vi "Beampointing.vi"() -> ()   [LabVIEW 2020]
uses:
  Ctrs/beam detection.ctl
  GUI_Beampointing_single_TRA/Ctrs/move.ctl
  Shared/GUI_Template/GUI_master/tcp_new_data_event.ctl
  Shared/GUI_Template/GUI_master/tcp new data cluster.ctl
  Ctrs/thresholds.ctl
  Ctrs/Detection all.ctl
  Ctrs/BP configuration.ctl
  General GUIs/Device GUIs/GUI_Cameras/Controls/Crosshair type def.ctl
  <userlib>/_OpenG.lib/array/array.llb/Filter 1D Array with Scalar (String)__ogtk.vi
  <userlib>/_OpenG.lib/array/array.llb/Sort 1D Array (DBL)__ogtk.vi
  <userlib>/_OpenG.lib/array/array.llb/Reorder 1D Array2 (Variant)__ogtk.vi
  <userlib>/_OpenG.lib/file/file.llb/File Exists - Scalar__ogtk.vi
  <userlib>/_OpenG.lib/array/array.llb/Remove Duplicates from 1D Array (String)__ogtk.vi
  <userlib>/_OpenG.lib/file/file.llb/Strip Path Extension - String__ogtk.vi
  <vilib>/Analysis/NI_AALBase.lvlib
  <vilib>/vision/NI_Vision_Development_Module.lvlib
  <vilib>/Utility/file.llb/Write To Spreadsheet File (string).vi
panel:
  in  "pixel calib":dbl
  out "A2y":dbl
  out "A1y":dbl
  out "A2x":dbl
  out "A1x":dbl
  in  "y'":dbl
  in  "x'":dbl
  in  "y":dbl
  in  "x":dbl
  in  "distance to target plane":dbl
  in  "seperation":dbl
  in  "downstream mirror":dbl
  in  "upstream mirror":dbl
  in  "Coupled Mirror Move":bool
  out "error out":errorcluster
  in  "active CCDs":i32(listbox)
  out "Prev State":string
  out "tcp data event 2":T1
  out "error out 3":errorcluster
  out "cam means":sgl[](array[numeric])
  in  "save path":path=path "W:/BP_DATA"
  out "millisecond timer value":u32
  out "motor refs 3":refnum<vi>[](array[refnum])
  in  "active man refs":cluster{"Ref X":refnum<vi>, "Ref Y":refnum<vi>}
  in  "#imgs avd so far":dbl
  out "Current State":string
  out "CCDs":string[](array[string])
  in  "GUIdevice 12":string
  in  "GUIdevice 11":string
  in  "GUIdevice 10":string
  in  "GUIdevice 9":string
  out "error out 2":errorcluster
  out "Names":string[](array[string])
  out "Box":T2(array[cluster])
  in  "Tab Cams":T3(tab)=enum."Main"
  in  "Cameras and motors":T4(array[cluster]) {"Motor Alias Y" items=["SHG-angle", "compensation-plate-x", "compensation-plate-y", "Stage [um]", "grating angle", "AttenuatorWavelplate", "Delay", "micrometer", "rail position", "Amp3 North", "djjdjd", "drive grating 2 trans", "speed_translation", "speed_rot_grating2", "speed_rot_grating1", "drive grating 2 rot", "drive grating 1 rot", "jet x", "jet y", "jet z", "ESP2_1_blade", "ESP2_2_target rotation", "home1", "ESP2_3_Scatter ST4 Move", "ESP3_3_mode z position", "com", "ESP3_1_Scatter_Mirror_Z", "ESP3_2", "ESP6_1_scatter ST4 x/hor", "ESP6_2_scatter ST4 y/vert", "ESP6_3_scatter mode z", "VISA", "S1C1 x", "S1C1 y", "S1C1 z", "S1C2 x", "S1C2 y", "S1C2 z", "S1C3 x", "S1C3 y", "S1C3 z", "S1C4 x", "S1C4 y", "S1C4 z", "S2C1 x", "S2C1 y", "S2C1 z", "S2C2 x", "S2C2 y", "S2C2 z", "S2C3 x", "S2C3 y", "S2C3 z", "S2C4 x", "S2C4 y", "S2C4 z", "S3C1 x", "S3C1 y", "S3C1 z", "S3C2 x", "S3C2 y", "S3C2 z", "S3C3 x", "S3C3 y", "S3C3 z", "S3C4 x", "S3C4 y", "S3C4 z", "S4C1 x", "S4C1y", "S4C1 z", "S4C2 x", "S4C2 y", "S4C2 z", "S4C3 x", "S4C3 y", "S4C3 z", "S4C4 x", "S4C4 y", "S4C4 z", "S5C1 x", "S5C1 y", "S5C1 z", "S5C2 x", "S5C2 y", "S5C2 z", "S5C3 x", "S5C3 y", "S5C3 z", "S5C4 x", "S5C4 y", "S5C4 z", "S1C1", "S1C2", "S1C3", "S1C4", "S2C1", "S2C2", "S2C3", "S2C4", "S3C1", "S3C2", "S3C3", "S3C4", "S4C1", "S4C2", "S4C3", "S4C4", "S5C1", "S5C2", "S5C3", "S5C4", "Stepsize 1", "Stepsize 2", "Stepsize 3", "VISA", "S1C1", "S1C2", "S1C3", "S1C4", "S2C1", "S2C2", "S2C3", "S2C4", "S3C1", "S3C2", "S3C3", "S3C4", "S4C1", "S4C2", "S4C3", "S4C4", "S5C1", "S5C2", "S5C3", "S5C4", "kHz EC wedge", "Fiber Mode", "XH2", "ND6", "XH4", "d-scan wedge", "EC wedge", "Lanex", "Gentec", "ModeImager", "Magnet", "ProbeDelay", "x position", "y position", "not working", "LaserDiodeX", "LaserDiodeY", "DelayStage (mm)", "Focus_Beam_2 (mm)", "Hex_x", "Hex_y", "Hex_z", "Hex_u", "Hex_v", "Hex_w", "Mode_Image_pos (mm)", "Jet X", "Jet Y", "Jet Z", "Amp2_out_Y", "Amp3_in_X", "Amp2_out_X", "Amp3_in_Y", "Amp4_in_X", "Amp4_in_Y", "Amp4_in_X", "Gaia2_South_Y", "Gaia3_South_X", "Gaia3_South_Y", "Gaia4_South_X", "Gaia4_South_Y", "Amp2_in_X", "Not Working", "Gaia3_North_X", "Gaia3_North_Y", "Gaia4_North_X", "Gaia4_North_Y", "Expanderin_1_X", "Expanderin_1_Y", "weak current", "Amp4_Out_Y", "Gaia2_North_X", "Gaia2_North_Y", "Amp4_out_X", "Amp2_in_Y", "Gaia2_South_X", "Stretcher_Out_X", "Not_Working", "Stretcher_Out_Y", "JetBladeHeight", "Probe far X", "Probe far Y", "Probe near X", "Probe near Y", "Seed in X", "Seed in Y", "Probe delay X", "Probe delay Y", "Seed Lens Z", "SeedWaveplateRot", "Broken", "SeedPrismBroken", "SeedPrismY", "SeedPrismX", "BCaveDiodeM2Horizontal", "BCaveDiodeM2Vertical", "BCaveDiodeM1Vertical", "BCaveDiodeM1Horizontal", "Grating separation (um)", "Grating1 angle", "Grating2 angle", "Jet_X (mm)", "Jet_Y (mm)", "Jet_Z (mm)", "Prepulse stage", "LegendCompressor (mm)", "devport", "ModeImager", "JetBlade", "ProbeDelay", "1", "TubeIn-x", "TubeIn-y", "CompIn-x", "CompIn-y", "stepSize", "Beamline_In-x", "Beamline_In-y", "Beamline_Out-y", "Beamline_Out-x", "OAPin2-x", "OAPin2-y", "Chassi IP", "BCaveIn-X", "BCaveIn-Y", "OAPIn1-X", "OAPIn1-Y", "DMSurface-X", "DMSurface-Y", "testzaber"]; "Motor Alias X" items=["SHG-angle", "compensation-plate-x", "compensation-plate-y", "Stage [um]", "grating angle", "AttenuatorWavelplate", "Delay", "micrometer", "rail position", "Amp3 North", "djjdjd", "drive grating 2 trans", "speed_translation", "speed_rot_grating2", "speed_rot_grating1", "drive grating 2 rot", "drive grating 1 rot", "jet x", "jet y", "jet z", "ESP2_1_blade", "ESP2_2_target rotation", "home1", "ESP2_3_Scatter ST4 Move", "ESP3_3_mode z position", "com", "ESP3_1_Scatter_Mirror_Z", "ESP3_2", "ESP6_1_scatter ST4 x/hor", "ESP6_2_scatter ST4 y/vert", "ESP6_3_scatter mode z", "VISA", "S1C1 x", "S1C1 y", "S1C1 z", "S1C2 x", "S1C2 y", "S1C2 z", "S1C3 x", "S1C3 y", "S1C3 z", "S1C4 x", "S1C4 y", "S1C4 z", "S2C1 x", "S2C1 y", "S2C1 z", "S2C2 x", "S2C2 y", "S2C2 z", "S2C3 x", "S2C3 y", "S2C3 z", "S2C4 x", "S2C4 y", "S2C4 z", "S3C1 x", "S3C1 y", "S3C1 z", "S3C2 x", "S3C2 y", "S3C2 z", "S3C3 x", "S3C3 y", "S3C3 z", "S3C4 x", "S3C4 y", "S3C4 z", "S4C1 x", "S4C1y", "S4C1 z", "S4C2 x", "S4C2 y", "S4C2 z", "S4C3 x", "S4C3 y", "S4C3 z", "S4C4 x", "S4C4 y", "S4C4 z", "S5C1 x", "S5C1 y", "S5C1 z", "S5C2 x", "S5C2 y", "S5C2 z", "S5C3 x", "S5C3 y", "S5C3 z", "S5C4 x", "S5C4 y", "S5C4 z", "S1C1", "S1C2", "S1C3", "S1C4", "S2C1", "S2C2", "S2C3", "S2C4", "S3C1", "S3C2", "S3C3", "S3C4", "S4C1", "S4C2", "S4C3", "S4C4", "S5C1", "S5C2", "S5C3", "S5C4", "Stepsize 1", "Stepsize 2", "Stepsize 3", "VISA", "S1C1", "S1C2", "S1C3", "S1C4", "S2C1", "S2C2", "S2C3", "S2C4", "S3C1", "S3C2", "S3C3", "S3C4", "S4C1", "S4C2", "S4C3", "S4C4", "S5C1", "S5C2", "S5C3", "S5C4", "kHz EC wedge", "Fiber Mode", "XH2", "ND6", "XH4", "d-scan wedge", "EC wedge", "Lanex", "Gentec", "ModeImager", "Magnet", "ProbeDelay", "x position", "y position", "not working", "LaserDiodeX", "LaserDiodeY", "DelayStage (mm)", "Focus_Beam_2 (mm)", "Hex_x", "Hex_y", "Hex_z", "Hex_u", "Hex_v", "Hex_w", "Mode_Image_pos (mm)", "Jet X", "Jet Y", "Jet Z", "Amp2_out_Y", "Amp3_in_X", "Amp2_out_X", "Amp3_in_Y", "Amp4_in_X", "Amp4_in_Y", "Amp4_in_X", "Gaia2_South_Y", "Gaia3_South_X", "Gaia3_South_Y", "Gaia4_South_X", "Gaia4_South_Y", "Amp2_in_X", "Not Working", "Gaia3_North_X", "Gaia3_North_Y", "Gaia4_North_X", "Gaia4_North_Y", "Expanderin_1_X", "Expanderin_1_Y", "weak current", "Amp4_Out_Y", "Gaia2_North_X", "Gaia2_North_Y", "Amp4_out_X", "Amp2_in_Y", "Gaia2_South_X", "Stretcher_Out_X", "Not_Working", "Stretcher_Out_Y", "JetBladeHeight", "Probe far X", "Probe far Y", "Probe near X", "Probe near Y", "Seed in X", "Seed in Y", "Probe delay X", "Probe delay Y", "Seed Lens Z", "SeedWaveplateRot", "Broken", "SeedPrismBroken", "SeedPrismY", "SeedPrismX", "BCaveDiodeM2Horizontal", "BCaveDiodeM2Vertical", "BCaveDiodeM1Vertical", "BCaveDiodeM1Horizontal", "Grating separation (um)", "Grating1 angle", "Grating2 angle", "Jet_X (mm)", "Jet_Y (mm)", "Jet_Z (mm)", "Prepulse stage", "LegendCompressor (mm)", "devport", "ModeImager", "JetBlade", "ProbeDelay", "1", "TubeIn-x", "TubeIn-y", "CompIn-x", "CompIn-y", "stepSize", "Beamline_In-x", "Beamline_In-y", "Beamline_Out-y", "Beamline_Out-x", "OAPin2-x", "OAPin2-y", "Chassi IP", "BCaveIn-X", "BCaveIn-Y", "OAPIn1-X", "OAPIn1-Y", "DMSurface-X", "DMSurface-Y", "testzaber"]}
  in  "tdms root":path=path "c:/BP_DATAsd"
  out "get pos time":u32
  out "config path":string
  out "tolerances (pix)":dbl[](array[numeric])
  in  "device ini":bool
  in  "Exposure:12":dbl=0.095 min=0.0001 max=1.0 format="%#_6f"
  in  "Triggerdelay::12":dbl=0.003 min=0.0 max=0.09 format="%#_6f"
  in  "Exposure::11":dbl=0.095 min=0.0001 max=1.0 format="%#_6f"
  in  "Triggerdelay::11":dbl=0.003 min=0.0 max=0.09 format="%#_6f"
  in  "Exposure::10":dbl=0.095 min=0.0001 max=1.0 format="%#_6f"
  in  "Triggerdelay::10":dbl=0.003 min=0.0 max=0.09 format="%#_6f"
  in  "Exposure::9":dbl=0.095 min=0.0001 max=1.0 format="%#_6f"
  in  "Triggerdelay::9":dbl=0.003 min=0.0 max=0.09 format="%#_6f"
  in  "Trigger::9":bool
  in  "Trigger::10":bool caption="Trigger:10"
  in  "Trigger::11":bool
  in  "Trigger::12":bool
  in  "Target.Y::9":dbl=45.0 caption="T9y" min=0.0 max=2000.0 format="%#_6f"
  in  "Target.X::9":dbl=47.0 caption="Tx9" min=0.0 max=2000.0 format="%#_6f"
  in  "Target.Y::10":dbl=45.0 caption="T10y" min=0.0 max=2000.0 format="%#_6f"
  in  "Target.X::10":dbl=47.0 caption="T10x" min=0.0 max=2000.0 format="%#_6f"
  in  "Target.Y::11":dbl=45.0 caption="T11y" min=0.0 max=2000.0 format="%#_6f"
  in  "Target.X::11":dbl=47.0 caption="T11x" min=0.0 max=2000.0 format="%#_6f"
  in  "Target.Y::12":dbl=45.0 caption="T12y" min=0.0 max=2000.0 format="%#_6f"
  in  "Target.X::12":dbl=47.0 caption="T12x" min=0.0 max=2000.0 format="%#_6f"
  in  "Exposure::8":dbl=0.095 min=3.8e-05 max=1.0 format="%#_6f"
  in  "Triggerdelay::8":dbl=0.003 min=0.0 max=0.09 format="%#_6f"
  in  "Trigger::8":bool
  in  "Target.Y::8":dbl=45.0 caption="T8y" min=0.0 max=2000.0 format="%#_6f"
  in  "Target.X::8":dbl=47.0 caption="T8x" min=0.0 max=2000.0 format="%#_6f"
  in  "Target.Y::7":dbl=45.0 caption="T7x" min=0.0 max=2000.0 format="%#_6f"
  in  "Target.X::7":dbl=47.0 caption="T7y" min=0.0 max=2000.0 format="%#_6f"
  in  "Target.Y::6":dbl=45.0 caption="T6y" min=0.0 max=2000.0 format="%#_6f"
  in  "Target.X::6":dbl=47.0 caption="T6x" min=0.0 max=2000.0 format="%#_6f"
  in  "Target.Y::5":dbl=45.0 caption="T5y" min=0.0 max=2000.0 format="%#_6f"
  in  "Target.X::5":dbl=47.0 caption="T5x" min=0.0 max=2000.0 format="%#_6f"
  in  "Target.Y::4":dbl=45.0 caption="T4y" min=0.0 max=2000.0 format="%#_6f"
  in  "Target.X::4":dbl=47.0 caption="T4x" min=0.0 max=2000.0 format="%#_6f"
  in  "Target.Y::3":dbl=163.0 caption="T3y" min=0.0 max=2000.0 format="%#_6f"
  in  "Target.X::3":dbl=152.0 caption="T3x" min=0.0 max=2000.0 format="%#_6f"
  in  "Target.Y::2":dbl=74.0 caption="T2y" min=0.0 max=2000.0 format="%#_6f"
  in  "Target.X::2":dbl=75.0 caption="T2x" min=0.0 max=2000.0 format="%#_6f"
  in  "Target.Y::1":dbl=61.0 caption="T1y" min=0.0 max=2000.0 format="%#_6f"
  in  "Target.X::1":dbl=77.0 caption="T1x" min=0.0 max=2000.0 format="%#_6f"
  in  "Exposure::7":dbl=0.095 min=3.8e-05 max=1.0 format="%#_6f"
  in  "Triggerdelay::7":dbl=0.003 min=0.0 max=0.09 format="%#_6f"
  in  "Trigger::7":bool
  in  "Exposure::6":dbl=0.095 min=0.0001 max=1.0 format="%#_6f"
  in  "Triggerdelay::6":dbl=0.003 min=1.0 max=900000.0 format="%#_6f"
  in  "Trigger::6":bool
  in  "Exposure::5":dbl=0.095 min=0.0001 max=1.0 format="%#_6f"
  in  "Triggerdelay::5":dbl=0.003 min=0.0 max=100000.0 format="%#_6f"
  in  "Trigger::5":bool
  in  "Exposure::4":dbl=0.095 min=10.0 max=1000000.0 format="%#_6f"
  in  "Triggerdelay::4":dbl=0.003 min=10.0 max=1000000.0 format="%#_6f"
  in  "Trigger::4":bool
  in  "Exposure::3":dbl=0.095 min=5e-05 max=1.0 format="%#_6f"
  in  "Triggerdelay::3":dbl=0.003 min=10.0 max=500000.0 format="%#_6f"
  in  "Trigger::3":bool
  in  "Exposure::2":dbl=0.095 min=1e-05 max=1.0 format="%#_6f"
  in  "Triggerdelay::2":dbl=0.003 min=10.0 max=100000.0 format="%#_6f"
  in  "Trigger::2":bool
  out "image::1":T5(plugin-control) caption="UC_TubeIn"
  out "image::2":T5(plugin-control) caption="UC_GratingMode"
  out "image::3":T5(plugin-control) caption="UC_DMSurface"
  out "image::4":T5(plugin-control) caption="UC_BCaveIn"
  out "image::5":T5(plugin-control) caption="UC_OAPin1"
  out "image::6":T5(plugin-control) caption="UC_OAPin2"
  out "image::7":T5(plugin-control)
  out "image::8":T5(plugin-control)
  in  "Exposure::1":dbl=0.095 min=50.0 max=500000.0 format="%#_6f"
  in  "Triggerdelay::1":dbl=0.003 min=0.01 max=999000.0 format="%#_6f"
  in  "Trigger::1":bool
  in  "UDP error message":string
  out "required Y":bool[](array[boolean])
  out "required X":bool[](array[boolean])
  out "detected":bool[](array[boolean])
  out "name array":string[](array[string])
  out "image::9":T5(plugin-control)
  out "image::10":T5(plugin-control)
  out "image::11":T5(plugin-control)
  out "image::12":T5(plugin-control)
  out "CCD 1":cluster{timestamp[], dbl[]}[](graph)
  in  "History Size":i32=500
  out "History Index":i32
  in  "Cam# history":i32
  out "Moving X":string
  out "Moving Y":string
  in  "centroidy::4":dbl=45.0 caption="T4y" min=0.0 max=0.0 format="%#_6f"
  in  "centroidx::4":dbl=47.0 caption="T4x" min=0.0 max=0.0 format="%#_6f"
  in  "centroidy::3":dbl=163.0 caption="T3y" min=0.0 max=0.0 format="%#_6f"
  in  "centroidx::3":dbl=152.0 caption="T3x" min=0.0 max=0.0 format="%#_6f"
  in  "centroidy::2":dbl=74.0 caption="T2y" min=0.0 max=0.0 format="%#_6f"
  in  "centroidx::2":dbl=75.0 caption="T2x" min=0.0 max=0.0 format="%#_6f"
  in  "centroidy::1":dbl=61.0 caption="T1y" min=0.0 max=0.0 format="%#_6f"
  in  "centroidx::1":dbl=77.0 caption="T1x" min=0.0 max=0.0 format="%#_6f"
  in  "centroidy::8":dbl=45.0 caption="T8y" min=0.0 max=0.0 format="%#_6f"
  in  "centroidx::8":dbl=47.0 caption="T8x" min=0.0 max=0.0 format="%#_6f"
  in  "centroidy::7":dbl=45.0 caption="T7x" min=0.0 max=0.0 format="%#_6f"
  in  "centroidx::7":dbl=47.0 caption="T7y" min=0.0 max=0.0 format="%#_6f"
  in  "centroidy::6":dbl=45.0 caption="T6y" min=0.0 max=0.0 format="%#_6f"
  in  "centroidx::6":dbl=47.0 caption="T6x" min=0.0 max=0.0 format="%#_6f"
  in  "centroidy::5":dbl=45.0 caption="T5y" min=0.0 max=0.0 format="%#_6f"
  in  "centroidx::5":dbl=47.0 caption="T5x" min=0.0 max=0.0 format="%#_6f"
  in  "centroidy::12":dbl=45.0 caption="T12y" min=0.0 max=2000.0 format="%#_6f"
  in  "centroidx::12":dbl=47.0 caption="T12x" min=0.0 max=2000.0 format="%#_6f"
  in  "centroidy::11":dbl=45.0 caption="T11y" min=0.0 max=2000.0 format="%#_6f"
  in  "centroidx::11":dbl=47.0 caption="T11x" min=0.0 max=2000.0 format="%#_6f"
  in  "centroidy::10":dbl=45.0 caption="T10y" min=0.0 max=2000.0 format="%#_6f"
  in  "centroidx::10":dbl=47.0 caption="T10x" min=0.0 max=2000.0 format="%#_6f"
  in  "centroidy::9":dbl=45.0 caption="T9y" min=0.0 max=2000.0 format="%#_6f"
  in  "centroidx::9":dbl=47.0 caption="Tx9" min=0.0 max=2000.0 format="%#_6f"
  out "active ccd particles":T6(array[cluster])
  in  "Speedmode":dbl=5.0 min=1.0 max=20.0
  out "all UDP in motor config good":bool
  in  "Feedback Global":bool
  in  "GUIdevice 8":string
  in  "Tab Control":T7(tab)
  in  "alarms":bool
  in  "new tdms":bool
  in  "Save Stats":bool
  in  "Save Config":bool
  in  "Load Config":bool
  in  "update speed [ms]":i32=2000 min=1000 max=10000
  in  "img to avg":i32=15 min=3 max=200
  in  "Reset History":bool
  in  "autodetect":bool
  in  "Detection Rate":dbl=0.9 min=0.001 max=1.0
  in  "Center":bool
  in  "Align":bool
  in  "average centroid":bool
  in  "clear error":bool
  in  "thresholds":T8
  in  "beam detection para":T9={"Filter"=1, "Filter Para"={"X Size"=5, "Y Size"=5, "% Tolerance"=1}, "detection method"=4, "Particle filtering"=[{"Measurement Parameter"=35, "Range Lower Value"=0.0, "Range Upper Value"=500.0, "Range"=FALSE, "Measurement Type"=FALSE}], "Remove small Objects"=TRUE, "Restrict to round Objects"=FALSE, "Use Cam COM"=FALSE} {"Particle filtering"."Measurement Parameter" items=["Center of Mass X", "Center of Mass Y", "First Pixel X", "First Pixel Y", "Bounding Rect Left", "Bounding Rect Top", "Bounding Rect Right", "Bounding Rect Bottom", "Max Feret Diameter Start X", "Max Feret Diameter Start Y", "Max Feret Diameter End X", "Max Feret Diameter End Y", "Max Horiz. Segment Length Left", "Max Horiz. Segment Length Right", "Max Horiz. Segment Length Row", "-", "Bounding Rect Width", "Bounding Rect Height", "Bounding Rect Diagonal", "Perimeter", "Convex Hull Perimeter", "Holes' Perimeter", "Max Feret Diameter", "Equivalent Ellipse Major Axis", "Equivalent Ellipse Minor Axis", "Equivalent Ellipse Minor Axis (Feret)", "Equivalent Rect Long Side", "Equivalent Rect Short Side", "Equivalent Rect Diagonal", "Equivalent Rect Short Side (Feret)", "Average Horiz. Segment Length", "Average Vert. Segment Length", "Hydraulic Radius", "Waddel Disk Diameter", "-", "Area", "Holes' Area", "Particle & Holes' Area", "Convex Hull Area", "Image Area", "-", "Number of Holes", "Number of Horiz. Segments", "Number of Vert. Segments", "-", "Orientation", "Max Feret Diameter Orientation", "-", "% Area/Image Area", "% Area/(Particle & Holes' Area)", "Ratio of Equivalent Ellipse Axes", "Ratio of Equivalent Rect Sides", "-", "Elongation Factor", "Compactness Factor", "Heywood Circularity Factor", "Type Factor", "-", "Sum X", "Sum Y", "Sum XX", "Sum XY", "Sum YY", "Sum XXX", "Sum XXY", "Sum XYY", "Sum YYY", "-", "Moment of Inertia XX", "Moment of Inertia XY", "Moment of Inertia YY", "Moment of Inertia XXX", "Moment of Inertia XXY", "Moment of Inertia XYY", "Moment of Inertia YYY", "Norm. Moment of Inertia XX", "Norm. Moment of Inertia XY", "Norm. Moment of Inertia YY", "Norm. Moment of Inertia XXX", "Norm. Moment of Inertia XXY", "Norm. Moment of Inertia XYY", "Norm. Moment of Inertia YYY", "Hu Moment 1", "Hu Moment 2", "Hu Moment 3", "Hu Moment 4", "Hu Moment 5", "Hu Moment 6", "Hu Moment 7"]; "Particle filtering"."Range Lower Value" format="%.2f"; "Particle filtering"."Range Upper Value" format="%.2f"; "detection method" items=["clustering", "entropy", "metric", "moments", "inter-class variance"]; "Filter" items=["No Filter", "Median Filter", "Low Pass Filter"]}
  out "Active CCD":string
  in  "move config":T11={"Tolerance [%]"=0.1, "Stepsize"=0.0001, "Invert Direction X"=FALSE, "Invert Direction Y"=TRUE, "enable feedback"=FALSE, "Set Centriod Target"=FALSE, "xCal"=0.0001, "xCal neg"=0.0001, "yCal"=0.0001, "yCal neg"=0.0001}
  in  "Position 2":dbl=0.001 caption="Stepsize" min=0.0 max=999999.0 format="%_6f"
  in  "Position 1":dbl=0.001 caption="Stepsize" min=0.0 max=999999.0 format="%_6f"
  in  "Right":bool caption="RelativeMove.Axis 1.CCW::1"
  in  "Left":bool caption="RelativeMove.Axis 1.CW::1"
  in  "Down":bool caption="RelativeMove.Axis. 2.CCW::1"
  in  "Up":bool caption="RelativeMove.Axis 2.CW::1"
  in  "StepSize":dbl=0.01 caption="Stepsize" min=0.0 max=1.0 step=0.001 format="%#_6p"
  in  "Time":timestamp[][](array[timestamp])
  in  "Offset X":dbl[][](array[numeric])
  in  "Mean Centroid X":dbl[][](array[numeric])
  in  "GUIdevice 7":string
  in  "GUIdevice 6":string
  in  "GUIdevice 5":string
  in  "GUIdevice 4":string
  in  "GUIdevice 3":string="TargetCam10Hz_Diode"
  in  "GUIdevice 2":string="StagingM1Far"
  in  "insert tag":bool=TRUE
  in  "stop":bool
  in  "GUIdevice 1":string="StagingM1Near"
  out "error IO 2":errorcluster
  # "code in progess for coupled mirror move: please don't delete (Sam)"
  # "Motor axes must have aliases"
  # "Save config after changing cams/motors"
  # "max"
  # "When running for the first time\nCancel the load configuration\nSet the Camera and motors in the config tab\nSave the configuration\nLoad the configuration\nConfigure the detection and feedback for each camera\nSave the configuration\n\nTips\nIn detection, you can exclude or include particles. Typically, include based on the area of the particle.\nYou can either use the particle centroid, or the center of mass calculated in the camera\nFor the case of camera COM, it will only use it if it is in the bounding box of the detected particle.\nA calibration is critical for good performance. Use MC to perform a motor scan and perform a linear fit of COM vs motor position in x and y. Put the gradients into xCal and yCal.\nStep size in move config no longer used.\nFor motors (like LTAs), set the backlash and set it to default in MC. Backlash amount is retrieved from a positive and negative motor scan, and reading the position distance between the lines of the graph of COM vs motor position.\nUnder system tab, update speed must be > than slowest camera update. Otherwise program will find the slow cam/s not having a new image, and it will perform a new configuration."
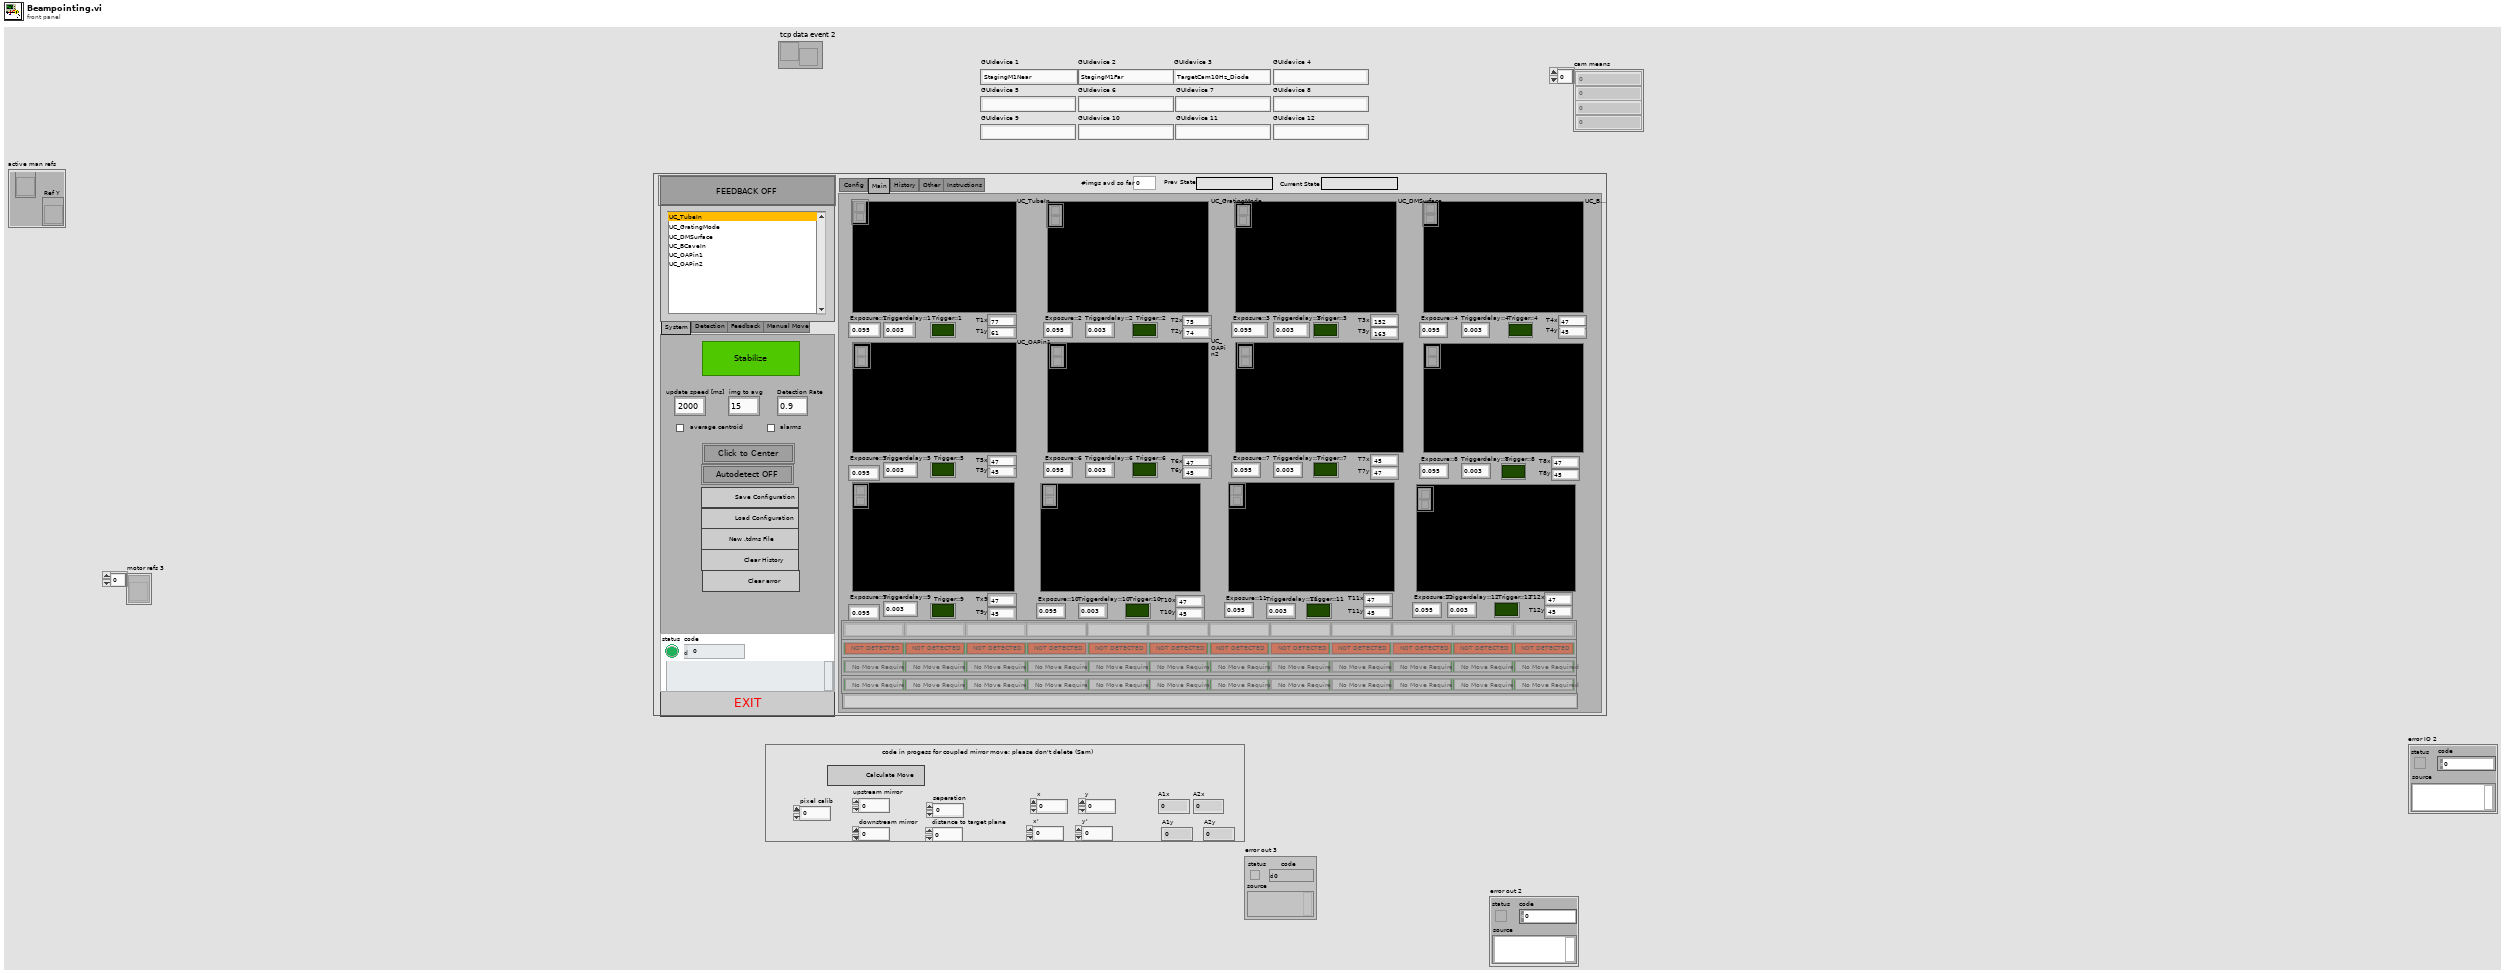
[diagram p1: front panel]
types:
  T1 = typedef "tcp_new_data_event.ctl" = refnum<user-event>
  T2 = cluster{"Left":dbl, "Top":dbl, "Right":dbl, "Bottom":dbl}[]
  T3 = enum32{"Config ", "Main", "History", "Other", "Instructions"}
  T4 = cluster{"Camera":string, "Motor Alias X":u16, "Motor Alias Y":u16}[]
  T5 = typedef "IMAQ Image.ctl" = refnum<image>
  T6 = cluster{"Area":dbl, "Number of Holes":dbl, "Bounding Rect":cluster{"Left":dbl, "Top":dbl, "Right":dbl, "Bottom":dbl}, "Center of Mass":cluster{"X":dbl, "Y":dbl}, "Orientation":dbl, "Dimensions":cluster{"Width":dbl, "Height":dbl}}[]
  T7 = enum32{"System", "Detection", "Feedback", "Manual Move"}
  T8 = typedef "thresholds.ctl" = cluster{"Lower value":sgl, "Upper value":sgl}
  T9 = typedef "beam detection.ctl" = cluster{"Filter":u16, "Filter Para":cluster{"X Size":i32, "Y Size":i32, "% Tolerance":i32}, "detection method":i32, "Particle filtering":cluster{"Measurement Parameter":T10, "Range Lower Value":dbl, "Range Upper Value":dbl, "Range":bool, "Measurement Type":bool}[], "Remove small Objects":bool, "Restrict to round Objects":bool, "Use Cam COM":bool}
  T10 = typedef "Particle Parameters" = i32
  T11 = typedef "move.ctl" = cluster{"Tolerance [%]":dbl, "Stepsize":dbl, "Invert Direction X":bool, "Invert Direction Y":bool, "enable feedback":bool, "Set Centriod Target":bool, "xCal":dbl, "xCal neg":dbl, "yCal":dbl, "yCal neg":dbl}
  T12 = cluster{"Target.X::1":refnum<vi>, "Target.Y::1":refnum<vi>}
  T13 = cluster{"Target.X::2":refnum<vi>, "Target.Y::2":refnum<vi>}
  T14 = cluster{"Target.X::3":refnum<vi>, "Target.Y::3":refnum<vi>}
  T15 = cluster{"Target.X::4":refnum<vi>, "Target.Y::4":refnum<vi>}
  T16 = cluster{"Target.X::5":refnum<vi>, "Target.Y::5":refnum<vi>}
  T17 = cluster{"Target.X::6":refnum<vi>, "Target.Y::6":refnum<vi>}
  T18 = cluster{"Target.X::7":refnum<vi>, "Target.Y::7":refnum<vi>}
  T19 = cluster{"Target.X::8":refnum<vi>, "Target.Y::8":refnum<vi>}
  T20 = cluster{"Target.X::12":refnum<vi>, "Target.Y::12":refnum<vi>}
  T21 = cluster{"Target.X::9":refnum<vi>, "Target.Y::9":refnum<vi>}
  T22 = cluster{"Target.X::10":refnum<vi>, "Target.Y::10":refnum<vi>}
  T23 = cluster{"Target.X::11":refnum<vi>, "Target.Y::11":refnum<vi>}
  T24 = cluster{"Target.X::12":refnum<vi>, "Target.Y::12":refnum<vi>}[]
  T25 = enum32{"invalid app kind", "Development System", "Run Time System", "Student Edition", "Embedded LabVIEW", "Evaluation", "Custom"}
  T26 = enum32{"Invalid", "Standard", "Closed", "Hidden", "Minimized", "Maximized"}
  T27 = typedef "BP configuration.ctl" = cluster{"Camera names":string[], "Motor aliases x":string[], "Motor aliases y":string[], "detection para":T9[], "thresholds":cluster{"Lower value":sgl, "Upper value":sgl}[], "move properties":T11[], "tdms root":path}
  T28 = typedef "tcp new data cluster.ctl" = cluster{"EventEnum":enum16{"new data", "connection status update"}, "Device name":string}
  T29 = enum16{"open", "replace", "create", "open or create", "replace or create", "replace or create with confirmation"}
  T30 = enum8{"Enabled", "Disabled", "Disabled and Grayed Out"}
  T31 = enum16{"open", "open or create", "create or replace", "create", "open (read-only)"}
  T32 = typedef "Detection all.ctl" = cluster{"detection para":T9[], "thresholds":cluster{"Lower value":sgl, "Upper value":sgl}[], "Centroid X":dbl[][], "Centroid Y":dbl[][], "Size":dbl[][], "Centroid refs":cluster{"centroidx::12":refnum<vi>, "centroidy::12":refnum<vi>}[], "img to avg":i32}
  T33 = cluster{"detection para":T9[], "thresholds":cluster{"Lower value":sgl, "Upper value":sgl}[], "Centroid X":dbl[][], "Centroid Y":dbl[][], "Size":dbl[][], "Centroid refs":cluster{"centroidx::12":refnum<vi>, "centroidy::12":refnum<vi>}[], "img to avg":i32}
  T34 = cluster{"Area":dbl, "Number of Holes":dbl, "Bounding Rect":cluster{"Left":dbl, "Top":dbl, "Right":dbl, "Bottom":dbl}, "Center of Mass":cluster{"X":dbl, "Y":dbl}, "Orientation":dbl, "Dimensions":cluster{"Width":dbl, "Height":dbl}}[][]
  T35 = cluster{"Core":cluster{"Current VI Reference":refnum<vi>, "Close Panel on Exit?":bool}, "Detection":T32, "Mean Centroid X":dbl[][], "Mean Centroid Y":dbl[][], "Offset X":dbl[][], "Offset Y":dbl[][], "Offset X stats ":dbl[][], "Offset Y stats ":dbl[][], "Mean Size":dbl[][], "Time":timestamp[][], "move properties":T11[], "active axis refs 2":cluster{"Ref X":refnum<vi>, "Ref Y":refnum<vi>}[], "active ccd":i32, "Feedback global":bool, "Motor X":dbl[][], "Motor Y":dbl[][], "active cams":string[], "tdms ref":refnum<k34>, "active man refs":cluster{"Ref X":refnum<vi>, "Ref Y":refnum<vi>}, "detected":bool[], "speedmode X":bool[], "speedmode Y":bool[], "steps speed X":dbl[], "steps speed Y":dbl[], "Supergui":cluster{"STOP queue":refnum<queue>, "SuperGUI ref":refnum<vi>}, "dev var alias arrays":cluster{"dev variable alias":string[][], "dev variable alias Motors X":string[][], "dev variable alias Motors Y":string[][]}, "Motor positions":cluster{"Positions x":dbl[], "Positions y":dbl[]}, "Config loaded":bool}
  T36 = cluster{"Positions x":dbl[], "Positions y":dbl[]}
  T37 = cluster{"dev variable alias":string[][], "dev variable alias Motors X":string[][], "dev variable alias Motors Y":string[][]}
  T38 = cluster{"Ref X":refnum<vi>, "Ref Y":refnum<vi>}[]
  T39 = cluster{"STOP queue":refnum<queue>, "SuperGUI ref":refnum<vi>}
  T40 = cluster{"Current VI Reference":refnum<vi>, "Close Panel on Exit?":bool}
  T41 = cluster{"centroidx::1":refnum<vi>, "centroidy::1":refnum<vi>}
  T42 = cluster{"centroidx::2":refnum<vi>, "centroidy::2":refnum<vi>}
  T43 = cluster{"centroidx::3":refnum<vi>, "centroidy::3":refnum<vi>}
  T44 = cluster{"centroidx::4":refnum<vi>, "centroidy::4":refnum<vi>}
  T45 = cluster{"centroidx::5":refnum<vi>, "centroidy::5":refnum<vi>}
  T46 = cluster{"centroidx::6":refnum<vi>, "centroidy::6":refnum<vi>}
  T47 = cluster{"centroidx::7":refnum<vi>, "centroidy::7":refnum<vi>}
  T48 = cluster{"centroidx::8":refnum<vi>, "centroidy::8":refnum<vi>}
  T49 = cluster{"centroidx::12":refnum<vi>, "centroidy::12":refnum<vi>}
  T50 = cluster{"centroidx::9":refnum<vi>, "centroidy::9":refnum<vi>}
  T51 = cluster{"centroidx::10":refnum<vi>, "centroidy::10":refnum<vi>}
  T52 = cluster{"centroidx::11":refnum<vi>, "centroidy::11":refnum<vi>}
  T53 = cluster{"centroidx::12":refnum<vi>, "centroidy::12":refnum<vi>}[]
  T54 = cluster{"Camera":string, "Motor Alias X":u16, "Motor Alias Y":u16}
  T55 = typedef "Image Type" = u32
  T56 = cluster{"appended array":timestamp[], "appended array":dbl[]}
  T57 = cluster{"appended array":timestamp[], "appended array":dbl[]}[]
  T58 = typedef "Crosshair type def.ctl" = cluster{"Draw":bool, "Target":cluster{"x":dbl, "y":dbl}, "Size":cluster{"x":dbl, "y":dbl}, "Angle":dbl, "Color":u32, "Thickness":u8, "CrosshairLabel":string}
  T59 = cluster{"Left":i32, "Top":i32, "Right":i32, "Bottom":i32}
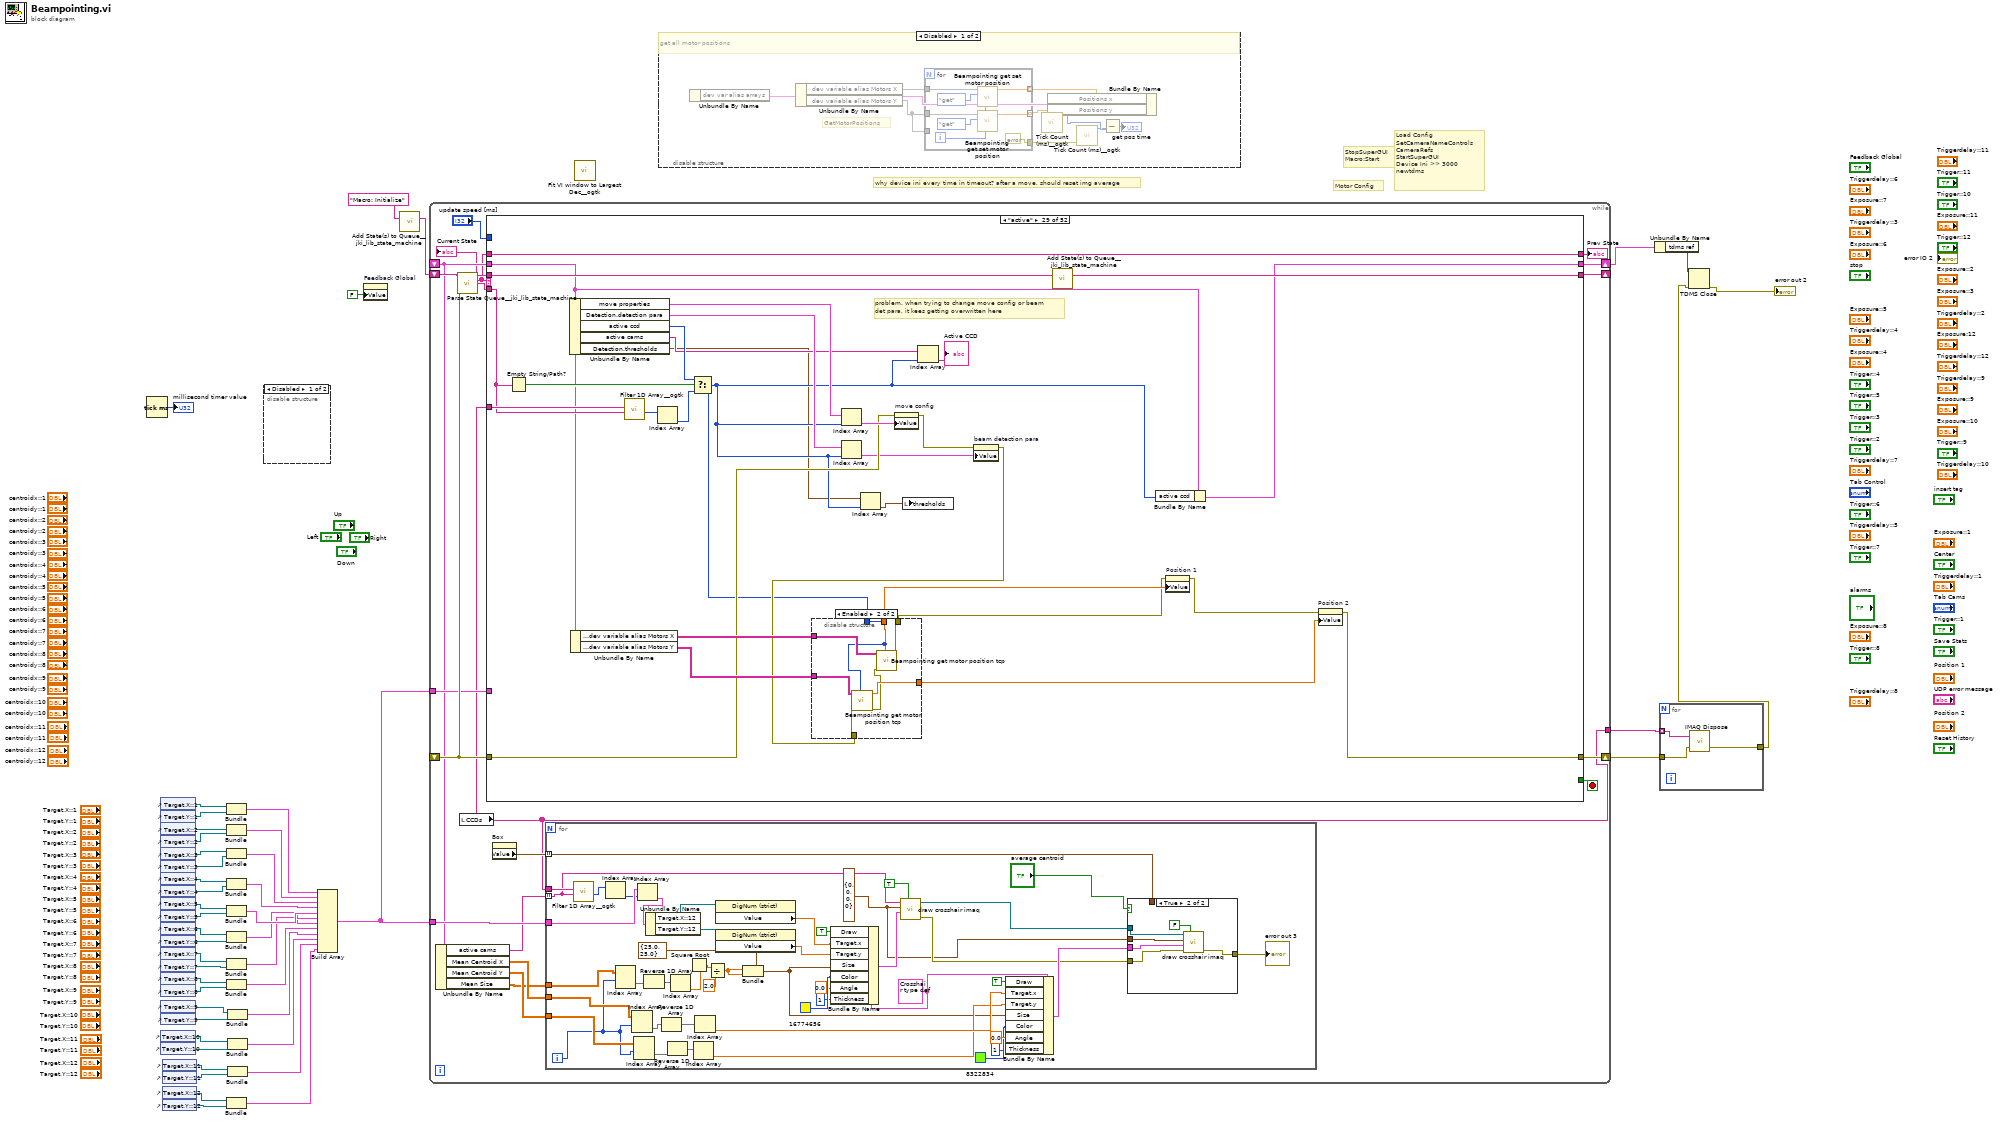
[diagram p0: block diagram]
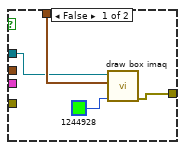
[diagram p4: hidden frame]
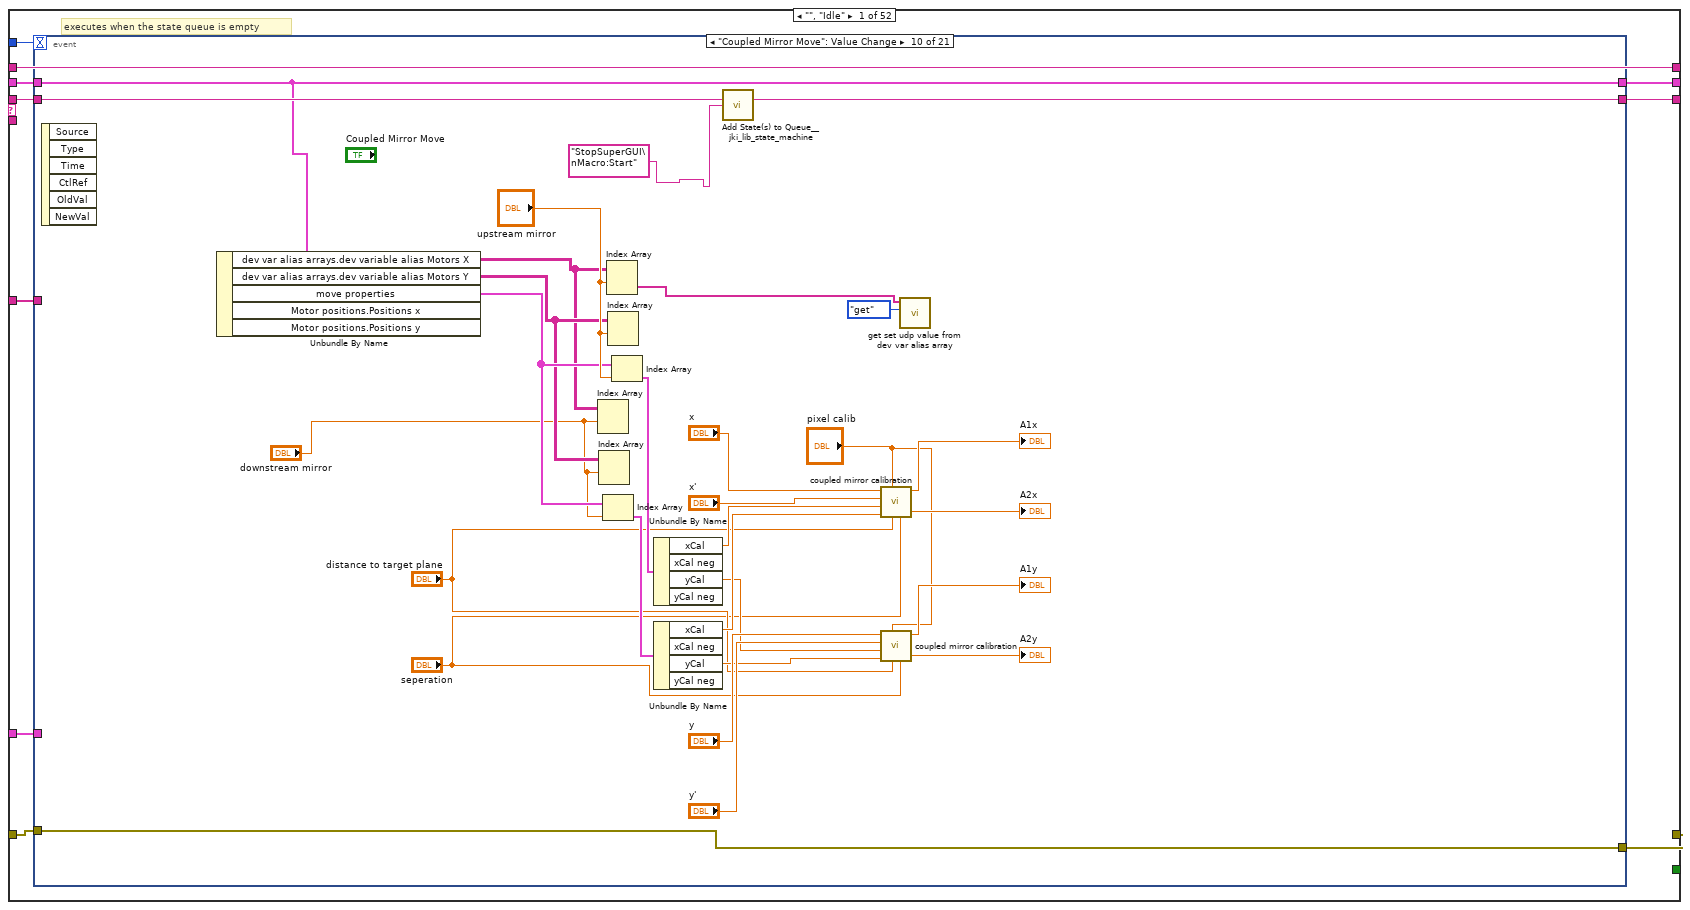
[diagram p5: hidden frame]
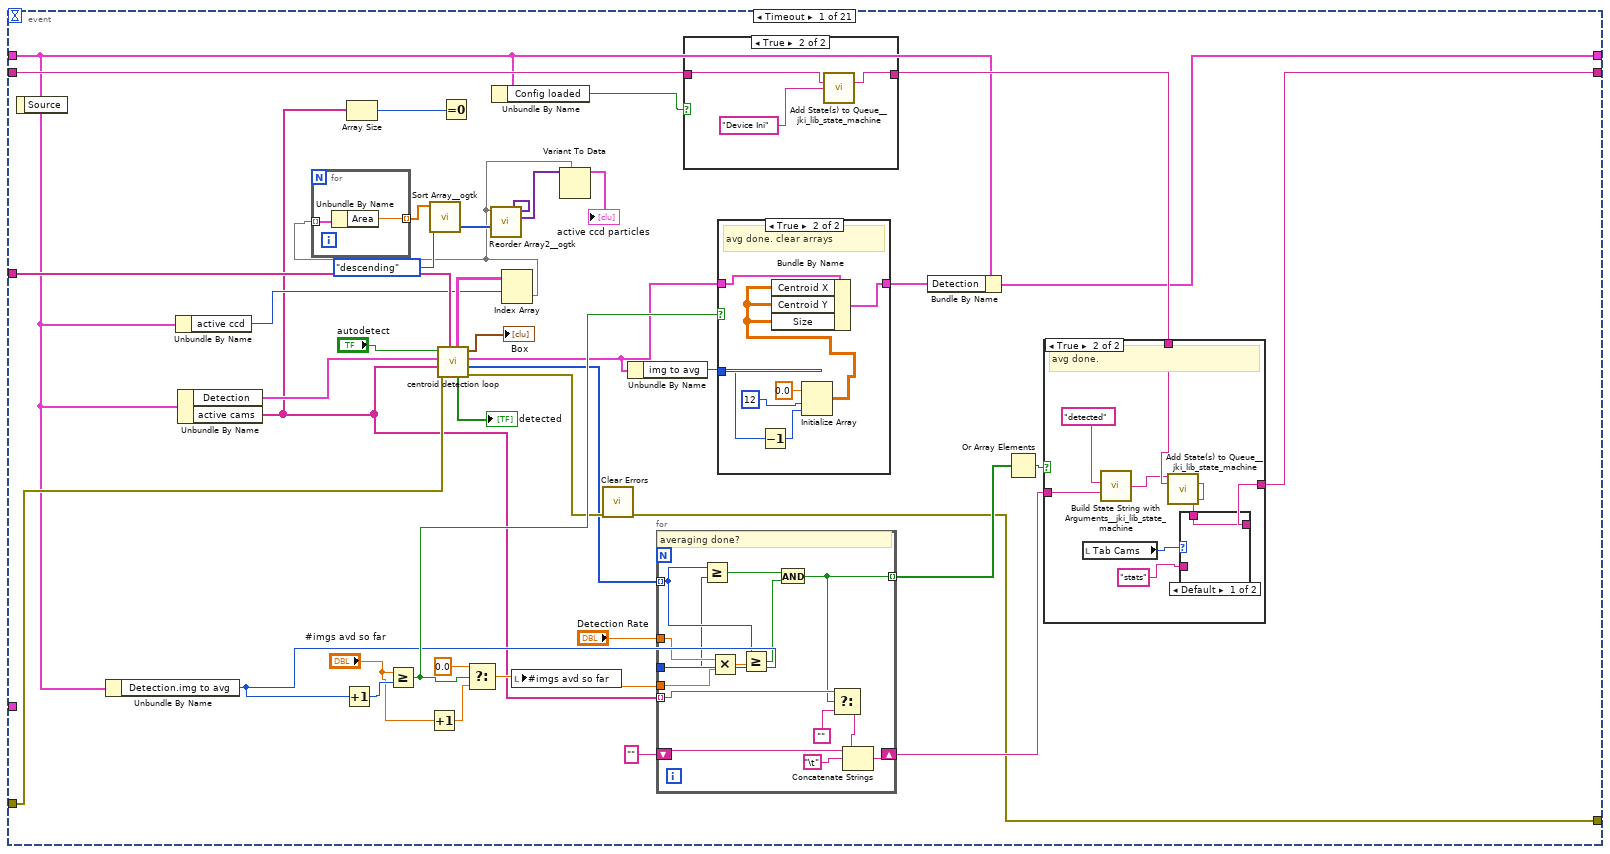
[diagram p6: hidden frame]
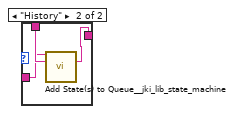
[diagram p10: hidden frame]
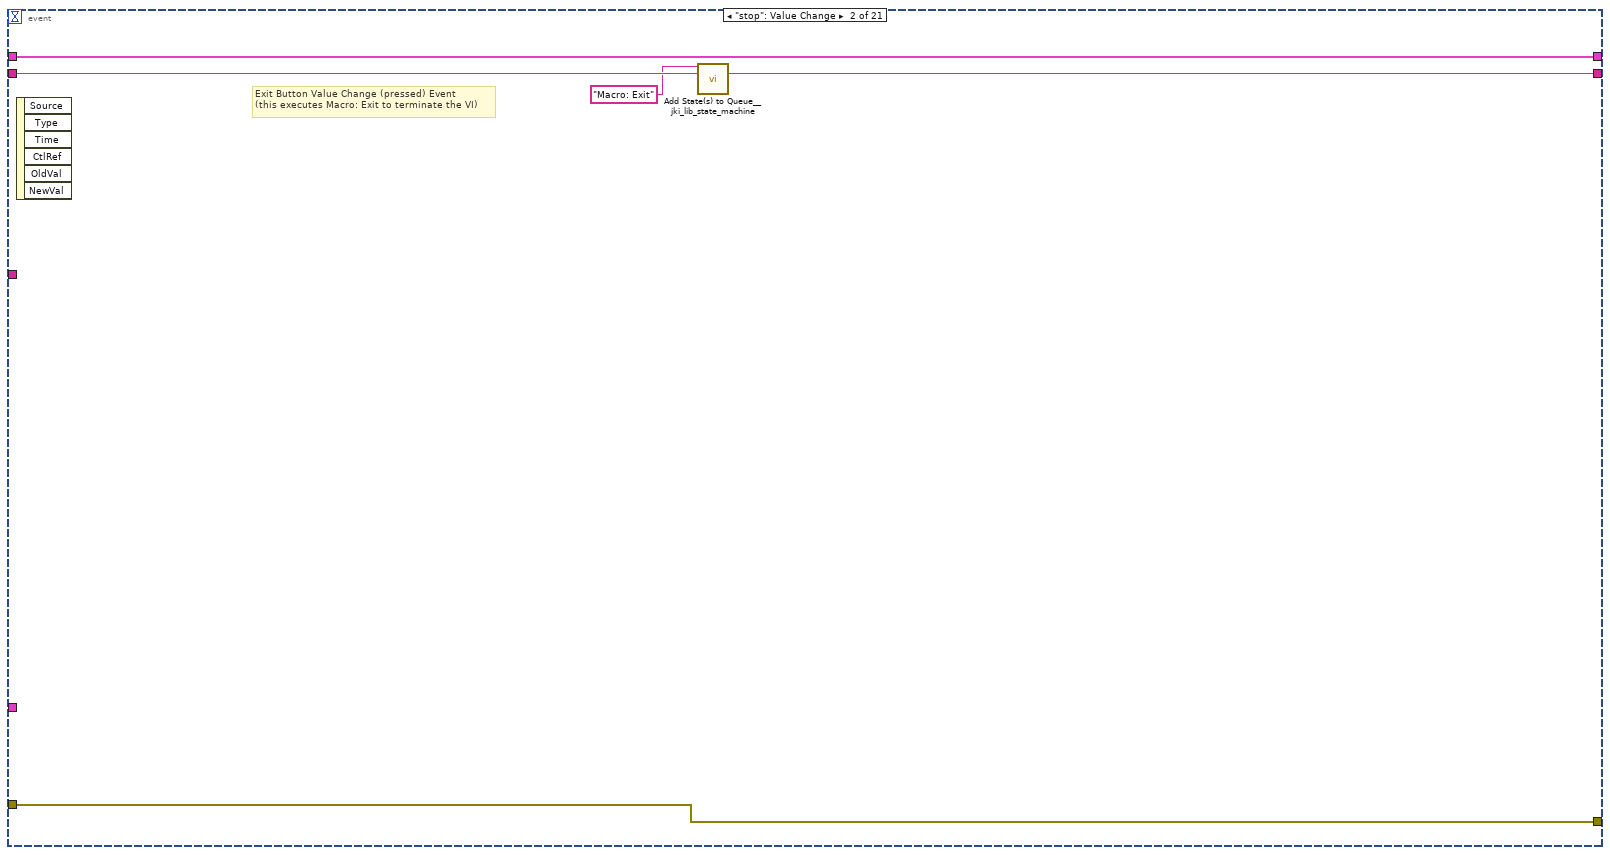
[diagram p11: hidden frame]
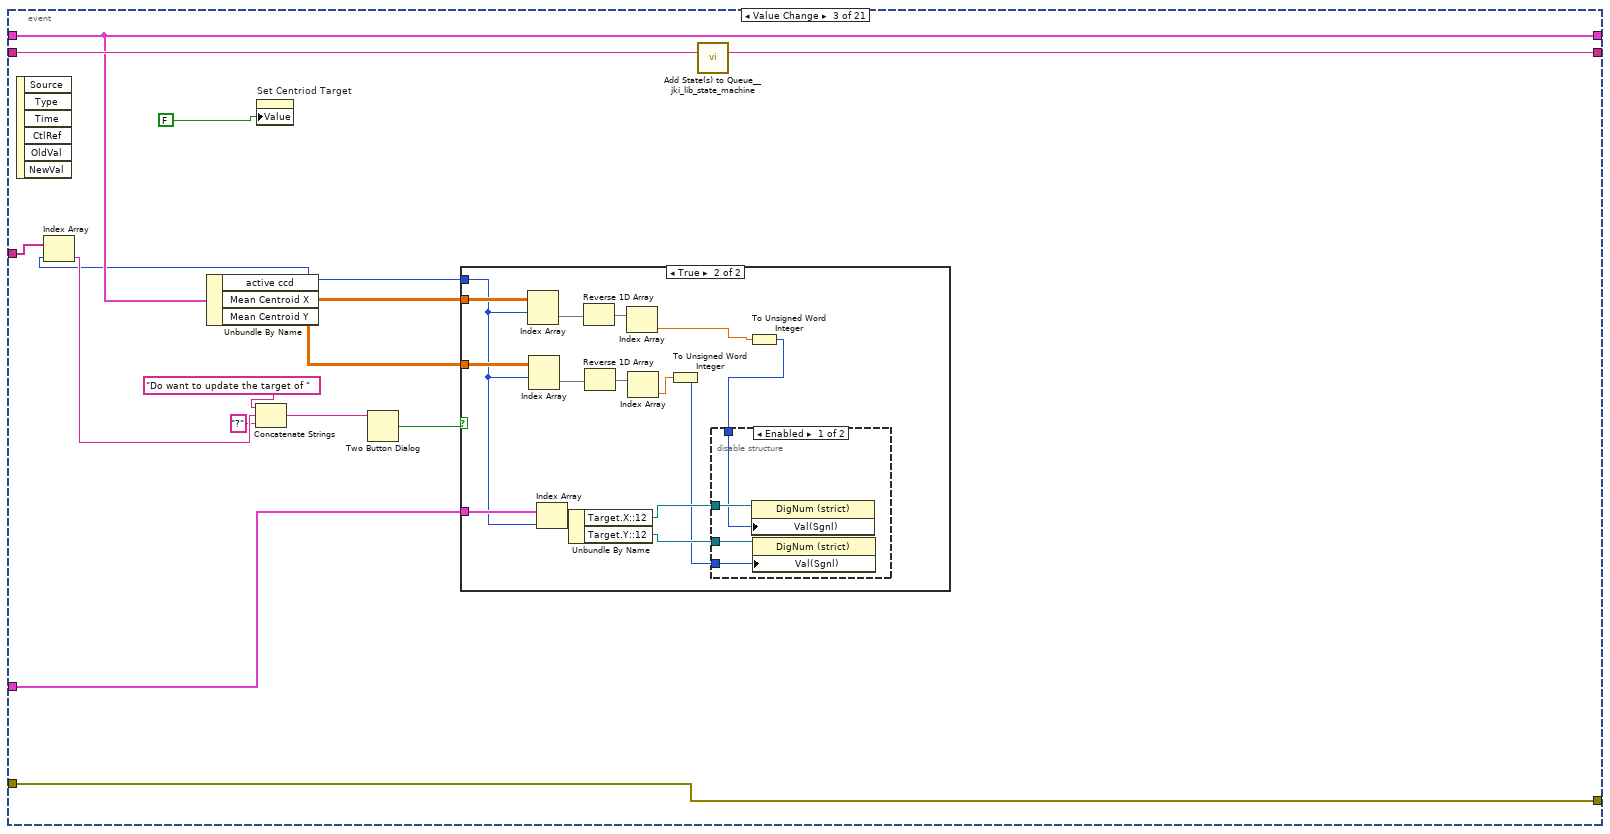
[diagram p12: hidden frame]
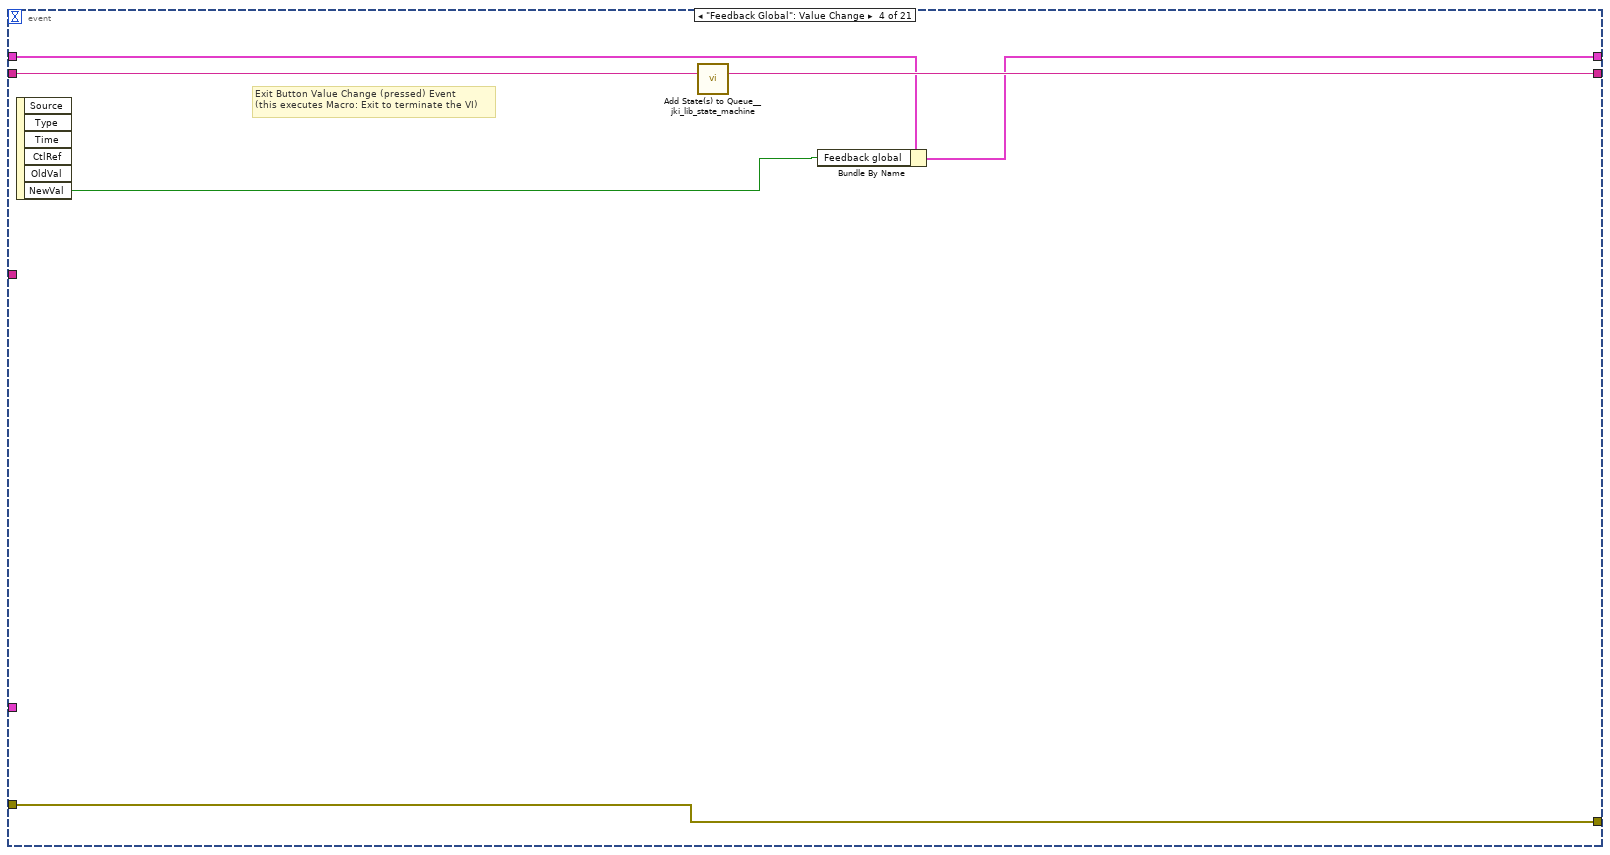
[diagram p15: hidden frame]
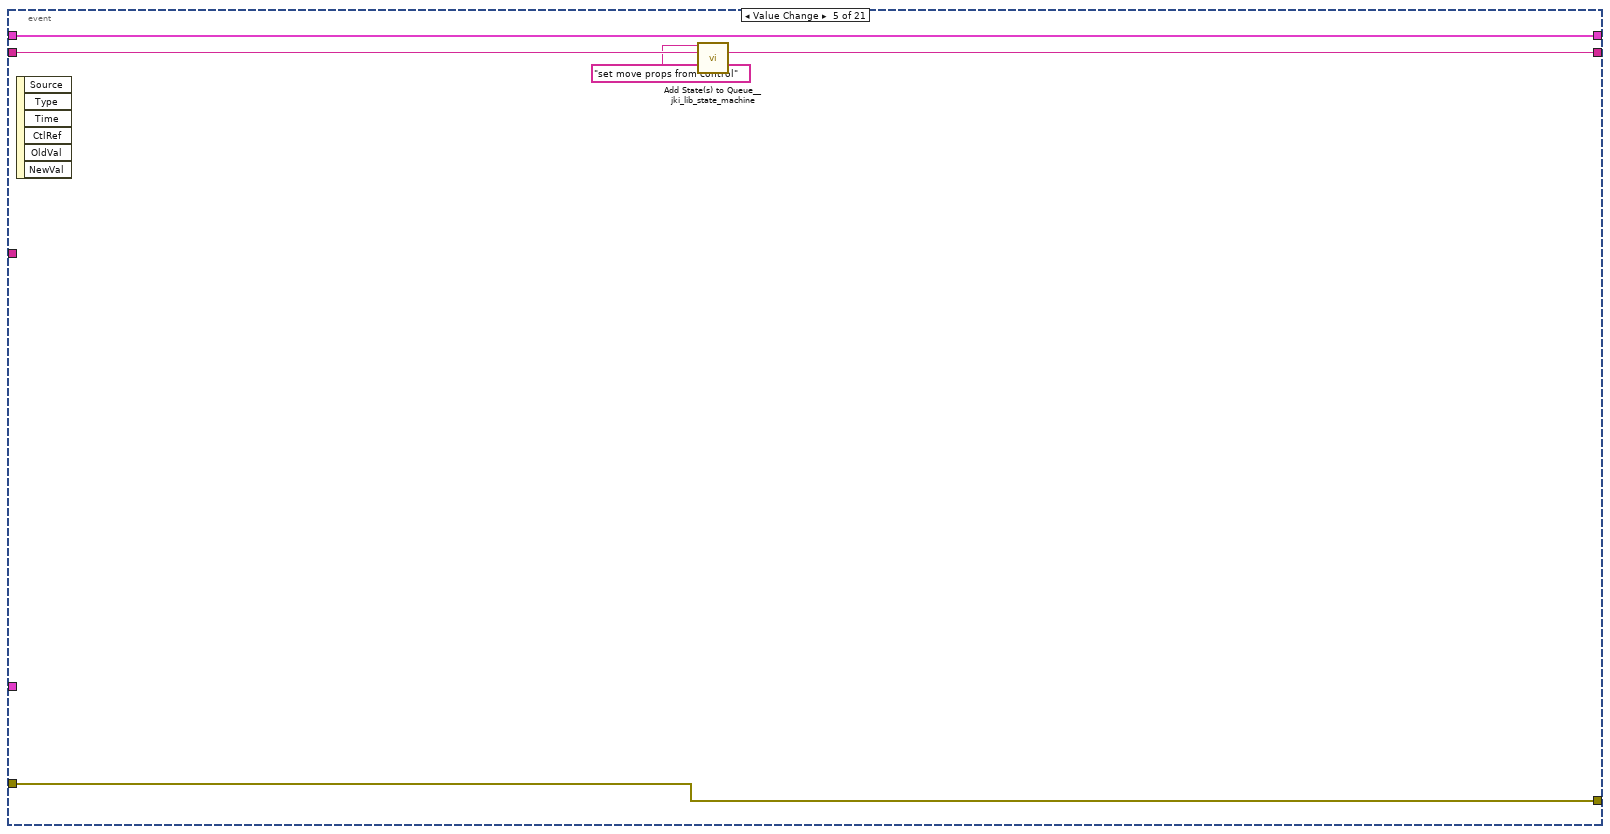
[diagram p16: hidden frame]
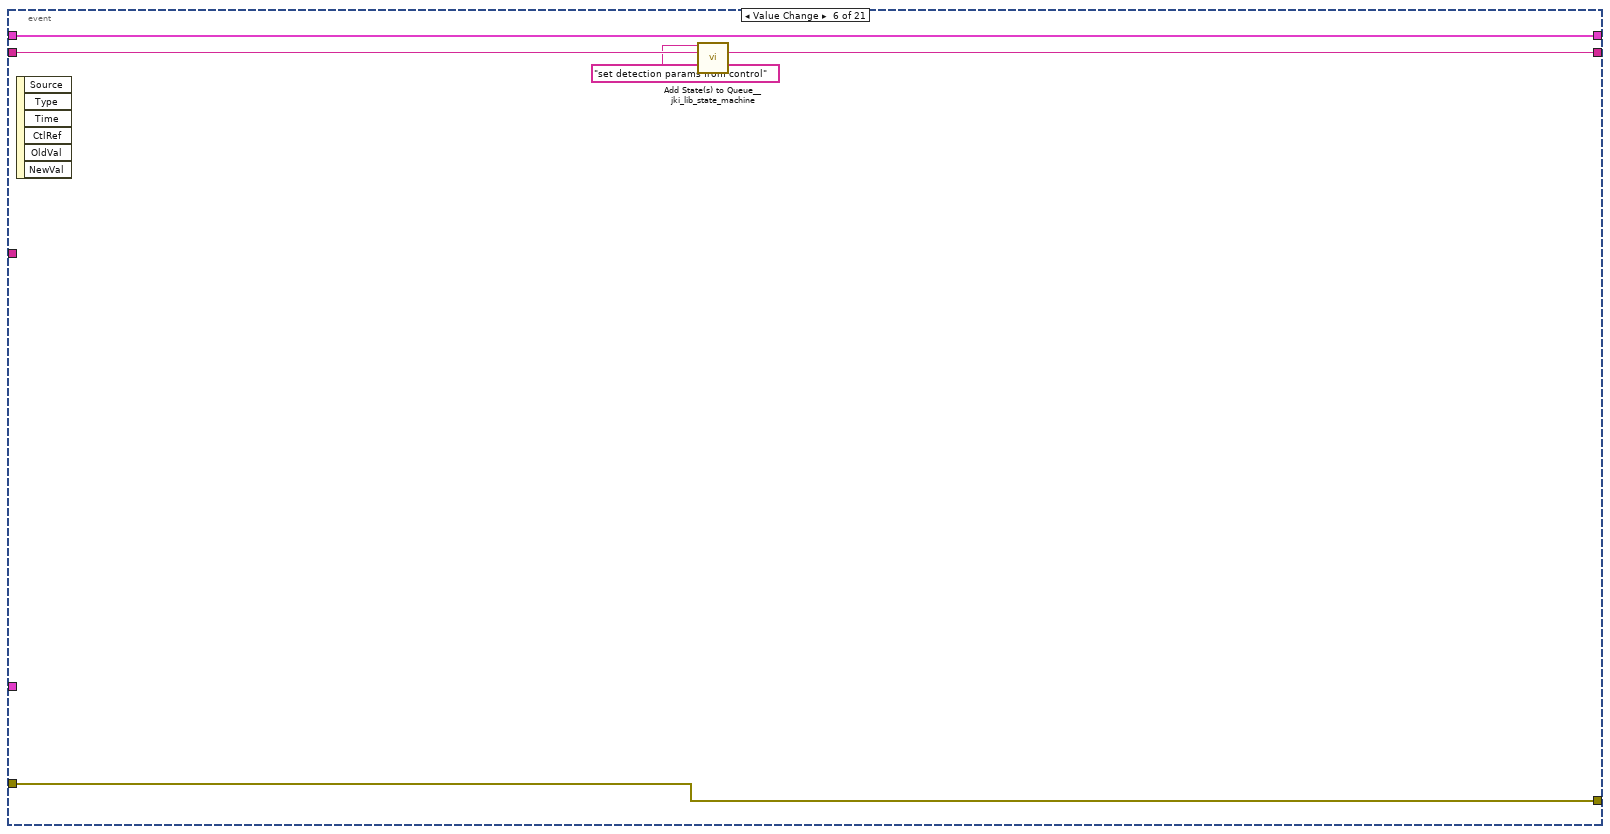
[diagram p17: hidden frame]
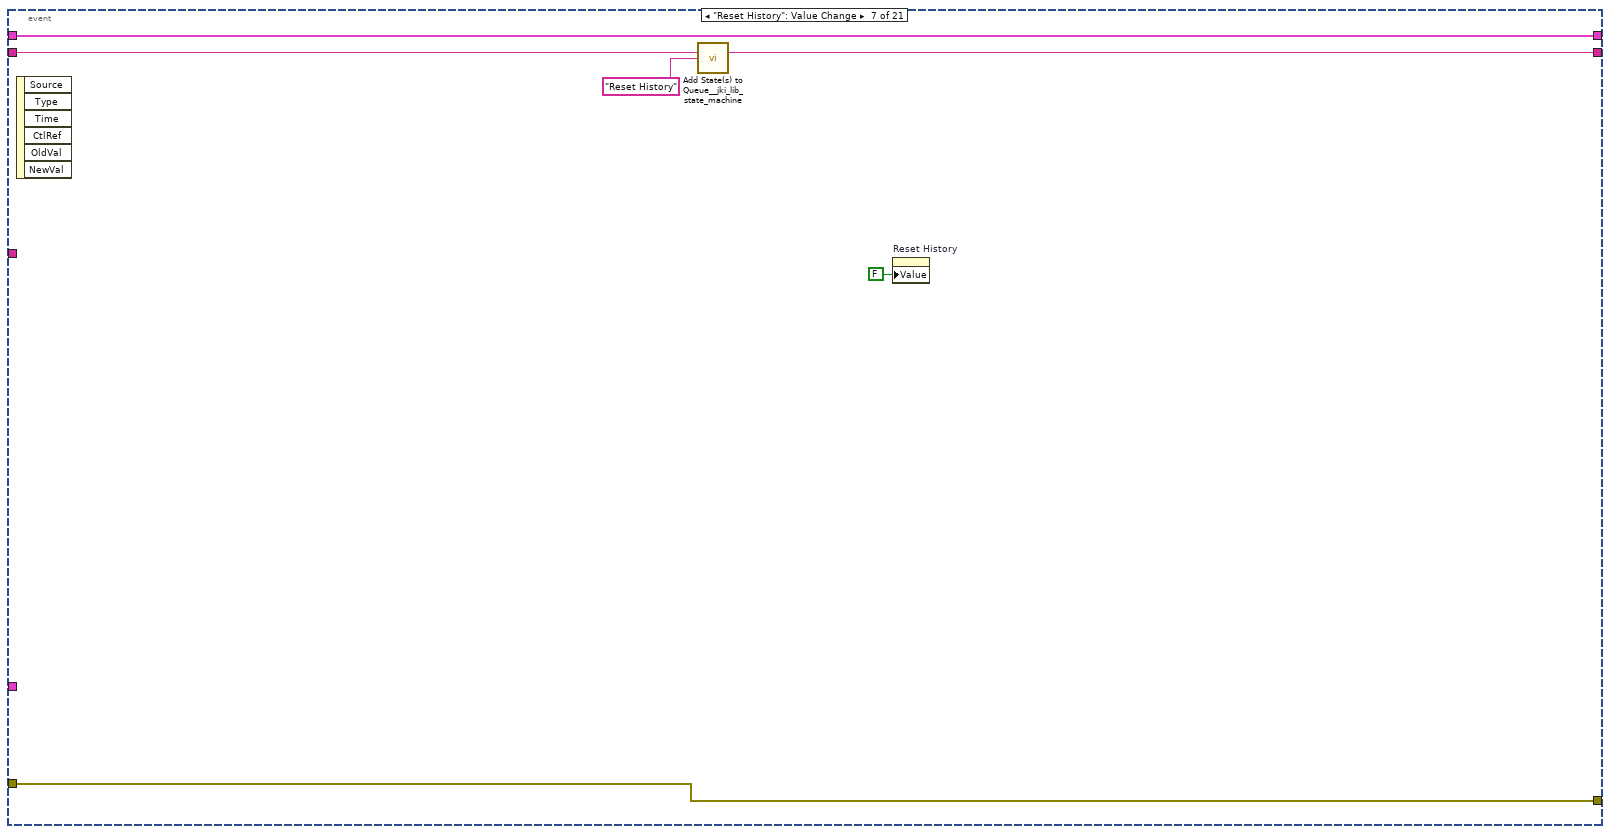
[diagram p18: hidden frame]
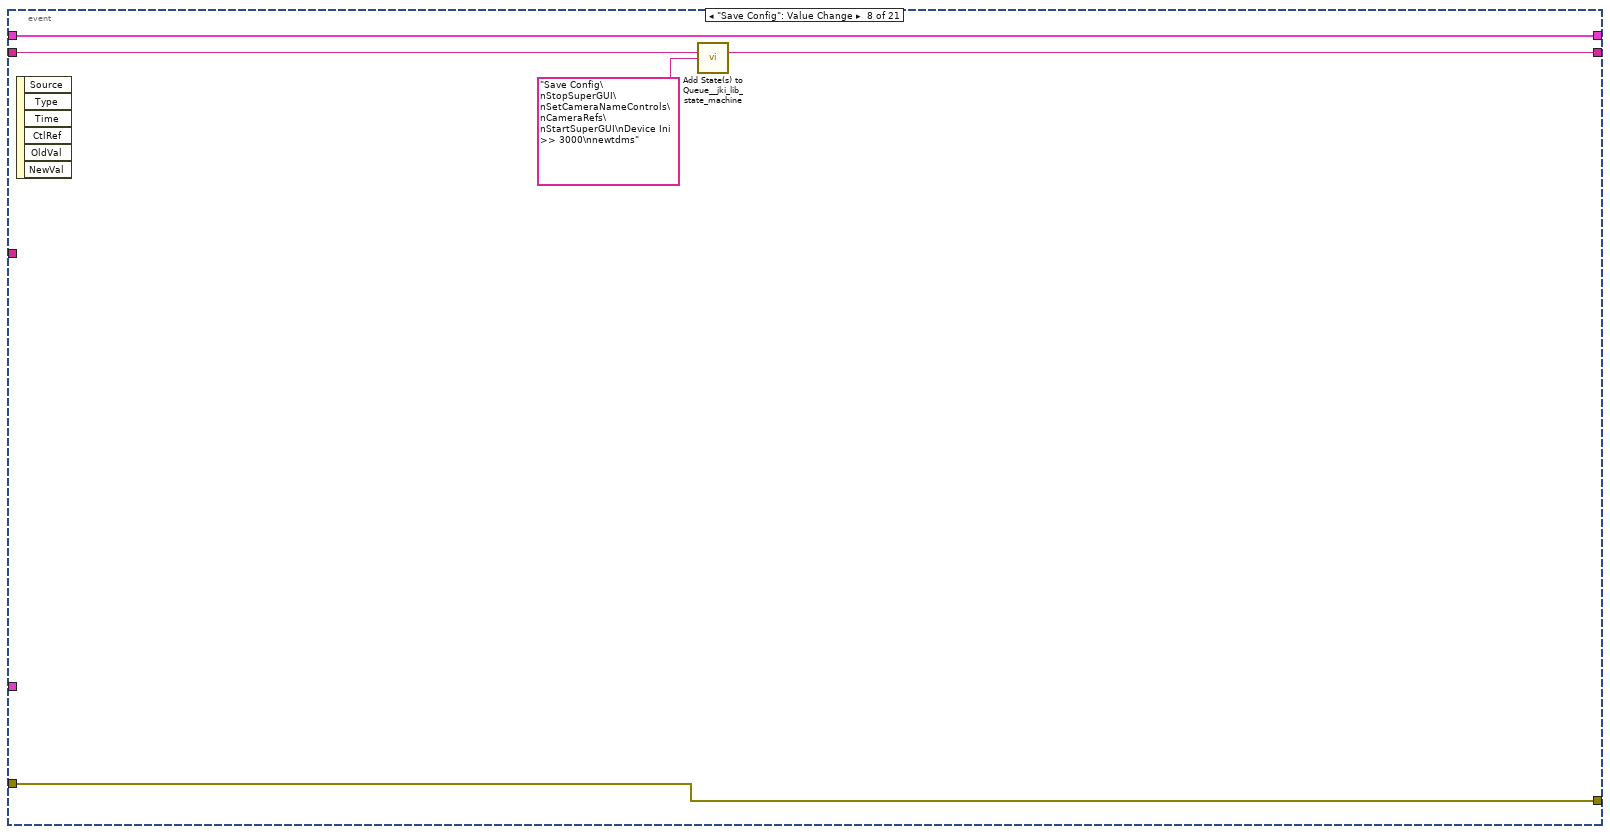
[diagram p19: hidden frame]
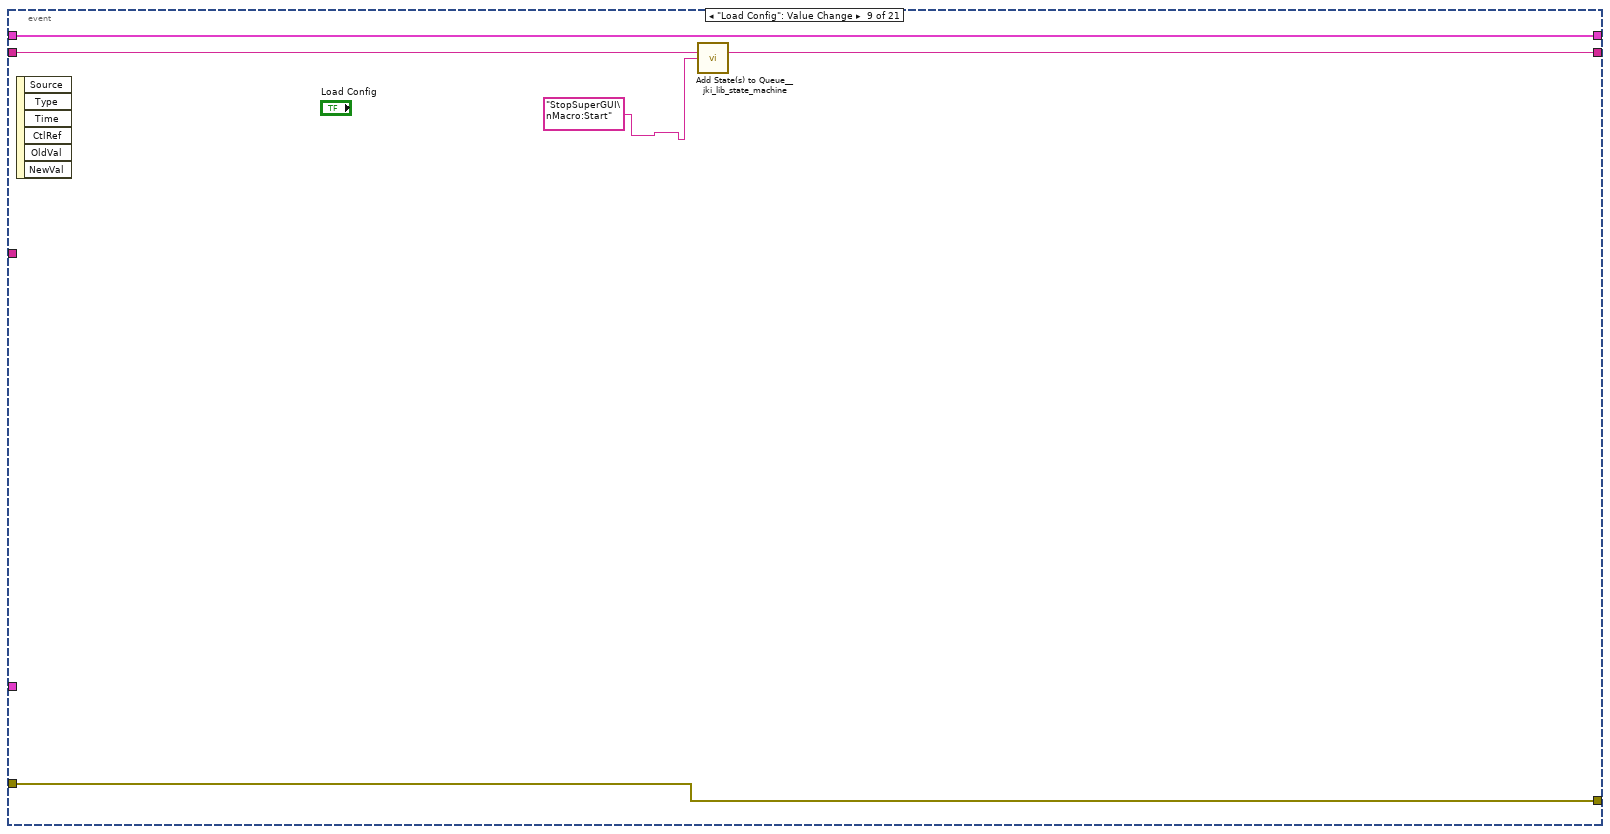
[diagram p20: hidden frame]
diagram:
  # "Motor Config"
  # "Load Config\nSetCameraNameControls\nCameraRefs\nStartSuperGUI\nDevice Ini >> 3000\nnewtdms"
  # "StopSuperGUI\nMacro:Start"
  # "why device ini every time in timeout? after a move, should reset img average"
  n1 = Tick Count (ms)() -> (millisecond timer value=→"millisecond timer value":u32)
  n2 = control-ref of="Target.X::1"() -> (w43:refnum<vi>)
  n3 = control-ref of="Target.Y::1"() -> (w42:refnum<vi>)
  n4 = control-ref of="Target.X::2"() -> (w41:refnum<vi>)
  n5 = control-ref of="Target.Y::2"() -> (w40:refnum<vi>)
  n6 = control-ref of="Target.X::3"() -> (w39:refnum<vi>)
  n7 = control-ref of="Target.Y::3"() -> (w38:refnum<vi>)
  n8 = control-ref of="Target.X::4"() -> (w37:refnum<vi>)
  n9 = control-ref of="Target.Y::4"() -> (w36:refnum<vi>)
  n10 = control-ref of="Target.X::5"() -> (w35:refnum<vi>)
  n11 = control-ref of="Target.Y::5"() -> (w34:refnum<vi>)
  n12 = control-ref of="Target.X::6"() -> (w33:refnum<vi>)
  n13 = control-ref of="Target.Y::6"() -> (w32:refnum<vi>)
  n14 = control-ref of="Target.X::7"() -> (w31:refnum<vi>)
  n15 = control-ref of="Target.Y::7"() -> (w30:refnum<vi>)
  n16 = control-ref of="Target.X::8"() -> (w29:refnum<vi>)
  n17 = control-ref of="Target.Y::8"() -> (w28:refnum<vi>)
  n18 = control-ref of="Target.X::9"() -> (w14:refnum<vi>)
  n19 = control-ref of="Target.Y::9"() -> (w13:refnum<vi>)
  n20 = control-ref of="Target.X::10"() -> (w12:refnum<vi>)
  n21 = control-ref of="Target.Y::10"() -> (w11:refnum<vi>)
  n22 = control-ref of="Target.X::11"() -> (w10:refnum<vi>)
  n23 = control-ref of="Target.Y::11"() -> (w9:refnum<vi>)
  n24 = control-ref of="Target.X::12"() -> (w8:refnum<vi>)
  n25 = control-ref of="Target.Y::12"() -> (w7:refnum<vi>)
  n26 = Bundle("Target.X::1"=w43, "Target.Y::1"=w42) -> (w27:T12)  [unwired: 1 in]
  n27 = Bundle("Target.X::2"=w41, "Target.Y::2"=w40) -> (w26:T13)  [unwired: 1 in]
  n28 = Bundle("Target.X::3"=w39, "Target.Y::3"=w38) -> (w25:T14)  [unwired: 1 in]
  n29 = Bundle("Target.X::4"=w37, "Target.Y::4"=w36) -> (w18:T15)  [unwired: 1 in]
  n30 = Bundle("Target.X::5"=w35, "Target.Y::5"=w34) -> (w24:T16)  [unwired: 1 in]
  n31 = Bundle("Target.X::6"=w33, "Target.Y::6"=w32) -> (w23:T17)  [unwired: 1 in]
  n32 = Bundle("Target.X::7"=w31, "Target.Y::7"=w30) -> (w22:T18)  [unwired: 1 in]
  n33 = Bundle("Target.X::8"=w29, "Target.Y::8"=w28) -> (w21:T19)  [unwired: 1 in]
  n34 = Bundle("Target.X::12"=w8, "Target.Y::12"=w7) -> (w3:T20)  [unwired: 1 in]
  n35 = Bundle("Target.X::9"=w14, "Target.Y::9"=w13) -> (w6:T21)  [unwired: 1 in]
  n36 = Bundle("Target.X::10"=w12, "Target.Y::10"=w11) -> (w5:T22)  [unwired: 1 in]
  n37 = Bundle("Target.X::11"=w10, "Target.Y::11"=w9) -> (w4:T23)  [unwired: 1 in]
  n38 = disable-structure shown="Disabled" {
    frame Disabled {
    }
    frame Enabled {
    }
  }
  n39 = Build Array(w27, w26, w25, w18, w24, w23, w22, w21, w6, w5, w4, w3) -> (w20:T24)
  n40 = property on="Feedback Global" class="Bool (strict)"("Value"=FALSE ("Feedback Global")) -> ()  [unwired: 2 in, 2 out]
  n41 = call <vilib>:"Add State(s) to Queue__jki_lib_state_machine.vi"("State(s) in (\"\")"="Macro: Initialize") -> ("States Out"=w47:string)  [unwired: 14 in]
  n42 = while "JKI - String-Based Queued State Machine (Basic) v1.0" {
    shift-right: [w62] -> w17
    shift-left: _ -> [w56]
    shift-right: [w64] -> w44
    shift-left: _ -> [w61]
    shift-right: [w50] -> _
    shift-left: w47 -> [w65]
    tunnel: w20 -> [w59]
    tunnel: [w51] -> w45
    tunnel: w20 -> [w58]
    stop <- w63 stop-if-true
    n43 = Unbundle By Name(w56) -> ("active cams"=w55:string[], "Mean Centroid X"=w54:dbl[][], "Mean Centroid Y"=w53:dbl[][], "Mean Size"=w52:dbl[][])
    n44 = call <vilib>:"Parse State Queue__jki_lib_state_machine.vi"("State Queue"=w65, "Error In (no error)"=w61) -> ("Remaining States"=w67:string, "Current State"=w48:string, "Arguments"=w66:string)  [unwired: 11 in]
    "Current State" <- w48
    n45 = local read "CCDs"() -> (w51:string[])
    n46 = case shown="\"active\"" w48 {
      selector: w48 -> [_ _ w399 _ _ _ _ _ _ _ _ _ _ _ _ _ _ _ _ _ _ _ _ _ _ _ _ _ _ _ _ _ _ _ _ _ _ _ _ _ _ _ _ _ _ _ _ _ _ _ _ _]
      tunnel: w67 -> [w133 w397 w403 w422 w429 w435 w440 w478 w490 w498 w508 w513 w520 w532 w557 w563 w606 w616 w624 w636 w641 w674 w735 w753 w783 w804 w832 w913 w963 w991 w1008 w1042 w1052 w1057 w1079 w1225 w1391 w1450 w1495 w1543 w1585 w1629 w1634 w1641 w1717 w1766 w1777 w1797 w1894 w1921 w1937 w1959]
      tunnel: w66 -> [_ _ _ _ _ _ _ _ _ _ _ _ w515 w527 _ _ _ _ _ _ _ w651 _ _ _ _ w810 _ w953 _ _ _ _ _ w1080 _ w1382 w1440 w1485 w1532 w1579 _ _ _ _ _ _ _ _ _ _ _]
      tunnel: w56 -> [w131 w394 w401 w412 w426 w433 w437 _ w483 w495 w505 w511 w518 w526 w554 w560 w566 w612 w621 w628 w638 w644 w733 w751 w781 w789 w825 w911 w950 w987 w1005 w1035 w1047 w1054 w1068 w1208 w1376 w1431 w1474 w1527 w1581 w1622 w1631 w1638 w1713 w1763 w1774 w1793 w1892 w1918 w1939 w1950]
      tunnel: [w130 w395 w405 w420 errorcluster {"status"=FALSE, "code"=0, "source"=""} ("error out") w432 w438 w452 w488 w494 w506 w510 w516 w529 w555 w561 w604 w614 w622 w634 w639 w647 w732 w750 w780 w786 w828 w909 w955 w989 w997 w1040 w1050 w1055 w1108 w1238 w1372 w1448 w1493 w1522 w1577 w1627 w1632 w1639 w1714 w1764 w1775 w1786 w1863 w1919 w1935 w1957] -> w64
      tunnel: w61 -> [w129 w395 w404 w420 w423 w432 w438 w452 w480 w494 w506 w510 w517 w530 w555 w561 w604 w614 w622 w634 w639 w645 w732 w750 w780 w787 w829 w910 w940 w989 w998 w1040 w1050 w1055 w1108 w1238 w1371 w1448 w1493 w1521 w1578 w1627 w1632 w1639 w1715 w1764 w1775 w1787 w1890 w1919 w1935 w1957]
      tunnel: [w132 w396 w402 w421 w428 w434 w439 w477 w489 w497 w507 w512 w519 w531 w556 w562 w605 w615 w623 w635 w640 w673 w734 w752 w782 w803 w819 w912 w962 w990 w1007 w1041 w1051 w1056 w1062 w1239 w1390 w1449 w1494 w1542 w1584 w1628 w1633 w1640 w1716 w1765 w1776 w1796 w1893 w1920 w1936 w1958] -> w50
      tunnel: [_ _ _ _ _ TRUE _ _ _ _ _ _ _ _ _ _ _ _ _ _ _ _ _ _ _ _ _ _ _ _ _ _ _ _ _ _ _ _ _ _ _ _ _ _ _ _ _ _ _ _ _ _] -> w63
      tunnel: [w126 w394 w401 w411 w426 w433 w437 w453 w483 w495 w505 w511 w518 w526 w554 w560 w565 w611 w621 w628 w638 w666 w733 w751 w781 w788 w830 w911 w957 w986 w1006 w1034 w1046 w1054 w1061 w1209 w1375 w1430 w1473 w1526 w1583 w1621 w1631 w1638 w1713 w1762 w1774 w1793 w1891 w1918 w1938 w1949] -> w62
      tunnel: "update speed [ms]" -> [w128 _ _ _ _ _ _ _ _ _ _ _ _ _ _ _ _ _ _ _ _ _ _ _ _ _ _ _ _ _ _ _ _ _ _ _ _ _ _ _ _ _ _ _ _ _ _ _ _ _ _ _]
      tunnel: w59 -> [w125 _ _ _ _ _ _ _ _ _ _ _ _ _ _ _ _ _ _ _ _ _ _ _ _ _ _ _ _ _ _ _ _ _ w1059 _ _ _ _ _ _ _ _ _ _ _ _ _ _ w1903 _ _]
      tunnel: w51 -> [w127 _ _ _ _ _ _ _ _ _ _ _ _ _ _ _ _ _ _ _ _ _ _ _ _ _ w831 _ w958 _ _ _ _ _ w1072 w1210 w1389 _ _ w1541 w1580 _ _ w1637 _ _ _ w1792 _ _ _ _]
      tunnel: [w124 w393 w398 w410 w424 w430 w436 w445 w486 w491 w504 w509 w514 w525 w553 w558 w603 w607 w619 w625 w637 w656 w731 w736 w754 w784 w806 w896 w948 w982 w1001 w1033 w1045 w1053 w1060 w1199 w1380 w1439 w1484 w1531 w1576 w1626 w1630 w1635 w1695 w1757 w1773 w1778 w1864 w1901 w1931 w1940] -> w49
      tunnel: w48 -> [w124 w393 w398 w410 w424 w430 w436 w445 w486 w491 w504 w509 w514 w525 w553 w558 w603 w607 w619 w625 w637 w656 w731 w736 w754 w784 w806 w896 w948 w982 w1001 w1033 w1045 w1053 w1060 w1199 w1380 w1439 w1484 w1531 w1576 w1626 w1630 w1635 w1695 w1757 w1773 w1778 w1864 w1901 w1931 w1940]
      frame "", "Idle" {
        # "executes when the state queue is empty"
        n47 = event shown="[9] \"Coupled Mirror Move\": Value Change" {
          selector: _ -> [_ _ _ _ _ _ _ _ _ _ _ _ _ _ _ _ _ _ _ _ _]
          dyn-events: _ -> [_ _ _ _ _ _ _ _ _ _ _ _ _ _ _ _ _ _ _ _ _]
          timeout: w128 -> [_ _ _ _ _ _ _ _ _ _ _ _ _ _ _ _ _ _ _ _ _]
          tunnel: w133 -> [w152 w219 w234 w259 w264 w269 w275 w280 w285 w314 w319 w321 w336 w348 w353 w358 w364 w372 w381 w385 w392]
          tunnel: [w163 w218 w233 w258 w263 w268 w274 w279 w284 w313 w318 w320 w335 w347 w352 w357 w363 w371 w380 w384 w391] -> w132
          tunnel: w131 -> [w141 w216 w231 w255 w261 w266 w272 w277 w282 w286 w316 w324 w334 w346 w351 w356 w362 w370 w374 w386 w389]
          tunnel: [w169 w217 w232 w257 w262 w267 w273 w278 w283 w312 w317 w323 w329 w341 w350 w355 w361 w369 w379 w383 w390] -> w130
          tunnel: w129 -> [w159 w217 w232 w257 w262 w267 w273 w278 w283 w312 w317 w323 w330 w342 w350 w355 w361 w369 w379 w383 w390]
          tunnel: [w145 w216 w231 w254 w261 w266 w272 w277 w282 w286 w316 w324 w334 w346 w351 w356 w362 w370 w374 w386 w389] -> w126
          tunnel: w127 -> [w160 _ w227 _ _ _ _ _ _ _ _ _ _ _ _ _ _ _ _ _ _]
          tunnel: w125 -> [_ _ w229 _ _ _ _ _ _ _ _ _ _ _ _ _ _ _ _ _ _]
          event Timeout {
            n48 = event-data() -> ()  [unwired: 1 in, 1 out]
            n49 = Unbundle By Name(w141) -> ("Detection.img to avg"=w150:i32)
            n50 = Unbundle By Name(w141) -> ("active ccd"=w147:i32)
            n51 = Unbundle By Name(w141) -> ("Detection"=w148:T32, "active cams"=w143:string[])
            n52 = Increment(x=w150) -> (x+1=w164:i32)
            n53 = Array Size(array=w143) -> (size(s)=w142:i32)
            n54 = Greater Or Equal?(x="#imgs avd so far", y=w164) -> (x >= y?=w162:bool)
            n55 = Increment(x="#imgs avd so far") -> (x+1=w166:dbl)
            n56 = call "centroid detection loop.vi"("CCDs"=w160, "error in (no error)"=w159, "active cams"=w143, "Detection in"=w148, "autodetect"="autodetect") -> ("error out"=w157:errorcluster, "# where centr y is 0"=w155:i32[], "Detection out"=w144:T33, "bounding rectangle"=→"Box":T2, "detected array"=→"detected":bool[], "Particle Reports (Pixels)"=w158:T34)  [unwired: 1 in]
            n57 = Equal To 0?(x=w142) -> ()  [unwired: 1 out]
            n58 = Select(t=0.0, s=w162, f=w166) -> (s? t:f=w165:dbl)
            n59 = Unbundle By Name(w141) -> ("Config loaded"=w140:bool)
            n60 = Index Array(array=w158, index (row)=w147) -> (element=w135:T6)  [unwired: 1 in]
            n61 = for {
              tunnel: w135 -> [w175] mode=indexing
              tunnel: [w174] -> w139 mode=indexing
              n62 = Unbundle By Name(w175) -> ("Area"=w174:dbl)
            }
            n63 = call-poly <userlib>:"Sort Array__ogtk.vi"("Order"=enum16{"ascending", "descending"}."descending", "Array in"=w139) -> ("Sorted Pointers"=w137:i32[])  [unwired: 8 in, 1 out]
            n64 = call-poly <userlib>:"Reorder Array2__ogtk.vi"("indices"=w137, "array"=w135) -> ("reordered array"=w136:variant[])  [unwired: 9 in]
            n65 = local write "#imgs avd so far"(w165) -> ()
            n66 = Variant To Data(type=w135, Variant=w136) -> (data=→"active ccd particles":T6)  [unwired: 1 in, 1 out]
            n67 = call <vilib>:"Clear Errors.vi"("error in (no error)"=w157) -> ("error out"=w169:errorcluster)  [unwired: 5 in, 1 out]
            n68 = Unbundle By Name(w144) -> ("img to avg"=w153:i32)
            n69 = for {
              tunnel: w155 -> [w208] mode=indexing
              tunnel: w143 -> [w214] mode=indexing
              shift-right: [w209] -> w170
              shift-left: "" ("GUIdevice 7") -> [w212]
              tunnel: [w203] -> w172 mode=indexing
              tunnel: "Detection Rate" -> [w207]
              tunnel: w165 -> [w205]
              tunnel: w150 -> [w201]
              # "averaging done?"
              n70 = Greater Or Equal?(x=w208, y=w201) -> (x >= y?=w204:bool)
              n71 = Multiply(x=w207, y=w205) -> (x*y=w206:dbl)
              n72 = Greater Or Equal?(x=w208, y=w206) -> (x >= y?=w202:bool)
              n73 = And(x=w204, y=w202) -> (x .and. y?=w203:bool)
              n74 = Select(t=w214, s=w203, f="") -> (s? t:f=w210:string)
              n75 = Concatenate Strings(w212, "\t", w210) -> (w209:string)
            }
            n76 = case shown="True" w140 {
              tunnel: w152 -> [w176 w179]
              tunnel: [w176 w178] -> w151
              frame False {
              }
              frame True {
                n77 = call <vilib>:"Add State(s) to Queue__jki_lib_state_machine.vi"("State(s) in (\"\")"=w179, "State(s) at Back (\"\")"="Device Ini" ("State(s) at Back (\"\")")) -> ("States Out"=w178:string)  [unwired: 13 in]
              }
            }
            n78 = case shown="True" w162 {
              tunnel: w144 -> [w180 w187]
              tunnel: [w180 w186] -> w146
              tunnel: w153 -> [_ w182]
              frame False {
              }
              frame True {
                # "avg done. clear arrays"
                n79 = Decrement(x=w182) -> (x-1=w185:i32)
                n80 = Initialize Array(0.0 ("element"), 12 ("dimension size"), w185) -> (w181:dbl[][])
                n81 = Bundle By Name(cluster=w187, "Centroid X"=w181, "Centroid Y"=w181, "Size"=w181) -> (w186:T33)
              }
            }
            n82 = Bundle By Name(cluster=w141, "Detection"=w146) -> (w145:T35)
            n83 = Or Array Elements(Boolean array=w172) -> (logical OR=w171:bool)
            n84 = case shown="True" w171 {
              tunnel: w170 -> [_ w195]
              tunnel: w151 -> [w188 w194]
              tunnel: [w188 w189] -> w163
              frame False {
                # "avg not done yet"
              }
              frame True {
                # "avg done."
                n85 = local read "Tab Cams"() -> (w192:T3)
                n86 = call <vilib>:"Build State String with Arguments__jki_lib_state_machine.vi"("Arguments (\"\")"=w195, "State"="detected") -> ("State with Arguments"=w193:string)  [unwired: 4 in]
                n87 = call <vilib>:"Add State(s) to Queue__jki_lib_state_machine.vi"("State(s) in Front (\"\")"=w193, "State(s) in (\"\")"=w194) -> ("States Out"=w190:string)  [unwired: 13 in]
                n88 = case shown="Default" w192 {
                  tunnel: w190 -> [w197 w200]
                  tunnel: "stats" ("State") -> [_ w199]
                  tunnel: [w197 w198] -> w189
                  frame Default {
                  }
                  frame "History" {
                    n89 = call <vilib>:"Add State(s) to Queue__jki_lib_state_machine.vi"("State(s) in Front (\"\")"=w199, "State(s) in (\"\")"=w200) -> ("States Out"=w198:string)  [unwired: 13 in]
                  }
                }
              }
            }
          }
          event "stop": Value Change {
            # "Exit Button Value Change (pressed) Event\n(this executes Macro: Exit to terminate the VI)"
            n90 = event-data() -> ()  [unwired: 1 in, 6 out]
            n91 = call <vilib>:"Add State(s) to Queue__jki_lib_state_machine.vi"("State(s) in Front (\"\")"="Macro: Exit", "State(s) in (\"\")"=w219) -> ("States Out"=w218:string)  [unwired: 13 in]
          }
          event Value Change {
            n92 = event-data() -> ()  [unwired: 1 in, 6 out]
            n93 = Unbundle By Name(w231) -> ("active ccd"=w223:i32, "Mean Centroid X"=w222:dbl[][], "Mean Centroid Y"=w221:dbl[][])
            n94 = Index Array(array=w227, index=w223) -> (element=w226:string)
            n95 = Concatenate Strings("Do want to update the target of " ("message"), w226, "?" ("string")) -> (w224:string)
            n96 = property on="Set Centriod Target" class="Bool (strict)"("Value"=FALSE) -> ()  [unwired: 2 in, 2 out]
            n97 = Two Button Dialog(message=w224) -> (T button?=w230:bool)  [unwired: 2 in]
            n98 = case shown="True" w230 {
              tunnel: w229 -> [_ w243]
              tunnel: w223 -> [_ w242]
              tunnel: w222 -> [_ w249]
              tunnel: w221 -> [_ w244]
              frame False {
              }
              frame True {
                n99 = Index Array(array=w249, index (row)=w242) -> (element=w248:dbl[])  [unwired: 1 in]
                n100 = Index Array(array=w244, index (row)=w242) -> (element=w245:dbl[])  [unwired: 1 in]
                n101 = Index Array(array=w243, index=w242) -> (element=w241:T20)
                n102 = Unbundle By Name(w241) -> ("Target.X::12"=w240:refnum<vi>, "Target.Y::12"=w239:refnum<vi>)
                n103 = Reverse 1D Array(array=w248) -> (reversed array=w247:dbl[])
                n104 = Reverse 1D Array(array=w245) -> (reversed array=w246:dbl[])
                n105 = Index Array(array=w247) -> (element=w238:dbl)  [unwired: 1 in]
                n106 = Index Array(array=w246) -> (element=w236:dbl)  [unwired: 1 in]
                n107 = To Unsigned Word Integer(number=w236) -> (unsigned 16bit integer=w235:u16)
                n108 = To Unsigned Word Integer(number=w238) -> (unsigned 16bit integer=w237:u16)
                n109 = disable-structure shown="Enabled" {
                  disable-tunnel: w240 -> [w253 _]
                  disable-tunnel: w237 -> [w252 _]
                  disable-tunnel: w239 -> [w251 _]
                  disable-tunnel: w235 -> [w250 _]
                  frame Enabled {
                    n110 = property class="DigNum (strict)"(reference=w253, "Val(Sgnl)"=w252) -> ()  [unwired: 1 in, 2 out]
                    n111 = property class="DigNum (strict)"(reference=w251, "Val(Sgnl)"=w250) -> ()  [unwired: 1 in, 2 out]
                  }
                  frame Disabled {
                  }
                }
              }
            }
            n112 = call <vilib>:"Add State(s) to Queue__jki_lib_state_machine.vi"("State(s) in (\"\")"=w234) -> ("States Out"=w233:string)  [unwired: 14 in]
          }
          event "Feedback Global": Value Change {
            # "Exit Button Value Change (pressed) Event\n(this executes Macro: Exit to terminate the VI)"
            n113 = event-data() -> ("NewVal"=w256:bool)  [unwired: 1 in, 5 out]
            n114 = call <vilib>:"Add State(s) to Queue__jki_lib_state_machine.vi"("State(s) in (\"\")"=w259) -> ("States Out"=w258:string)  [unwired: 14 in]
            n115 = Bundle By Name(cluster=w255, "Feedback global"=w256) -> (w254:T35)
          }
          event Value Change {
            n116 = event-data() -> ()  [unwired: 1 in, 6 out]
            n117 = call <vilib>:"Add State(s) to Queue__jki_lib_state_machine.vi"("State(s) in Front (\"\")"="set move props from control", "State(s) in (\"\")"=w264) -> ("States Out"=w263:string)  [unwired: 13 in]
          }
          event Value Change {
            n118 = event-data() -> ()  [unwired: 1 in, 6 out]
            n119 = call <vilib>:"Add State(s) to Queue__jki_lib_state_machine.vi"("State(s) in Front (\"\")"="set detection params from control", "State(s) in (\"\")"=w269) -> ("States Out"=w268:string)  [unwired: 13 in]
          }
          event "Reset History": Value Change {
            n120 = event-data() -> ()  [unwired: 1 in, 6 out]
            n121 = call <vilib>:"Add State(s) to Queue__jki_lib_state_machine.vi"("State(s) in (\"\")"=w275, "State(s) at Back (\"\")"="Reset History" ("State(s) at Back (\"\")")) -> ("States Out"=w274:string)  [unwired: 13 in]
            n122 = property on="Reset History" class="Bool (strict)"("Value"=FALSE ("Reset History")) -> ()  [unwired: 2 in, 2 out]
          }
          event "Save Config": Value Change {
            n123 = event-data() -> ()  [unwired: 1 in, 6 out]
            n124 = call <vilib>:"Add State(s) to Queue__jki_lib_state_machine.vi"("State(s) in (\"\")"=w280, "State(s) at Back (\"\")"="Save Config\nStopSuperGUI\nSetCameraNameControls\nCameraRefs\nStartSuperGUI\nDevice Ini >> 3000\nnewtdms" ("State(s) at Back (\"\")")) -> ("States Out"=w279:string)  [unwired: 13 in]
          }
          event "Load Config": Value Change {
            n125 = event-data() -> ()  [unwired: 1 in, 6 out]
            n126 = call <vilib>:"Add State(s) to Queue__jki_lib_state_machine.vi"("State(s) in (\"\")"=w285, "State(s) at Back (\"\")"="StopSuperGUI\nMacro:Start" ("State(s) at Back (\"\")")) -> ("States Out"=w284:string)  [unwired: 13 in]
          }
          event "Coupled Mirror Move": Value Change {
            n127 = event-data() -> ()  [unwired: 1 in, 6 out]
            n128 = Unbundle By Name(w286) -> ("dev var alias arrays.dev variable alias Motors X"=w304:string[][], "dev var alias arrays.dev variable alias Motors Y"=w305:string[][], "move properties"=w306:T11[])  [unwired: 2 out]
            n129 = Index Array(array=w304, index (row)="downstream mirror") -> ()  [unwired: 1 in, 1 out]
            n130 = Index Array(array=w305, index (row)="downstream mirror") -> ()  [unwired: 1 in, 1 out]
            n131 = Index Array(array=w306, index="downstream mirror") -> (element=w302:T11)
            n132 = Index Array(array=w304, index (row)="upstream mirror") -> (element=w309:string[])  [unwired: 1 in]
            n133 = Index Array(array=w305, index (row)="upstream mirror") -> ()  [unwired: 1 in, 1 out]
            n134 = Index Array(array=w306, index="upstream mirror") -> (element=w307:T11)
            n135 = Unbundle By Name(w307) -> ("xCal"=w296:dbl, "yCal"=w293:dbl)  [unwired: 2 out]
            n136 = Unbundle By Name(w302) -> ("xCal"=w297:dbl, "yCal"=w292:dbl)  [unwired: 2 out]
            n137 = call <vilib>:"Add State(s) to Queue__jki_lib_state_machine.vi"("State(s) in (\"\")"=w314, "State(s) at Back (\"\")"="StopSuperGUI\nMacro:Start" ("State(s) at Back (\"\")")) -> ("States Out"=w313:string)  [unwired: 13 in]
            n138 = call "coupled mirror calibration.vi"("seperation"="seperation", "distance to target plane"="distance to target plane", "pixel calib"="pixel calib", "xCal 2"=w297, "xCal"=w296, "x'"="x'", "x"="x") -> ("A2x"=→"A2x":dbl, "A1x"=→"A1x":dbl)  [unwired: 3 in]
            n139 = call "coupled mirror calibration.vi"("seperation"="seperation", "distance to target plane"="distance to target plane", "pixel calib"="pixel calib", "xCal 2"=w292, "xCal"=w293, "x'"="y'", "x"="y") -> ("A2x"=→"A2y":dbl, "A1x"=→"A1y":dbl)  [unwired: 3 in]
            n140 = call "get set udp value from dev var alias array.vi"("get or set"=enum16{"get", "set"}."get", "dev variable alias Motors X"=w309) -> ()  [unwired: 7 in, 3 out]
          }
          event "Save Stats": Value Change {
            n141 = event-data() -> ()  [unwired: 1 in, 6 out]
            n142 = call <vilib>:"Add State(s) to Queue__jki_lib_state_machine.vi"("State(s) in (\"\")"=w319, "State(s) at Back (\"\")"="Save Stats" ("State(s) at Back (\"\")")) -> ("States Out"=w318:string)  [unwired: 13 in]
          }
          event "Tab Cams": Value Change {
            n143 = event-data() -> ()  [unwired: 1 in, 6 out]
            n144 = call <vilib>:"Add State(s) to Queue__jki_lib_state_machine.vi"("State(s) in (\"\")"=w321, "State(s) at Back (\"\")"="stats" ("State")) -> ("States Out"=w320:string)  [unwired: 13 in]
          }
          event "Left", "Right": Value Change {
            n145 = event-data() -> ("CtlRef"=w333:refnum<vi>)  [unwired: 1 in, 5 out]
            n146 = property class="Bool (strict)"(reference=w333, error in=w330) -> (reference out=w332:refnum<vi>, error out=w331:errorcluster, "Label.Text"=w327:string)
            n147 = property class="Bool (strict)"(reference=w332, error in=w331, "Value"=FALSE) -> (error out=w329:errorcluster)  [unwired: 1 out]
            n148 = call <vilib>:"Build State String with Arguments__jki_lib_state_machine.vi"("Arguments (\"\")"=w327, "State"="ManMove X") -> ("State with Arguments"=w326:string)  [unwired: 4 in]
            n149 = call <vilib>:"Add State(s) to Queue__jki_lib_state_machine.vi"("State(s) in (\"\")"=w336, "State(s) at Back (\"\")"=w326) -> ("States Out"=w335:string)  [unwired: 13 in]
          }
          event "Up", "Down": Value Change {
            n150 = event-data() -> ("CtlRef"=w345:refnum<vi>)  [unwired: 1 in, 5 out]
            n151 = property class="Bool (strict)"(reference=w345, error in=w342) -> (reference out=w344:refnum<vi>, error out=w343:errorcluster, "Label.Text"=w339:string)
            n152 = property class="Bool (strict)"(reference=w344, error in=w343, "Value"=FALSE) -> (error out=w341:errorcluster)  [unwired: 1 out]
            n153 = call <vilib>:"Build State String with Arguments__jki_lib_state_machine.vi"("Arguments (\"\")"=w339, "State"="ManMove Y") -> ("State with Arguments"=w338:string)  [unwired: 4 in]
            n154 = call <vilib>:"Add State(s) to Queue__jki_lib_state_machine.vi"("State(s) in (\"\")"=w348, "State(s) at Back (\"\")"=w338) -> ("States Out"=w347:string)  [unwired: 13 in]
          }
          event "Center": Value Change {
            n155 = event-data() -> ()  [unwired: 1 in, 6 out]
            n156 = call <vilib>:"Add State(s) to Queue__jki_lib_state_machine.vi"("State(s) in (\"\")"=w353, "State(s) at Back (\"\")"="Center" ("State(s) at Back (\"\")")) -> ("States Out"=w352:string)  [unwired: 13 in]
          }
          event "new tdms", "tdms root": Value Change {
            n157 = event-data() -> ()  [unwired: 1 in, 6 out]
            n158 = call <vilib>:"Add State(s) to Queue__jki_lib_state_machine.vi"("State(s) in (\"\")"=w358, "State(s) at Back (\"\")"="newtdms" ("State(s) at Back (\"\")")) -> ("States Out"=w357:string)  [unwired: 13 in]
          }
          event "device ini": Value Change {
            n159 = event-data() -> ()  [unwired: 1 in, 6 out]
            n160 = property on="device ini" class="Bool (strict)"("Value"=FALSE ("test")) -> ()  [unwired: 2 in, 2 out]
            n161 = disable-structure shown="Enabled" {
              disable-tunnel: ["Device Ini" ("State(s) at Back (\"\")") "StopSuperGUI\nMacro:Start" ("State(s) at Back (\"\")")] -> w360
              frame Disabled {
              }
              frame Enabled {
              }
            }
            n162 = call <vilib>:"Add State(s) to Queue__jki_lib_state_machine.vi"("State(s) in (\"\")"=w364, "State(s) at Back (\"\")"=w360) -> ("States Out"=w363:string)  [unwired: 13 in]
          }
          event "clear error": Value Change {
            n163 = event-data() -> ()  [unwired: 1 in, 6 out]
            n164 = property on="clear error" class="Bool (strict)"("Value"=FALSE ("test")) -> ()  [unwired: 2 in, 2 out]
            n165 = local write "error out"(errorcluster {"status"=FALSE, "code"=0, "source"=""} ("error out")) -> ()
            n166 = call <vilib>:"Add State(s) to Queue__jki_lib_state_machine.vi"("State(s) in (\"\")"=w372) -> ("States Out"=w371:string)  [unwired: 14 in]
          }
          event "active CCDs": Value Change {
            n167 = event-data() -> ("NewVal"=w375:i32)  [unwired: 1 in, 5 out]
            n168 = Unbundle By Name(w374) -> ("active cams"=w376:string[])
            n169 = Index Array(array=w376, index=w375) -> (element=w377:string)
            n170 = call <vilib>:"Build State String with Arguments__jki_lib_state_machine.vi"("Arguments (\"\")"=w377, "State"="active" ("State(s) at Back (\"\")")) -> ("State with Arguments"=w373:string)  [unwired: 4 in]
            n171 = call <vilib>:"Add State(s) to Queue__jki_lib_state_machine.vi"("State(s) in (\"\")"=w381, "State(s) at Back (\"\")"=w373) -> ("States Out"=w380:string)  [unwired: 13 in]
          }
          event "img to avg": Value Change {
            n172 = event-data() -> ()  [unwired: 1 in, 6 out]
            n173 = call <vilib>:"Add State(s) to Queue__jki_lib_state_machine.vi"("State(s) in Front (\"\")"="ImgToAvg" ("State(s) at Back (\"\")"), "State(s) in (\"\")"=w385) -> ("States Out"=w384:string)  [unwired: 13 in]
          }
          event Panel Close? {
            # "Discard the event because we'll close the front panel ourselves in Macro: Exit"
            # "Close Panel button (pressed) Event\n(this executes Macro: Exit to terminate the VI)"
            n174 = event-data() -> ()  [unwired: 1 in, 1 out]
            n175 = call <vilib>:"Add State(s) to Queue__jki_lib_state_machine.vi"("State(s) in Front (\"\")"="Macro: Exit", "State(s) in (\"\")"=w392) -> ("States Out"=w391:string)  [unwired: 13 in]
            n176 = event-data("Discard?"=TRUE) -> ()  [unwired: 1 in, 1 out]
          }
        }
      }
      frame "---------- Core ----------" {
        # "Do not put any code in this frame.\n(it is a separator no-op)"
        n177 = call <vilib>:"Add State(s) to Queue__jki_lib_state_machine.vi"("State(s) in (\"\")"=w397) -> ("States Out"=w396:string)  [unwired: 14 in]
      }
      frame Default {
        w408 = 42 items=["No error", "Argument error", "Memory is full", "Out of zone", "End of file", "File already open", "Generic file I/O error", "File not found", "File permission error", "Disk is full", "Duplicate path", "Too many files open", "System feature not enabled", "Resource file not found", "Cannot add resource", "Resource not found", "Image not found", "Image memory error", "Pen does not exist", "Config type invalid", "Config token not found", "Config parse error", "Config memory error", "Bad external code format", "Bad external code offset", "External code not present", "Null window", "Destroy window error", "Null menu", "Print aborted", "Bad print record", "Print driver error", "Windows error during printing", "Memory error during printing", "Print dialog error", "Generic print error", "Invalid device refnum", "Device not found", "Device parameter error", "Device unit error", "Cannot open device", "Device call aborted", "Generic error", "Cancelled by user", "Object ID too low", "Object ID too high", "Object not in heap", "Unknown heap", "Unknown object (invalid DefProc)", "Unknown object (DefProc not in table)", "Message out of range", "Invalid (null) method", "Unknown message", "Manager call not supported", "Bad address", "Network operation in progress", "Network operation timed out", "Connection is busy", "Network attribute not supported", "Network error", "Address in use", "System out of memory", "Connection aborted", "Connection refused", "Not connected", "Already connected", "Connection closed", "Initialization error (interapplication manager)", "Bad occurrence", "Wait on unbound occurrence handler", "Occurrence queue overflow", "Datalog type conflict", "Unused", "Unrecognized type (interapplication manager)", "Memory corrupt", "Failed to make temporary DLL", "Old CIN version", "Drag socket not found", "Failed to load drop-object", "Failed to register OLE object", "Failed to release OLE object", "Format specifier type mismatch", "Unknown format specifier", "Too few format specifiers", "Too many format specifiers", "Scan failed", "Newer CIN version", "Error converting to variant", "Runtime menu error", "Password tampered", "Variant attribute not found", "Incompatible variant data type", "Event data is not available", "Event Store is not present", "Occurrence is not found", "Event Queue is not created", "Event info is not available", "Refnum passed is NULL", "Error retrieving Class GUID", "Error retrieving CoClass GUID", "Error retrieving TypeLib GUID.", "Bad built application magic bytes.", "Specific driver is different from the specific driver associated with the Logical Name.", "There is no session opened to the class driver.", "Max Error", "MAX - Error with config objects", "MAX - Error loading configuration", "MAX - Group not supported"]
        # "Current State"
        # "Do not delete, rename, or modify this frame.\n(this is used to capture unhandled states and typos)"
        # "Handle mistyped state name (developer tool)"
        n178 = Format Into String(format string="Software Exception: Unhandled State \"%s\"." ("message"), error in=w404, w399) -> (resulting string=w407:string, error out=w406:errorcluster)  [unwired: 1 in]
        n179 = call <vilib>:"Error Cluster From Error Code.vi"("show call chain? (False)"=TRUE, "error in (no error)"=w406, "error message (\"\")"=w407, "error code (0)"=w408) -> ("error out"=w405:errorcluster)  [unwired: 5 in]
        n180 = call <vilib>:"Add State(s) to Queue__jki_lib_state_machine.vi"("State(s) in (\"\")"=w403) -> ("States Out"=w402:string)  [unwired: 14 in]
      }
      frame "Initialize Core Data" {
        # "Do not delete, rename, or modify this frame.\n(this is used to determine panel behavior on exit)"
        # "originally closed?"
        # "exe?"
        # "If panel starts closed or is an EXE, then close it when we exit"
        n181 = property class="VI"() -> ("Front Panel.Open"=w419:bool)  [unwired: 2 in, 2 out]
        n182 = property class="App"() -> ("App.Kind"=w418:T25)  [unwired: 2 in, 2 out]
        n183 = control-ref of="Current VI Reference"() -> (w413:refnum<vi>)
        n184 = Not(x=w419) -> (.not. x?=w416:bool)
        n185 = Equal?(x=w418, y=T25."Run Time System" ("Application:Kind")) -> (x = y?=w415:bool)
        n186 = Or(x=w416, y=w415) -> (x .or. y?=w414:bool)
        n187 = Bundle By Name(cluster=w412, "Core.Current VI Reference"=w413, "Core.Close Panel on Exit?"=w414) -> (w411:T35)
        n188 = call <vilib>:"Add State(s) to Queue__jki_lib_state_machine.vi"("State(s) in (\"\")"=w422) -> ("States Out"=w421:string)  [unwired: 14 in]
      }
      frame "Error Handler" {
        # "Unhandled Error -- Display it"
        # "Handle any errors here.\nYou can also output any states to clean-up after errors occur"
        # "Clear error"
        n189 = call <vilib>:"Add State(s) to Queue__jki_lib_state_machine.vi"("State(s) in Front (\"\")"="/* Post Error States", "State(s) in (\"\")"=w429) -> ("States Out"=w428:string)  [unwired: 13 in]
        "error out" <- w423
      }
      frame "Exit" {
        # "Do not put any code in this frame.\n(No errors that occur here will be handled.)"
        n190 = call <vilib>:"Add State(s) to Queue__jki_lib_state_machine.vi"("State(s) in (\"\")"=w435) -> ("States Out"=w434:string)  [unwired: 14 in]
      }
      frame "---------- Data ----------" {
        # "Do not put any code in this frame.\n(It is a separator no-op. You can make a copy of this frame to create a new Data frame)"
        n191 = call <vilib>:"Add State(s) to Queue__jki_lib_state_machine.vi"("State(s) in (\"\")"=w440) -> ("States Out"=w439:string)  [unwired: 14 in]
      }
      frame "Data: Initialize" {
        w441 = FALSE  # Config loaded
        w443 = T32 {"detection para"=[{"Filter"=1, "Filter Para"={"X Size"=5, "Y Size"=5, "% Tolerance"=1}, "detection method"=4, "Particle filtering"=[{"Measurement Parameter"=35, "Range Lower Value"=0.0, "Range Upper Value"=0.0, "Range"=TRUE, "Measurement Type"=FALSE}], "Remove small Objects"=TRUE, "Restrict to round Objects"=FALSE, "Use Cam COM"=FALSE}, {"Filter"=1, "Filter Para"={"X Size"=5, "Y Size"=5, "% Tolerance"=1}, "detection method"=4, "Particle filtering"=[{"Measurement Parameter"=35, "Range Lower Value"=0.0, "Range Upper Value"=500.0, "Range"=FALSE, "Measurement Type"=FALSE}], "Remove small Objects"=TRUE, "Restrict to round Objects"=FALSE, "Use Cam COM"=FALSE}, {"Filter"=1, "Filter Para"={"X Size"=5, "Y Size"=5, "% Tolerance"=1}, "detection method"=4, "Particle filtering"=[{"Measurement Parameter"=35, "Range Lower Value"=0.0, "Range Upper Value"=500.0, "Range"=TRUE, "Measurement Type"=FALSE}], "Remove small Objects"=TRUE, "Restrict to round Objects"=FALSE, "Use Cam COM"=FALSE}, {"Filter"=1, "Filter Para"={"X Size"=5, "Y Size"=5, "% Tolerance"=1}, "detection method"=4, "Particle filtering"=[{"Measurement Parameter"=35, "Range Lower Value"=0.0, "Range Upper Value"=500.0, "Range"=TRUE, "Measurement Type"=FALSE}], "Remove small Objects"=TRUE, "Restrict to round Objects"=FALSE, "Use Cam COM"=FALSE}, {"Filter"=1, "Filter Para"={"X Size"=5, "Y Size"=5, "% Tolerance"=1}, "detection method"=4, "Particle filtering"=[{"Measurement Parameter"=35, "Range Lower Value"=0.0, "Range Upper Value"=500.0, "Range"=TRUE, "Measurement Type"=FALSE}], "Remove small Objects"=TRUE, "Restrict to round Objects"=FALSE, "Use Cam COM"=FALSE}, {"Filter"=1, "Filter Para"={"X Size"=5, "Y Size"=5, "% Tolerance"=1}, "detection method"=4, "Particle filtering"=[{"Measurement Parameter"=35, "Range Lower Value"=0.0, "Range Upper Value"=500.0, "Range"=TRUE, "Measurement Type"=FALSE}], "Remove small Objects"=TRUE, "Restrict to round Objects"=FALSE, "Use Cam COM"=FALSE}, {"Filter"=1, "Filter Para"={"X Size"=5, "Y Size"=5, "% Tolerance"=1}, "detection method"=4, "Particle filtering"=[{"Measurement Parameter"=35, "Range Lower Value"=0.0, "Range Upper Value"=500.0, "Range"=TRUE, "Measurement Type"=FALSE}], "Remove small Objects"=TRUE, "Restrict to round Objects"=FALSE, "Use Cam COM"=FALSE}, {"Filter"=1, "Filter Para"={"X Size"=5, "Y Size"=5, "% Tolerance"=1}, "detection method"=3, "Particle filtering"=[{"Measurement Parameter"=35, "Range Lower Value"=0.0, "Range Upper Value"=0.0, "Range"=FALSE, "Measurement Type"=FALSE}], "Remove small Objects"=TRUE, "Restrict to round Objects"=FALSE, "Use Cam COM"=FALSE}, {"Filter"=1, "Filter Para"={"X Size"=5, "Y Size"=5, "% Tolerance"=1}, "detection method"=4, "Particle filtering"=[{"Measurement Parameter"=35, "Range Lower Value"=0.0, "Range Upper Value"=0.0, "Range"=FALSE, "Measurement Type"=FALSE}], "Remove small Objects"=TRUE, "Restrict to round Objects"=FALSE, "Use Cam COM"=FALSE}, {"Filter"=1, "Filter Para"={"X Size"=5, "Y Size"=5, "% Tolerance"=1}, "detection method"=4, "Particle filtering"=[{"Measurement Parameter"=35, "Range Lower Value"=0.0, "Range Upper Value"=500.0, "Range"=TRUE, "Measurement Type"=FALSE}], "Remove small Objects"=TRUE, "Restrict to round Objects"=FALSE, "Use Cam COM"=FALSE}, {"Filter"=1, "Filter Para"={"X Size"=5, "Y Size"=5, "% Tolerance"=1}, "detection method"=4, "Particle filtering"=[{"Measurement Parameter"=35, "Range Lower Value"=0.0, "Range Upper Value"=500.0, "Range"=TRUE, "Measurement Type"=FALSE}], "Remove small Objects"=TRUE, "Restrict to round Objects"=FALSE, "Use Cam COM"=FALSE}, {"Filter"=1, "Filter Para"={"X Size"=5, "Y Size"=5, "% Tolerance"=1}, "detection method"=4, "Particle filtering"=[{"Measurement Parameter"=35, "Range Lower Value"=0.0, "Range Upper Value"=500.0, "Range"=TRUE, "Measurement Type"=FALSE}], "Remove small Objects"=TRUE, "Restrict to round Objects"=FALSE, "Use Cam COM"=FALSE}], "thresholds"=[{"Lower value"=93.0, "Upper value"=255.0}, {"Lower value"=105.0, "Upper value"=255.0}, {"Lower value"=0.0, "Upper value"=255.0}, {"Lower value"=127.0, "Upper value"=255.0}, {"Lower value"=0.0, "Upper value"=255.0}, {"Lower value"=0.0, "Upper value"=255.0}, {"Lower value"=0.0, "Upper value"=255.0}, {"Lower value"=0.0, "Upper value"=255.0}, {"Lower value"=0.0, "Upper value"=255.0}, {"Lower value"=0.0, "Upper value"=255.0}, {"Lower value"=0.0, "Upper value"=255.0}, {"Lower value"=0.0, "Upper value"=255.0}], "Centroid X"=[], "Centroid Y"=[], "Size"=[], "Centroid refs"=[], "img to avg"=6}  # Detection
        w444 = T36 {"Positions x"=[0.0, 0.0, 0.0, 0.0, 0.0, 0.0, 0.0, 0.0, 0.0, 0.0, 0.0, 0.0], "Positions y"=[0.0, 0.0, 0.0, 0.0, 0.0, 0.0, 0.0, 0.0, 0.0, 0.0, 0.0, 0.0]}  # Motor positions
        w446 = T37 {"dev variable alias"=[], "dev variable alias Motors X"=[], "dev variable alias Motors Y"=[]}  # dev var alias arrays
        w464 = dbl[][] []  # Offset Y stats
        w472 = dbl[][] []  # Mean Size
        w470 = T11[] [{"Tolerance [%]"=0.1, "Stepsize"=0.0001, "Invert Direction X"=FALSE, "Invert Direction Y"=TRUE, "enable feedback"=FALSE, "Set Centriod Target"=FALSE, "xCal"=0.0001, "xCal neg"=0.0001, "yCal"=0.0001, "yCal neg"=0.0001}, {"Tolerance [%]"=0.1, "Stepsize"=0.0001, "Invert Direction X"=FALSE, "Invert Direction Y"=TRUE, "enable feedback"=FALSE, "Set Centriod Target"=FALSE, "xCal"=0.0001, "xCal neg"=0.0001, "yCal"=0.0001, "yCal neg"=0.0001}, {"Tolerance [%]"=0.1, "Stepsize"=0.0001, "Invert Direction X"=FALSE, "Invert Direction Y"=TRUE, "enable feedback"=FALSE, "Set Centriod Target"=FALSE, "xCal"=0.0001, "xCal neg"=0.0001, "yCal"=0.0001, "yCal neg"=0.0001}, {"Tolerance [%]"=0.1, "Stepsize"=0.0001, "Invert Direction X"=FALSE, "Invert Direction Y"=TRUE, "enable feedback"=FALSE, "Set Centriod Target"=FALSE, "xCal"=0.0001, "xCal neg"=0.0001, "yCal"=0.0001, "yCal neg"=0.0001}, {"Tolerance [%]"=0.1, "Stepsize"=0.0001, "Invert Direction X"=FALSE, "Invert Direction Y"=TRUE, "enable feedback"=FALSE, "Set Centriod Target"=FALSE, "xCal"=0.0001, "xCal neg"=0.0001, "yCal"=0.0001, "yCal neg"=0.0001}, {"Tolerance [%]"=0.1, "Stepsize"=0.0001, "Invert Direction X"=FALSE, "Invert Direction Y"=TRUE, "enable feedback"=FALSE, "Set Centriod Target"=FALSE, "xCal"=0.0001, "xCal neg"=0.0001, "yCal"=0.0001, "yCal neg"=0.0001}, {"Tolerance [%]"=0.1, "Stepsize"=0.0001, "Invert Direction X"=FALSE, "Invert Direction Y"=TRUE, "enable feedback"=FALSE, "Set Centriod Target"=FALSE, "xCal"=0.0001, "xCal neg"=0.0001, "yCal"=0.0001, "yCal neg"=0.0001}, {"Tolerance [%]"=0.1, "Stepsize"=0.0001, "Invert Direction X"=FALSE, "Invert Direction Y"=TRUE, "enable feedback"=FALSE, "Set Centriod Target"=FALSE, "xCal"=0.0001, "xCal neg"=0.0001, "yCal"=0.0001, "yCal neg"=0.0001}, {"Tolerance [%]"=0.1, "Stepsize"=0.0001, "Invert Direction X"=FALSE, "Invert Direction Y"=TRUE, "enable feedback"=FALSE, "Set Centriod Target"=FALSE, "xCal"=0.0001, "xCal neg"=0.0001, "yCal"=0.0001, "yCal neg"=0.0001}, {"Tolerance [%]"=0.1, "Stepsize"=0.0001, "Invert Direction X"=FALSE, "Invert Direction Y"=TRUE, "enable feedback"=FALSE, "Set Centriod Target"=FALSE, "xCal"=0.0001, "xCal neg"=0.0001, "yCal"=0.0001, "yCal neg"=0.0001}, {"Tolerance [%]"=0.1, "Stepsize"=0.0001, "Invert Direction X"=FALSE, "Invert Direction Y"=TRUE, "enable feedback"=FALSE, "Set Centriod Target"=FALSE, "xCal"=0.0001, "xCal neg"=0.0001, "yCal"=0.0001, "yCal neg"=0.0001}, {"Tolerance [%]"=0.1, "Stepsize"=0.0001, "Invert Direction X"=FALSE, "Invert Direction Y"=TRUE, "enable feedback"=FALSE, "Set Centriod Target"=FALSE, "xCal"=0.0001, "xCal neg"=0.0001, "yCal"=0.0001, "yCal neg"=0.0001}, {"Tolerance [%]"=0.1, "Stepsize"=0.0001, "Invert Direction X"=FALSE, "Invert Direction Y"=TRUE, "enable feedback"=FALSE, "Set Centriod Target"=FALSE, "xCal"=0.0001, "xCal neg"=0.0001, "yCal"=0.0001, "yCal neg"=0.0001}]  # move properties
        w469 = T38 []  # active axis refs 2
        w463 = dbl[][] []  # Motor X
        w462 = dbl[][] []  # Motor Y
        w461 = string[] []  # active cams
        w447 = T39 {"STOP queue"=refnum, "SuperGUI ref"=refnum}  # Supergui
        w448 = dbl[] [0.0, 0.0, 0.0, 0.0, 0.0, 0.0, 0.0, 0.0, 0.0, 0.0, 0.0, 0.0]  # steps speed Y
        w449 = dbl[] [0.0, 0.0, 0.0, 0.0, 0.0, 0.0, 0.0, 0.0, 0.0, 0.0, 0.0, 0.0]  # steps speed X
        w450 = refnum<k34> refnum  # tdms ref
        w451 = bool[] [FALSE, FALSE, FALSE, FALSE, TRUE, TRUE, TRUE, FALSE, FALSE, FALSE, FALSE, FALSE]  # detected
        w458 = bool[] [FALSE, FALSE, FALSE, FALSE, FALSE, FALSE, FALSE, FALSE, FALSE, FALSE, FALSE, TRUE]  # speedmode Y
        w459 = bool[] [FALSE, FALSE, FALSE, FALSE, FALSE, FALSE, FALSE, FALSE, FALSE, FALSE, FALSE, TRUE]  # speedmode X
        w467 = FALSE  # Feedback global
        w468 = 0  # active ccd
        w476 = T40 {"Current VI Reference"=refnum, "Close Panel on Exit?"=FALSE}  # Core
        # "Initialize the shift-register data, here.\n(data names are defined by what you wire into the bundle function)"
        n192 = call <vilib>:"Add State(s) to Queue__jki_lib_state_machine.vi"("State(s) in (\"\")"=w478) -> ("States Out"=w477:string)  [unwired: 14 in]
        n193 = Unbundle By Name(w443) -> ("img to avg"=w442:i32)
        n194 = Bundle("Core"=w476, "Detection"=w443, "Mean Centroid X"="Mean Centroid X", "Mean Centroid Y"=dbl[][] [], "Offset X"="Offset X", "Offset Y"=dbl[][] [], "Offset X stats"=dbl[][] [], "Offset Y stats"=w464, "Mean Size"=w472, "Time"="Time", "move properties"=w470, "active axis refs 2"=w469, "active ccd"=w468, "Feedback global"=w467, "Motor X"=w463, "Motor Y"=w462, "active cams"=w461, "tdms ref"=w450, "active man refs"="active man refs", "detected"=w451, "speedmode X"=w459, "speedmode Y"=w458, "steps speed X"=w449, "steps speed Y"=w448, "Supergui"=w447, "dev var alias arrays"=w446, "Motor positions"=w444, "Config loaded"=w441) -> (w454:T35)  [unwired: 1 in]
        n195 = Initialize Array(0.0 ("element"), 12 ("dimension size"), w442) -> (w457:dbl[][])
        n196 = Bundle By Name(cluster=w454, "Detection.Centroid X"=w457, "Detection.Centroid Y"=w457, "Detection.Size"=w457) -> (w453:T35)
      }
      frame "Data: Cleanup" {
        # "Cleanup any data and references, here.\n(this is called automatically, by the Macro: Exit)"
        n197 = Unbundle By Name(w483) -> ("Core.Current VI Reference"=w487:refnum<vi>)
        n198 = Unbundle By Name(w483) -> ("tdms ref"=w485:refnum<k34>)
        n199 = call "close fgv udp connections.vi"("error in"=w480) -> ("error out"=w479:errorcluster)  [unwired: 10 in]
        n200 = TDMS Close(8:w479, 11:w485) -> (0:w484:errorcluster)  [unwired: 1 out]
        n201 = call <vilib>:"Clear Errors.vi"("error in (no error)"=w484) -> ("error out"=w482:errorcluster)  [unwired: 5 in, 1 out]
        n202 = Merge Errors(w482, w479) -> (w481:errorcluster)
        n203 = Close Reference(reference=w487, error in (no error)=w481) -> (error out=w488:errorcluster)
        n204 = call <vilib>:"Add State(s) to Queue__jki_lib_state_machine.vi"("State(s) in (\"\")"=w490) -> ("States Out"=w489:string)  [unwired: 14 in]
      }
      frame "StopSuperGUI" {
        # "Initialize the User Interface, here.\n(this is called automatically, by the Macro: Init)"
        n205 = Unbundle By Name(w495) -> ("Supergui.SuperGUI ref"=w493:refnum<vi>, "Supergui.STOP queue"=w496:refnum<queue>)
        n206 = Not A Number/Path/Refnum?(number/path/refnum=w493) -> (NaN/Path/Refnum?=w492:bool)
        n207 = case shown="False" w492 {
          tunnel: w496 -> [w503 _]
          tunnel: w493 -> [w499 _]
          frame False {
            n208 = Release Queue(queue=w503) -> (error out=w502:errorcluster)  [unwired: 2 in, 2 out]
            n209 = call-by-ref "Wait On Asynchronous Call"(reference=w499, error in=w502) -> (error out=w501:errorcluster, 0:"error out"=w500:errorcluster)  [unwired: 11 in, 1 out]
            n210 = call <vilib>:"Clear Errors.vi"("error in (no error)"=w500) -> ()  [unwired: 5 in, 2 out]
            n211 = call <vilib>:"Clear Errors.vi"("error in (no error)"=w501) -> ()  [unwired: 5 in, 2 out]
          }
          frame True {
          }
        }
        n212 = call <vilib>:"Add State(s) to Queue__jki_lib_state_machine.vi"("State(s) in (\"\")"=w498) -> ("States Out"=w497:string)  [unwired: 14 in]
      }
      frame "---------- UI ----------" {
        # "Do not put any code in this frame.\n(It is a separator no-op. You can make a copy of this frame to create a new UI frame)"
        n213 = call <vilib>:"Add State(s) to Queue__jki_lib_state_machine.vi"("State(s) in (\"\")"=w508) -> ("States Out"=w507:string)  [unwired: 14 in]
      }
      frame "UI: Initialize" {
        # "Initialize the User Interface, here.\n(this is called automatically, by the Macro: Init)"
        n214 = call <vilib>:"Add State(s) to Queue__jki_lib_state_machine.vi"("State(s) in (\"\")"=w513) -> ("States Out"=w512:string)  [unwired: 14 in]
      }
      frame "UI: Cursor Set" {
        # "Argument"
        # "Set and Unset Cursor Busy.\n(Usage: \"UI: Cursor Set >> Busy|Idle\")"
        n215 = case shown="\"Idle\", Default" w515 {
          tunnel: w517 -> [w522 w524]
          tunnel: [w521 w523] -> w516
          frame "Idle", Default {
            n216 = call <vilib>:"Unset Busy.vi"("error in (no error)"=w522) -> ("error out"=w521:errorcluster)  [unwired: 10 in]
          }
          frame "Busy" {
            n217 = call <vilib>:"Set Busy.vi"("error in (no error)"=w524) -> ("error out"=w523:errorcluster)  [unwired: 9 in, 1 out]
          }
        }
        n218 = call <vilib>:"Add State(s) to Queue__jki_lib_state_machine.vi"("State(s) in (\"\")"=w520) -> ("States Out"=w519:string)  [unwired: 14 in]
      }
      frame "UI: Front Panel State" {
        # "Argument"
        # "Set Front Panel Open or Closed\n(Usage: \"UI: Front Panel State >> Open|Close\")"
        n219 = Unbundle By Name(w526) -> ("Core.Current VI Reference"=w528:refnum<vi>)
        n220 = case shown="\"Open\", Default" w527 {
          tunnel: w530 -> [w536 w547]
          tunnel: [w537 w548] -> w529
          tunnel: w528 -> [_ _]
          frame "Open", Default {
            n221 = property class="VI"(error in=w536) -> (reference out=w534:refnum<vi>, error out=w535:errorcluster, "Front Panel.Open"=w533:bool)  [unwired: 1 in]
            n222 = case shown="False" w533 {
              tunnel: [w540 w543] -> w537
              tunnel: w535 -> [w539 w543]
              tunnel: w534 -> [w538 _]
              frame False {
                n223 = invoke class="VI" method="FP.Open"(reference=w538, error in=w539, "Activate"=TRUE, "State"=T26."Standard") -> (error out=w540:errorcluster)  [unwired: 1 in, 4 out]
              }
              frame True {
              }
            }
          }
          frame "Close" {
            n224 = property class="VI"(error in=w547) -> (reference out=w545:refnum<vi>, error out=w546:errorcluster, "Front Panel.Open"=w544:bool)  [unwired: 1 in]
            n225 = case shown="True" w544 {
              tunnel: [w549 w552] -> w548
              tunnel: w546 -> [w549 w551]
              tunnel: w545 -> [_ w550]
              frame False {
              }
              frame True {
                n226 = invoke class="VI" method="FP.Close"(reference=w550, error in=w551) -> (error out=w552:errorcluster)  [unwired: 1 in, 2 out]
              }
            }
          }
        }
        n227 = call <vilib>:"Add State(s) to Queue__jki_lib_state_machine.vi"("State(s) in (\"\")"=w532) -> ("States Out"=w531:string)  [unwired: 14 in]
      }
      frame "---------- Macro ----------" {
        # "Do not put any code in this frame.\n(It is a separator no-op. You can make a copy of this frame to create a new Macro frame)"
        n228 = call <vilib>:"Add State(s) to Queue__jki_lib_state_machine.vi"("State(s) in (\"\")"=w557) -> ("States Out"=w556:string)  [unwired: 14 in]
      }
      frame "Macro: Initialize" {
        # "Initialization Macro\n(This is called once, when the VI starts)"
        n229 = call <vilib>:"Add State(s) to Queue__jki_lib_state_machine.vi"("State(s) in Front (\"\")"="Data: Initialize\nCentroidRefs\nInitialize Core Data\nUI: Initialize\nUI: Front Panel State >> Open\nGetMotorsFromDB\nMacro:Start", "State(s) in (\"\")"=w563) -> ("States Out"=w562:string)  [unwired: 13 in]
      }
      frame "CentroidRefs" {
        n230 = control-ref of="centroidx::1"() -> (w602:refnum<vi>)
        n231 = control-ref of="centroidy::1"() -> (w601:refnum<vi>)
        n232 = control-ref of="centroidx::2"() -> (w600:refnum<vi>)
        n233 = control-ref of="centroidy::2"() -> (w599:refnum<vi>)
        n234 = control-ref of="centroidx::3"() -> (w598:refnum<vi>)
        n235 = control-ref of="centroidy::3"() -> (w597:refnum<vi>)
        n236 = control-ref of="centroidx::4"() -> (w596:refnum<vi>)
        n237 = control-ref of="centroidy::4"() -> (w595:refnum<vi>)
        n238 = control-ref of="centroidx::5"() -> (w594:refnum<vi>)
        n239 = control-ref of="centroidy::5"() -> (w593:refnum<vi>)
        n240 = control-ref of="centroidx::6"() -> (w592:refnum<vi>)
        n241 = control-ref of="centroidy::6"() -> (w591:refnum<vi>)
        n242 = control-ref of="centroidx::7"() -> (w590:refnum<vi>)
        n243 = control-ref of="centroidy::7"() -> (w589:refnum<vi>)
        n244 = control-ref of="centroidx::8"() -> (w588:refnum<vi>)
        n245 = control-ref of="centroidy::8"() -> (w587:refnum<vi>)
        n246 = control-ref of="centroidx::9"() -> (w578:refnum<vi>)
        n247 = control-ref of="centroidy::9"() -> (w577:refnum<vi>)
        n248 = control-ref of="centroidx::10"() -> (w576:refnum<vi>)
        n249 = control-ref of="centroidy::10"() -> (w575:refnum<vi>)
        n250 = control-ref of="centroidx::11"() -> (w574:refnum<vi>)
        n251 = control-ref of="centroidy::11"() -> (w573:refnum<vi>)
        n252 = control-ref of="centroidx::12"() -> (w572:refnum<vi>)
        n253 = control-ref of="centroidy::12"() -> (w571:refnum<vi>)
        n254 = Bundle("centroidx::1"=w602, "centroidy::1"=w601) -> (w586:T41)  [unwired: 1 in]
        n255 = Bundle("centroidx::2"=w600, "centroidy::2"=w599) -> (w585:T42)  [unwired: 1 in]
        n256 = Bundle("centroidx::3"=w598, "centroidy::3"=w597) -> (w584:T43)  [unwired: 1 in]
        n257 = Bundle("centroidx::4"=w596, "centroidy::4"=w595) -> (w579:T44)  [unwired: 1 in]
        n258 = Bundle("centroidx::5"=w594, "centroidy::5"=w593) -> (w583:T45)  [unwired: 1 in]
        n259 = Bundle("centroidx::6"=w592, "centroidy::6"=w591) -> (w582:T46)  [unwired: 1 in]
        n260 = Bundle("centroidx::7"=w590, "centroidy::7"=w589) -> (w581:T47)  [unwired: 1 in]
        n261 = Bundle("centroidx::8"=w588, "centroidy::8"=w587) -> (w580:T48)  [unwired: 1 in]
        n262 = Bundle("centroidx::12"=w572, "centroidy::12"=w571) -> (w567:T49)  [unwired: 1 in]
        n263 = Bundle("centroidx::9"=w578, "centroidy::9"=w577) -> (w570:T50)  [unwired: 1 in]
        n264 = Bundle("centroidx::10"=w576, "centroidy::10"=w575) -> (w569:T51)  [unwired: 1 in]
        n265 = Bundle("centroidx::11"=w574, "centroidy::11"=w573) -> (w568:T52)  [unwired: 1 in]
        n266 = Build Array(w586, w585, w584, w579, w583, w582, w581, w580, w570, w569, w568, w567) -> (w564:T53)
        n267 = Bundle By Name(cluster=w566, "Detection.Centroid refs"=w564) -> (w565:T35)
        n268 = call <vilib>:"Add State(s) to Queue__jki_lib_state_machine.vi"("State(s) in (\"\")"=w606) -> ("States Out"=w605:string)  [unwired: 14 in]
      }
      frame "GetMotorsFromDB" {
        n269 = call "get all aliases of a class.vi"("class (eg motor)"="motor") -> ("dev variable alias"=w610:string[][])  [unwired: 10 in]
        n270 = Bundle By Name(cluster=w612, "dev var alias arrays.dev variable alias"=w610) -> (w611:T35)
        n271 = Index Array(array=w610, index (col)=2 ("disabled index (col)")) -> (element=w608:string[])  [unwired: 1 in]
        "Names" <- w608
        n272 = property on="Motor Alias Y" class="Ring (strict)"("Strings []"=w608) -> ()  [unwired: 2 in, 2 out]
        n273 = property on="Motor Alias X" class="Ring (strict)"("Strings []"=w608) -> ()  [unwired: 2 in, 2 out]
        n274 = call <vilib>:"Add State(s) to Queue__jki_lib_state_machine.vi"("State(s) in (\"\")"=w616) -> ("States Out"=w615:string)  [unwired: 14 in]
      }
      frame "Macro:Start" {
        # "Dont believe JKI. This state is indeed called with \"load config button\" and more"
        # "Initialization Macro\n(This is called once, when the VI starts)"
        n275 = local write "config path"("" ("config path")) -> ()
        n276 = call <vilib>:"Add State(s) to Queue__jki_lib_state_machine.vi"("State(s) in Front (\"\")"="Load Config\nSetCameraNameControls\nCameraRefs\nStartSuperGUI\nDevice Ini >> 3000\nnewtdms\nImgToAvg", "State(s) in (\"\")"=w624) -> ("States Out"=w623:string)  [unwired: 13 in]
        n277 = local write "active CCDs"(0 ("active CCDs")) -> ()
      }
      frame "Macro: Exit" {
        # "Exit Macro\n(This is called once, when the VI exits)"
        n278 = Unbundle By Name(w628) -> ("Core.Close Panel on Exit?"=w627:bool)
        n279 = Select(t="UI: Front Panel State >> Close", s=w627, f="") -> (s? t:f=w631:string)
        n280 = call <vilib>:"Add State(s) to Queue__jki_lib_state_machine.vi"("State(s) in Front (\"\")"="StopSuperGUI" ("State(s) in Front (\"\")"), "State(s) in (\"\")"=w631, "State(s) at Back (\"\")"="Data: Cleanup\nExit") -> ("States Out"=w629:string)  [unwired: 12 in]
        n281 = call <vilib>:"Add State(s) to Queue__jki_lib_state_machine.vi"("State(s) in Front (\"\")"=w629, "State(s) in (\"\")"=w636) -> ("States Out"=w635:string)  [unwired: 13 in]
      }
      frame "---------- Ini and Configure ----------" {
        # "Template Separator\n(You can make a copy of, or modify, this frame)"
        n282 = call <vilib>:"Add State(s) to Queue__jki_lib_state_machine.vi"("State(s) in (\"\")"=w641) -> ("States Out"=w640:string)  [unwired: 14 in]
      }
      frame "Load Config" {
        w658 = T54 {"Camera"="", "Motor Alias X"=0, "Motor Alias Y"=0}  # Camera and motors
        # "Your code here.\n(You can make a copy of, or modify, this frame)"
        n283 = Unbundle By Name(w644) -> ("Detection.detection para"=w672:T9[], "move properties"=w669:T11[], "Detection.thresholds"=w664:cluster{"Lower value":sgl, "Upper value":sgl}[])
        n284 = Empty String/Path?(string/path=w651) -> (empty?=w652:bool)
        n285 = case shown="True" w652 {
          tunnel: [w690 w699] -> w648
          tunnel: w645 -> [w689 w698]
          tunnel: [w689 w697] -> w649
          tunnel: w651 -> [w691 _]
          frame False {
            n286 = String To Path(string=w691) -> (path=w690:path)
          }
          frame True {
            n287 = call <vilib>:"Application Directory.vi"() -> ("Application Directory"=w693:path)
            n288 = Build Path(base path=w693, name or relative path=path "cfg") -> (appended path=w695:path)
            n289 = call-poly <userlib>:"File Exists__ogtk.vi"("file path"=w695) -> ("exists"=w694:bool)  [unwired: 6 in, 1 out]
            n290 = case shown="True" w694 {
              tunnel: w695 -> [w703 w704]
              tunnel: [w702 w704] -> w692
              frame False {
                n291 = Create Folder(path (use dialog)=w703) -> (created path=w702:path)  [unwired: 2 in, 2 out]
              }
              frame True {
              }
            }
            n292 = call "File Dialog2"("start path"=w692, "error in"=w698, "pattern (all files)"="*.cfg", "pattern label"="config") -> ("selected path"=w699:path, "error out"=w697:errorcluster)  [unwired: 8 in, 2 out]
          }
        }
        n293 = property on="Load Config" class="Bool (strict)"("Value"=FALSE ("Load Config")) -> ()  [unwired: 2 in, 2 out]
        n294 = Path To String(path=w648) -> (string=→"config path":string)
        n295 = case shown="No Error" w649 {
          tunnel: w674 -> [w685 _]
          tunnel: [w684 _] -> w673
          tunnel: w649 -> [w679 _]
          tunnel: w648 -> [w678 _]
          tunnel: [w677 w688] -> w647
          tunnel: [w676 T27 {"Camera names"=[], "Motor aliases x"=[], "Motor aliases y"=[], "detection para"=[], "thresholds"=[], "move properties"=[], "tdms root"=path "c:/BP_DATAsd"} ("BP Configuration")] -> w646
          tunnel: w645 -> [_ w688]
          tunnel: [TRUE ("Config loaded") FALSE ("Config loaded")] -> w642
          frame No Error {
            w680 = T27 {"Camera names"=[], "Motor aliases x"=[], "Motor aliases y"=[], "detection para"=[], "thresholds"=[], "move properties"=[], "tdms root"=path "c:/BP_DATAsd"}  # BP Configuration
            n296 = call <userlib>:"MGI Read Anything.vi"("Type of Anything"=w680, "Error In"=w679, "Path (dialog)"=w678) -> ("Error Out"=w682:errorcluster, "Anything"=w681:variant)  [unwired: 5 in, 2 out]
            n297 = Variant To Data(error in=w682, type=w680, Variant=w681) -> (data=w676:T27, error out=w677:errorcluster)
            n298 = call <vilib>:"Add State(s) to Queue__jki_lib_state_machine.vi"("State(s) in (\"\")"=w685, "State(s) at Back (\"\")"="Motor Config" ("State(s) at Back (\"\")")) -> ("States Out"=w684:string)  [unwired: 13 in]
          }
          frame Error {
          }
        }
        n299 = Unbundle By Name(w646) -> ("Motor aliases x"=w663:string[], "Motor aliases y"=w660:string[], "Camera names"=w655:string[], "detection para"=w671:T9[], "move properties"=w670:T11[], "thresholds"=w665:cluster{"Lower value":sgl, "Upper value":sgl}[], "tdms root"=w650:path)
        n300 = local write "tdms root"(w650) -> ()
        n301 = Bundle By Name(cluster=w644, "Config loaded"=w642) -> (w643:T35)
        n302 = call-poly <userlib>:"Remove Duplicates from 1D Array__ogtk.vi"("Input Array"=w655) -> ("Output Array"=w654:string[])  [unwired: 1 out]
        "CCDs" <- w654
        n303 = property on="Motor Alias X" class="Ring (strict)"() -> ("Strings []"=w659:string[])  [unwired: 2 in, 2 out]
        n304 = for {
          tunnel: w654 -> [w727]
          tunnel: w671 -> [w729]
          tunnel: w670 -> [w728]
          shift-right: [w722] -> w668
          shift-left: w672 -> [w726]
          shift-right: [w720] -> w667
          shift-left: w669 -> [w725]
          tunnel: w665 -> [w721]
          shift-right: [w717] -> w661
          shift-left: w664 -> [w719]
          tunnel: w663 -> [w716]
          tunnel: w660 -> [w714]
          tunnel: w659 -> [w710]
          tunnel: w658 -> [w712]
          tunnel: [w707] -> w657 mode=indexing
          tunnel: w654 -> [w705] mode=indexing
          i -> [w715]
          n305 = call-poly <userlib>:"Filter 1D Array__ogtk.vi"("items to filter"=w705, "array"=w727) -> ("filtered item indices"=w730:i32[])  [unwired: 4 in, 1 out]
          n306 = Index Array(array=w730) -> (element=w713:i32)  [unwired: 1 in]
          n307 = Index Array(array=w714, index=w713) -> (element=w706:string)
          n308 = Index Array(array=w716, index=w713) -> (element=w709:string)
          n309 = Index Array(array=w729, index=w713) -> (element=w724:T9)
          n310 = Index Array(array=w728, index=w713) -> (element=w723:T11)
          n311 = Index Array(array=w721, index=w713) -> (element=w718:cluster{"Lower value":sgl, "Upper value":sgl})
          n312 = Search 1D Array(1D array=w710, element=w706) -> (index of element=w711:i32)  [unwired: 1 in]
          n313 = Search 1D Array(1D array=w710, element=w709) -> (index of element=w708:i32)  [unwired: 1 in]
          n314 = Bundle By Name(cluster=w712, "Camera"=w705, "Motor Alias Y"=w711, "Motor Alias X"=w708) -> (w707:T54)
          n315 = Replace Array Subset(array=w726, new element=w724, index=w715) -> (w722:T9[])
          n316 = Replace Array Subset(array=w725, new element=w723, index=w715) -> (w720:T11[])
          n317 = Replace Array Subset(array=w719, new element=w718, index=w715) -> (w717:cluster{"Lower value":sgl, "Upper value":sgl}[])
        }
        n318 = property on="Cameras and motors" class="Arr (strict)"("Value"=w657) -> ()  [unwired: 2 in, 2 out]
        n319 = Bundle By Name(cluster=w643, "Detection.detection para"=w668, "move properties"=w667, "Detection.thresholds"=w661) -> (w666:T35)
      }
      frame "MotorRefs" {
        n320 = call <vilib>:"Add State(s) to Queue__jki_lib_state_machine.vi"("State(s) in (\"\")"=w735) -> ("States Out"=w734:string)  [unwired: 14 in]
      }
      frame "SetCameraNameControls" {
        # "Initialize the User Interface, here.\n(this is called automatically, by the Macro: Init)"
        n321 = local read "CCDs"() -> (w749:string[])
        n322 = Index Array(array=w749) -> (element #1=w748:string, element #2=w747:string, element #3=w746:string, element #4=w745:string, element #5=w744:string, element #6=w743:string, element #7=w742:string, element #8=w741:string, element #9=w740:string, element #10=w739:string, element #11=w738:string, element #12=w737:string)  [unwired: 12 in]
        n323 = property on="GUIdevice 1" class="Str"("Val(Sgnl)"=w748) -> ()  [unwired: 2 in, 2 out]
        n324 = property on="GUIdevice 2" class="Str"("Val(Sgnl)"=w747) -> ()  [unwired: 2 in, 2 out]
        n325 = property on="GUIdevice 3" class="Str"("Val(Sgnl)"=w746) -> ()  [unwired: 2 in, 2 out]
        n326 = property on="GUIdevice 4" class="Str"("Val(Sgnl)"=w745) -> ()  [unwired: 2 in, 2 out]
        n327 = property on="GUIdevice 5" class="Str"("Val(Sgnl)"=w744) -> ()  [unwired: 2 in, 2 out]
        n328 = property on="GUIdevice 6" class="Str"("Val(Sgnl)"=w743) -> ()  [unwired: 2 in, 2 out]
        n329 = property on="GUIdevice 7" class="Str"("Val(Sgnl)"=w742) -> ()  [unwired: 2 in, 2 out]
        n330 = property on="GUIdevice 8" class="Str"("Val(Sgnl)"=w741) -> ()  [unwired: 2 in, 2 out]
        n331 = property on="GUIdevice 9" class="Str"("Val(Sgnl)"=w740) -> ()  [unwired: 2 in, 2 out]
        n332 = property on="GUIdevice 10" class="Str"("Val(Sgnl)"=w739) -> ()  [unwired: 2 in, 2 out]
        n333 = property on="GUIdevice 11" class="Str"("Val(Sgnl)"=w738) -> ()  [unwired: 2 in, 2 out]
        n334 = property on="GUIdevice 12" class="Str"("Val(Sgnl)"=w737) -> ()  [unwired: 2 in, 2 out]
        n335 = call <vilib>:"Add State(s) to Queue__jki_lib_state_machine.vi"("State(s) in (\"\")"=w753) -> ("States Out"=w752:string)  [unwired: 14 in]
      }
      frame "CameraRefs" {
        w755 = T55 0 items=["Grayscale (U8)", "Grayscale (I16)", "Grayscale (SGL)", "Complex (CSG)", "RGB (U32)", "HSL (U32)", "RGB (U64)", "Grayscale (U16)"] ("Image Type")
        n336 = property on="image::5" class="ImageControl"("Caption.Text"="GUIdevice 5") -> ()  [unwired: 2 in, 2 out]
        n337 = property on="image::7" class="ImageControl"("Caption.Text"="GUIdevice 7") -> ()  [unwired: 2 in, 2 out]
        n338 = property on="image::6" class="ImageControl"("Caption.Text"="GUIdevice 6") -> ()  [unwired: 2 in, 2 out]
        n339 = property on="image::9" class="ImageControl"("Caption.Text"="GUIdevice 9") -> ()  [unwired: 2 in, 2 out]
        n340 = property on="image::1" class="ImageControl"("Caption.Text"="GUIdevice 1") -> ()  [unwired: 2 in, 2 out]
        n341 = property on="image::10" class="ImageControl"("Caption.Text"="GUIdevice 10") -> ()  [unwired: 2 in, 2 out]
        n342 = property on="image::8" class="ImageControl"("Caption.Text"="GUIdevice 8") -> ()  [unwired: 2 in, 2 out]
        n343 = property on="image::2" class="ImageControl"("Caption.Text"="GUIdevice 2") -> ()  [unwired: 2 in, 2 out]
        n344 = property on="image::4" class="ImageControl"("Caption.Text"="GUIdevice 4") -> ()  [unwired: 2 in, 2 out]
        n345 = property on="image::3" class="ImageControl"("Caption.Text"="GUIdevice 3") -> ()  [unwired: 2 in, 2 out]
        n346 = property on="image::11" class="ImageControl"("Caption.Text"="GUIdevice 11") -> ()  [unwired: 2 in, 2 out]
        n347 = property on="image::12" class="ImageControl"("Caption.Text"="GUIdevice 12") -> ()  [unwired: 2 in, 2 out]
        n348 = call "IMAQ Create"("Image Name"="GUIdevice 8", "Image Type"=w755) -> ("New Image"=→"image::8":T5)  [unwired: 3 in, 1 out]
        n349 = call "IMAQ Create"("Image Name"="GUIdevice 9", "Image Type"=w755) -> ("New Image"=→"image::9":T5)  [unwired: 3 in, 1 out]
        n350 = call "IMAQ Create"("Image Name"="GUIdevice 10", "Image Type"=w755) -> ("New Image"=→"image::10":T5)  [unwired: 3 in, 1 out]
        n351 = call "IMAQ Create"("Image Name"="GUIdevice 6", "Image Type"=w755) -> ("New Image"=→"image::6":T5)  [unwired: 3 in, 1 out]
        n352 = call "IMAQ Create"("Image Name"="GUIdevice 7", "Image Type"=w755) -> ("New Image"=→"image::7":T5)  [unwired: 3 in, 1 out]
        n353 = call "IMAQ Create"("Image Name"="GUIdevice 11", "Image Type"=w755) -> ("New Image"=→"image::11":T5)  [unwired: 3 in, 1 out]
        n354 = call "IMAQ Create"("Image Name"="GUIdevice 12", "Image Type"=w755) -> ("New Image"=→"image::12":T5)  [unwired: 3 in, 1 out]
        n355 = call "IMAQ Create"("Image Name"="GUIdevice 2") -> ("New Image"=→"image::2":T5)  [unwired: 4 in, 1 out]
        n356 = call "IMAQ Create"("Image Name"="GUIdevice 4", "Image Type"=w755) -> ("New Image"=→"image::4":T5)  [unwired: 3 in, 1 out]
        n357 = call "IMAQ Create"("Image Name"="GUIdevice 1", "Image Type"=w755) -> ("New Image"=→"image::1":T5)  [unwired: 3 in, 1 out]
        n358 = call "IMAQ Create"("Image Name"="GUIdevice 3", "Image Type"=w755) -> ("New Image"=→"image::3":T5)  [unwired: 3 in, 1 out]
        n359 = call "IMAQ Create"("Image Name"="GUIdevice 5", "Image Type"=w755) -> ("New Image"=→"image::5":T5)  [unwired: 3 in, 1 out]
        n360 = call <vilib>:"Add State(s) to Queue__jki_lib_state_machine.vi"("State(s) in (\"\")"=w783) -> ("States Out"=w782:string)  [unwired: 14 in]
      }
      frame "StartSuperGUI" {
        # "create stop queue for supergui and its clones"
        # "can make an icon"
        # "x100 abort will be dependent on caller VI\nx80 abort will be independent of caller vi, this will abort vi when labview is closed."
        # "Initialize the User Interface, here.\n(this is called automatically, by the Macro: Init)"
        n361 = vi-ref "GUI_Master_subvi_reentrant_queues.vi"() -> (w792:refnum<vi>)
        n362 = call "supergui create stop queue.vi"() -> ("STOP Queue out"=w793:refnum<queue>)  [unwired: 11 in]
        n363 = control-ref of="This Application"() -> (w796:refnum<vi>)
        n364 = property class="VI"(reference=w792) -> ("Path"=w791:path)  [unwired: 1 in, 2 out]
        n365 = control-ref of="This VI"() -> (w795:refnum<vi>)
        n366 = Create User Event(user event datatype=T28 {"EventEnum"=enum."new data", "Device name"="Device name"} ("New Event"), error in=w787) -> (user event=w797:refnum<user-event>, error out=w798:errorcluster)
        "tcp data event 2" <- w797
        n367 = Current VI's Menubar() -> (w794:refnum<k9>)
        n368 = register-events(w797) -> ()  [unwired: 2 in, 2 out]
        n369 = Open VI Reference(type specifier VI Refnum (for type only)=refnum<vi> refnum, vi path=w791, options=256, error in (no error)=w787) -> (vi reference=w802:refnum<vi>, error out=w801:errorcluster)  [unwired: 2 in]
        n370 = call <vilib>:"Add State(s) to Queue__jki_lib_state_machine.vi"("State(s) in (\"\")"=w804) -> ("States Out"=w803:string)  [unwired: 14 in]
        n371 = call-by-ref "Start Asynchronous Call"(reference=w802, error in=w801, "STOP Queue in"=w793, "This Application"=w796, 8:"error in (no error)"=w798, "tcp data event"=w797, "Caller menu reference"=w794, "Caller VI ref"=w795) -> (reference out=w790:refnum<vi>, error out=w786:errorcluster)  [unwired: 5 in, 1 out]
        n372 = Bundle By Name(cluster=w789, "Supergui.SuperGUI ref"=w790, "Supergui.STOP queue"=w793) -> (w788:T35)
      }
      frame "Device Ini" {
        n373 = Empty String/Path?(string/path=w810) -> (empty?=w827:bool)
        n374 = flat-sequence {
          tunnel: w831 -> [w834]
          tunnel: [w834] -> w805
          tunnel: w826 -> [w833]
          tunnel: w805 -> [w839]
          tunnel: [w837] -> w813
          frame #0 {
            # "check"
            n375 = Wait (ms)(milliseconds to wait=w833) -> ()  [unwired: 1 out]
          }
          frame #1 {
            # "check if cam images are new"
            n376 = local read "cam means"() -> (w835:sgl[])
            n377 = for {
              tunnel: w839 -> [w842] mode=indexing
              shift-right: [w847] -> w837
              shift-left: string[] [] -> [w848]
              tunnel: [w841] -> w836 mode=indexing
              shift-right: [w845] -> _
              shift-left: w835 -> [w845]
              i -> [w846]
              n378 = call "IMAQ Histograph"("Image"=w842) -> ("error out"=w840:errorcluster, "Mean Value"=w841:sgl)  [unwired: 7 in, 2 out]
              n379 = Index Array(array=w845, index=w846) -> (element=w844:sgl)
              n380 = call <vilib>:"Clear Errors.vi"("error in (no error)"=w840) -> ()  [unwired: 5 in, 2 out]
              n381 = Equal?(x=w841, y=w844) -> (x = y?=w843:bool)
              n382 = case shown="False" w843 {
                tunnel: w848 -> [w851 w852]
                tunnel: [w850 w852] -> w847
                tunnel: w842 -> [w849 _]
                frame False {
                  n383 = Build Array (concatenate)(w851, w849) -> (w850:string[])
                }
                frame True {
                }
              }
            }
            "cam means" <- w836
          }
        }
        n384 = case shown="False" w827 {
          tunnel: w810 -> [w888 _]
          tunnel: [w887 0] -> w826
          frame False {
            n385 = Decimal String To Number(string=w888) -> (number=w887:i32)  [unwired: 2 in, 1 out]
          }
          frame True {
          }
        }
        n386 = Unbundle By Name(w825) -> ("active cams"=w818:string[])
        n387 = Equal?(x=w810, y="T") -> (x = y?=w808:bool)
        n388 = Equal?(x=w818, y=w813) -> (x = y?=w824:bool[])
        n389 = Empty Array?(array=w818) -> (empty?=w823:bool)
        n390 = Not(x=w823) -> (.not. x?=w822:bool)
        n391 = Build Array (concatenate)(w824, w822) -> (w821:bool[])
        n392 = Array Size(array=w813) -> (size(s)=w817:i32)
        n393 = Array Size(array=w818) -> (size(s)=w816:i32)
        n394 = And Array Elements(Boolean array=w821) -> (logical AND=w814:bool)
        n395 = Equal?(x=w817, y=w816) -> (x = y?=w815:bool)
        n396 = And(x=w815, y=w814) -> (x .and. y?=w812:bool)
        n397 = Not(x=w812) -> (.not. x?=w809:bool)
        n398 = Or(x=w809, y=w808) -> (x .or. y?=w807:bool)
        n399 = call <vilib>:"Add State(s) to Queue__jki_lib_state_machine.vi"("State(s) in (\"\")"=w832) -> ("States Out"=w820:string)  [unwired: 14 in]
        n400 = case shown="True" w807 {
          tunnel: [w855 w870] -> w830
          tunnel: w829 -> [w854 w869]
          tunnel: [w854 w869] -> w828
          tunnel: w825 -> [w855 w866]
          tunnel: w813 -> [_ w859]
          tunnel: w820 -> [w853 w857]
          tunnel: [w853 w862] -> w819
          frame False {
          }
          frame True {
            # "#todo check repercussion of not loading config here"
            # "# active cams changed, perform configuration"
            n401 = local write "#imgs avd so far"(0.0 ("Numeric")) -> ()
            n402 = property on="active CCDs" class="LstBox (strict)"("Item Names"=w859) -> ()  [unwired: 2 in, 2 out]
            n403 = Bundle By Name(cluster=w866, "active cams"=w859) -> (w858:T35)
            n404 = Array Size(array=w859) -> (size(s)=w876:i32)
            n405 = Initialize Array(0.0 ("element"), w876, 0 ("dimension size")) -> (w871:dbl[][])
            n406 = Unbundle By Name(w858) -> ("Detection.img to avg"=w865:i32)
            n407 = Initialize Array(0.0 ("element"), 12 ("dimension size"), w865) -> (w864:dbl[][])
            n408 = for {
              N: 1 -> [_]
              shift-right: [w881] -> w874
              shift-left: timestamp[][] [] ("Time") -> [w883]
              n409 = for {
                N: 12 -> [_]
                tunnel: w883 -> [w886] mode=indexing
                tunnel: [w884] -> w881 mode=indexing
                n410 = Get Date/Time In Seconds() -> (seconds since 1Jan1904=w885:timestamp)
                n411 = Build Array (concatenate)(w886, w885) -> (w884:timestamp[])
              }
            }
            n412 = Bundle By Name(cluster=w858, "Offset X stats"=w871, "Offset Y stats"=w871, "Detection.Centroid X"=w864, "Detection.Centroid Y"=w864, "Mean Centroid X"=w871, "Mean Centroid Y"=w871, "Offset X"=w871, "Offset Y"=w871, "Detection.Size"=w864, "Mean Size"=w871, "Motor X"=w871, "Motor Y"=w871) -> (w870:T35)
            n413 = disable-structure shown="Disabled" {
              disable-tunnel: [w878 _] -> w861
              frame Disabled {
                n414 = property on="config path" class="Str"() -> ("Value"=w879:string)  [unwired: 2 in, 2 out]
                n415 = call <vilib>:"Build State String with Arguments__jki_lib_state_machine.vi"("Arguments (\"\")"=w879, "State"="Load Config" ("State(s) in Front (\"\")")) -> ("State with Arguments"=w878:string)  [unwired: 4 in]
              }
              frame Enabled {
              }
            }
            n416 = property on="Time" class="Arr (strict)"("Value"=w874) -> ()  [unwired: 2 in, 2 out]
            n417 = call <vilib>:"Add State(s) to Queue__jki_lib_state_machine.vi"("State(s) in (\"\")"=w857, "State(s) at Back (\"\")"="active\nCenter" ("State(s) in Front (\"\")")) -> ("States Out"=w863:string)  [unwired: 13 in]
            n418 = call <vilib>:"Add State(s) to Queue__jki_lib_state_machine.vi"("State(s) in (\"\")"=w863, "State(s) at Back (\"\")"=w861) -> ("States Out"=w862:string)  [unwired: 13 in]
            "name array" <- w859
          }
        }
      }
      frame "Save Config" {
        w902 = T27 {"Camera names"=[], "Motor aliases x"=[], "Motor aliases y"=[], "detection para"=[], "thresholds"=[], "move properties"=[], "tdms root"=path "c:/BP_DATAsd"}  # BP Configuration
        n419 = property on="Save Config" class="Bool (strict)"("Value"=FALSE ("Save Config")) -> ()  [unwired: 2 in, 2 out]
        n420 = local read "Cameras and motors"() -> (w897:T4)
        n421 = property on="Motor Alias X" class="Ring (strict)"() -> ("Strings []"=w898:string[])  [unwired: 2 in, 2 out]
        n422 = call "File Dialog"("pattern (all files)"="*.cfg", "pattern label"="config") -> ("selected path"=w892:path)  [unwired: 10 in, 3 out]
        n423 = for {
          tunnel: [w919] -> w901 mode=indexing
          tunnel: [w915] -> w900 mode=indexing
          tunnel: w898 -> [w917]
          tunnel: w897 -> [w920] mode=indexing
          tunnel: [w914] -> w895 mode=indexing
          n424 = Unbundle By Name(w920) -> ("Camera"=w914:string, "Motor Alias X"=w918:u16, "Motor Alias Y"=w916:u16)
          n425 = Index Array(array=w917, index=w916) -> (element=w915:string)
          n426 = Index Array(array=w917, index=w918) -> (element=w919:string)
        }
        n427 = Unbundle By Name(w911) -> ("move properties"=w905:T11[], "Detection.detection para"=w904:T9[], "Detection.thresholds"=w903:cluster{"Lower value":sgl, "Upper value":sgl}[])
        n428 = local read "tdms root"() -> (w894:path)
        n429 = Bundle By Name(cluster=w902, "Camera names"=w895, "move properties"=w905, "detection para"=w904, "thresholds"=w903, "Motor aliases x"=w901, "Motor aliases y"=w900, "tdms root"=w894) -> (w899:T27)
        n430 = disable-structure shown="Enabled" {
          disable-tunnel: w910 -> [w924 w932]
          disable-tunnel: [w923 w931] -> w909
          disable-tunnel: w892 -> [w922 w930]
          disable-tunnel: w899 -> [w921 w933]
          frame Disabled {
            n431 = Open/Create/Replace File(file path (use dialog)=w922, error in=w924, operation (0:open)=T29."replace or create with confirmation") -> (refnum out=w926:refnum<file>, error out=w927:errorcluster)  [unwired: 3 in, 1 out]
            n432 = Write to Binary File(file (use dialog)=w926, data=w921, error in=w927) -> (refnum out=w929:refnum<file>, error out=w928:errorcluster)  [unwired: 3 in, 1 out]
            n433 = Close File(refnum=w929, error in=w928) -> (error out=w923:errorcluster)  [unwired: 1 out]
          }
          frame Enabled {
            n434 = call <userlib>:"MGI Write Anything.vi"("Error In"=w932, "Anything"=w933, "Path (dialog)"=w930) -> ("Error Out"=w931:errorcluster)  [unwired: 6 in, 2 out]
          }
        }
        n435 = Path To String(path=w892) -> (string=w891:string)
        n436 = call <vilib>:"Build State String with Arguments__JKI_lib_State_Machine.vi"("Arguments (\"\")"=w891, "State"="Load Config" ("State(s) at Back (\"\")")) -> ("State with Arguments"=w890:string)  [unwired: 4 in]
        n437 = call <vilib>:"Add State(s) to Queue__jki_lib_state_machine.vi"("State(s) in Front (\"\")"=w890, "State(s) in (\"\")"=w913) -> ("States Out"=w912:string)  [unwired: 13 in]
      }
      frame "active" {
        # "problem. when trying to change move config or beam\ndet para, it kees getting overwritten here"
        n438 = Empty String/Path?(string/path=w953) -> (empty?=w952:bool)
        n439 = Unbundle By Name(w950) -> ("move properties"=w960:T11[], "Detection.detection para"=w956:T9[], "active ccd"=w943:i32, "active cams"=w942:string[], "Detection.thresholds"=w934:cluster{"Lower value":sgl, "Upper value":sgl}[])
        n440 = Unbundle By Name(w950) -> ("dev var alias arrays.dev variable alias Motors X"=w947:string[][], "dev var alias arrays.dev variable alias Motors Y"=w945:string[][])
        n441 = call-poly <userlib>:"Filter 1D Array__ogtk.vi"("items to filter"=w953, "array"=w958) -> ("filtered item indices"=w961:i32[])  [unwired: 4 in, 1 out]
        n442 = Index Array(array=w961) -> (element=w951:i32)  [unwired: 1 in]
        n443 = Select(t=w943, s=w952, f=w951) -> (s? t:f=w936:i32)
        n444 = Index Array(array=w960, index=w936) -> (element=w959:T11)
        n445 = Index Array(array=w956, index=w936) -> (element=w937:T9)
        n446 = Index Array(array=w934, index=w936) -> (element=w935:cluster{"Lower value":sgl, "Upper value":sgl})
        n447 = property on="move config" class="Clust (strict)"(error in=w940, "Value"=w959) -> (error out=w954:errorcluster)  [unwired: 1 in, 1 out]
        n448 = local write "thresholds"(w935) -> ()
        n449 = Index Array(array=w942, index=w936) -> (element=→"Active CCD":string)
        n450 = property on="beam detection para" class="Clust (strict)"(error in=w954, "Value"=w937) -> (error out=w939:errorcluster)  [unwired: 1 in, 1 out]
        n451 = disable-structure shown="Enabled" {
          disable-tunnel: w947 -> [w973 w981]
          disable-tunnel: [w971 w980] -> w946
          disable-tunnel: w945 -> [w969 w979]
          disable-tunnel: [w968 w978] -> w944
          disable-tunnel: w936 -> [w967 w977]
          disable-tunnel: w939 -> [w966 w976]
          disable-tunnel: [w964 w974] -> w938
          frame Disabled {
            n452 = call "Beampointing get set motor position.vi"("Active CCD"=w967, "error in (no error)"=w966, "get or set"=enum16{"get", "set"}."get", "dev variable alias Motors X"=w969) -> ("error out"=w965:errorcluster, "Actual Position"=w968:dbl)  [unwired: 6 in]
            n453 = call "Beampointing get set motor position.vi"("Active CCD"=w967, "error in (no error)"=w965, "get or set"=enum16{"get", "set"}."get", "dev variable alias Motors X"=w973) -> ("error out"=w964:errorcluster, "Actual Position"=w971:dbl)  [unwired: 6 in]
          }
          frame Enabled {
            n454 = call "Beampointing get motor position tcp.vi"("Active CCD"=w977, "error in (no error)"=w976, "dev variable alias Motors X"=w979) -> ("error out"=w975:errorcluster, "value"=w978:dbl)  [unwired: 7 in]
            n455 = call "Beampointing get motor position tcp.vi"("Active CCD"=w977, "error in (no error)"=w975, "dev variable alias Motors X"=w981) -> ("error out"=w974:errorcluster, "value"=w980:dbl)  [unwired: 7 in]
          }
        }
        n456 = call <vilib>:"Add State(s) to Queue__jki_lib_state_machine.vi"("State(s) in (\"\")"=w963) -> ("States Out"=w962:string)  [unwired: 14 in]
        n457 = Bundle By Name(cluster=w950, "active ccd"=w936) -> (w957:T35)
        n458 = property on="Position 1" class="DigNum (strict)"(error in=w938, "Value"=w946) -> (error out=w949:errorcluster)  [unwired: 1 in, 1 out]
        n459 = property on="Position 2" class="DigNum (strict)"(error in=w949, "Value"=w944) -> (error out=w955:errorcluster)  [unwired: 1 in, 1 out]
      }
      frame "set detection params from control" {
        # "Your code here.\n(You can make a copy of, or modify, this frame)"
        n460 = Unbundle By Name(w987) -> ("Detection.detection para"=w983:T9[], "active ccd"=w988:i32)
        n461 = Replace Array Subset(array=w983, new element="beam detection para", index=w988) -> (w984:T9[])
        n462 = Bundle By Name(cluster=w987, "Detection.detection para"=w984) -> (w986:T35)
        n463 = call <vilib>:"Add State(s) to Queue__jki_lib_state_machine.vi"("State(s) in (\"\")"=w991) -> ("States Out"=w990:string)  [unwired: 14 in]
      }
      frame "Motor Config" {
        n464 = for {
          tunnel: w1005 -> [w1028]
          tunnel: "Cameras and motors" -> [w1027] mode=indexing
          tunnel: [w1015] -> w1003 mode=indexing
          tunnel: [w1020] -> w1002 mode=indexing
          tunnel: [w1018] -> w1000 mode=indexing
          tunnel: [w1016] -> w999 mode=indexing
          tunnel: w998 -> [w1013]
          tunnel: [w1012] -> w997
          tunnel: [w1010] -> w996 mode=indexing
          tunnel: [w1009] -> w995 mode=indexing
          w1011 = 3000 ("slow timeout ms (3000)")
          n465 = Unbundle By Name(w1028) -> ("dev var alias arrays.dev variable alias"=w1024:string[][])
          n466 = Index Array(array=w1024, index (col)=2 ("disabled index (col)")) -> (element=w1023:string[])  [unwired: 1 in]
          n467 = Unbundle By Name(w1027) -> ("Motor Alias X"=w1032:u16, "Motor Alias Y"=w1022:u16)
          n468 = property on="Motor Alias X" class="Ring (strict)"() -> ("Strings []"=w1021:string[])  [unwired: 2 in, 2 out]
          n469 = Index Array(array=w1021, index=w1032) -> (element=w1031:string)
          n470 = Search 1D Array(1D array=w1023, element=w1031) -> (index of element=w1030:i32)  [unwired: 1 in]
          n471 = Index Array(array=w1024, index (row)=w1030) -> (element=w1015:string[])  [unwired: 1 in]
          n472 = Index Array(array=w1021, index=w1022) -> (element=w1025:string)
          n473 = Search 1D Array(1D array=w1023, element=w1025) -> (index of element=w1026:i32)  [unwired: 1 in]
          n474 = Index Array(array=w1024, index (row)=w1026) -> (element=w1020:string[])  [unwired: 1 in]
          n475 = call "get set udp value from dev var alias array.vi"("slow timeout ms (3000)"=w1011, "error in (no error)"=w1013, "get or set"=enum16{"get", "set"}."get", "dev variable alias Motors X"=w1020) -> ("error out"=w1014:errorcluster, "No errors =T"=w1009:bool, "Numeric"=w1018:dbl)  [unwired: 5 in]
          n476 = call "get set udp value from dev var alias array.vi"("slow timeout ms (3000)"=w1011, "error in (no error)"=w1014, "get or set"=enum16{"get", "set"}."get", "dev variable alias Motors X"=w1015) -> ("error out"=w1012:errorcluster, "No errors =T"=w1010:bool, "Numeric"=w1016:dbl)  [unwired: 5 in]
        }
        n477 = call <vilib>:"Add State(s) to Queue__jki_lib_state_machine.vi"("State(s) in (\"\")"=w1008) -> ("States Out"=w1007:string)  [unwired: 14 in]
        n478 = And Array Elements(Boolean array=w996) -> (logical AND=w994:bool)
        n479 = And Array Elements(Boolean array=w995) -> (logical AND=w993:bool)
        n480 = And(x=w994, y=w993) -> (x .and. y?=→"all UDP in motor config good":bool)
        n481 = Bundle By Name(cluster=w1005, "dev var alias arrays.dev variable alias Motors X"=w1003, "dev var alias arrays.dev variable alias Motors Y"=w1002, "Motor positions.Positions x"=w999, "Motor positions.Positions y"=w1000) -> (w1006:T35)
      }
      frame "set move props from control" {
        # "Your code here.\n(You can make a copy of, or modify, this frame)"
        n482 = Unbundle By Name(w1035) -> ("move properties"=w1039:T11[], "active ccd"=w1038:i32)
        n483 = Replace Array Subset(array=w1039, new element="move config", index=w1038) -> (w1036:T11[])
        n484 = Bundle By Name(cluster=w1035, "move properties"=w1036) -> (w1034:T35)
        n485 = call <vilib>:"Add State(s) to Queue__jki_lib_state_machine.vi"("State(s) in (\"\")"=w1042) -> ("States Out"=w1041:string)  [unwired: 14 in]
      }
      frame "set thresholds" {
        # "Your code here.\n(You can make a copy of, or modify, this frame)"
        n486 = Unbundle By Name(w1047) -> ("Detection.thresholds"=w1049:cluster{"Lower value":sgl, "Upper value":sgl}[], "active ccd"=w1048:i32)
        n487 = Replace Array Subset(array=w1049, new element="thresholds", index=w1048) -> (w1043:cluster{"Lower value":sgl, "Upper value":sgl}[])
        n488 = Bundle By Name(cluster=w1047, "Detection.thresholds"=w1043) -> (w1046:T35)
        n489 = call <vilib>:"Add State(s) to Queue__jki_lib_state_machine.vi"("State(s) in (\"\")"=w1052) -> ("States Out"=w1051:string)  [unwired: 14 in]
      }
      frame "----------Centroid & Move----------" {
        # "Template Separator\n(You can make a copy of, or modify, this frame)"
        n490 = call <vilib>:"Add State(s) to Queue__jki_lib_state_machine.vi"("State(s) in (\"\")"=w1057) -> ("States Out"=w1056:string)  [unwired: 14 in]
      }
      frame "detected" {
        n491 = Unbundle By Name(w1068) -> ("Offset X"=w1100:dbl[][], "Offset Y"=w1099:dbl[][], "Detection.Size"=w1098:dbl[][], "Mean Size"=w1097:dbl[][], "Time"=w1094:timestamp[][], "Motor X"=w1077:dbl[][], "Motor positions"=w1076:T36, "Motor Y"=w1075:dbl[][])  [unwired: 1 out]
        n492 = Spreadsheet String To Array(format string="%s", spreadsheet string=w1080, array type (2D Dbl)=string[] []) -> (array=w1071:string[])  [unwired: 1 in]
        n493 = for {
          tunnel: w1072 -> [w1112] mode=indexing
          tunnel: w1071 -> [w1111]
          tunnel: [w1110] -> w1070 mode=indexing
          n494 = for {
            tunnel: w1112 -> [w1115]
            tunnel: [w1114] -> w1109 mode=indexing
            tunnel: w1111 -> [w1113] mode=indexing
            n495 = Equal?(x=w1115, y=w1113) -> (x = y?=w1114:bool)
          }
          n496 = Or Array Elements(Boolean array=w1109) -> (logical OR=w1110:bool)
        }
        n497 = local read "Cameras and motors"() -> (w1058:T4)
        n498 = Unbundle By Name(w1068) -> ("Mean Centroid X"=w1103:dbl[][], "Mean Centroid Y"=w1102:dbl[][], "Detection.Centroid X"=w1105:dbl[][], "Detection.Centroid Y"=w1104:dbl[][])
        n499 = call <vilib>:"Add State(s) to Queue__jki_lib_state_machine.vi"("State(s) in (\"\")"=w1079) -> ("States Out"=w1078:string)  [unwired: 14 in]
        n500 = for {
          tunnel: w1105 -> [w1165]
          tunnel: w1104 -> [w1164]
          tunnel: w1103 -> [w1163]
          tunnel: w1102 -> [w1162]
          tunnel: [w1161] -> w1091 mode=indexing
          tunnel: [w1160] -> w1101 mode=indexing
          tunnel: w1100 -> [w1159]
          tunnel: w1099 -> [w1158]
          tunnel: [w1157] -> w1069 mode=indexing
          tunnel: [w1156] -> w1092 mode=indexing
          tunnel: w1098 -> [w1155]
          tunnel: w1097 -> [w1154]
          tunnel: [w1153] -> w1096 mode=indexing
          tunnel: w1094 -> [w1152]
          tunnel: [w1151] -> w1093 mode=indexing
          tunnel: w1077 -> [w1148]
          tunnel: w1076 -> [w1121]
          tunnel: w1075 -> [w1147]
          tunnel: [w1127] -> w1074 mode=indexing
          tunnel: [w1126] -> w1073 mode=indexing
          tunnel: w1070 -> [w1125]
          tunnel: w1059 -> [w1123]
          tunnel: w1058 -> [_] mode=indexing
          i -> [w1117]
          n501 = Index Array(array=w1123, index=w1117) -> (element=w1122:T20)
          n502 = Unbundle By Name(w1121) -> ("Positions x"=w1120:dbl[], "Positions y"=w1118:dbl[])
          n503 = Unbundle By Name(w1122) -> ("Target.X::12"=w1131:refnum<vi>, "Target.Y::12"=w1130:refnum<vi>)
          n504 = Index Array(array=w1148, index (row)=w1117) -> (element=w1149:dbl[])  [unwired: 1 in]
          n505 = Index Array(array=w1120, index=w1117) -> (element=w1119:dbl)
          n506 = Index Array(array=w1147, index (row)=w1117) -> (element=w1150:dbl[])  [unwired: 1 in]
          n507 = Index Array(array=w1125, index=w1117) -> (element=w1124:bool)
          n508 = Index Array(array=w1163, index (row)=w1117) -> (element=w1143:dbl[])  [unwired: 1 in]
          n509 = Index Array(array=w1162, index (row)=w1117) -> (element=w1144:dbl[])  [unwired: 1 in]
          n510 = Index Array(array=w1165, index (row)=w1117) -> (element=w1146:dbl[])  [unwired: 1 in]
          n511 = Index Array(array=w1164, index (row)=w1117) -> (element=w1145:dbl[])  [unwired: 1 in]
          n512 = Index Array(array=w1159, index (row)=w1117) -> (element=w1139:dbl[])  [unwired: 1 in]
          n513 = Index Array(array=w1158, index (row)=w1117) -> (element=w1138:dbl[])  [unwired: 1 in]
          n514 = Index Array(array=w1155, index (row)=w1117) -> (element=w1136:dbl[])  [unwired: 1 in]
          n515 = Index Array(array=w1154, index (row)=w1117) -> (element=w1135:dbl[])  [unwired: 1 in]
          n516 = Index Array(array=w1152, index (row)=w1117) -> (element=w1132:timestamp[])  [unwired: 1 in]
          n517 = Index Array(array=w1118, index=w1117) -> (element=w1116:dbl)
          n518 = property class="DigNum (strict)"(reference=w1131) -> ("Value"=w1129:dbl)  [unwired: 1 in, 2 out]
          n519 = property class="DigNum (strict)"(reference=w1130) -> ("Value"=w1128:dbl)  [unwired: 1 in, 2 out]
          n520 = call <vilib>:"Std Deviation and Variance.vi"("X"=w1146) -> ("mean"=w1142:dbl)  [unwired: 1 in, 2 out]
          n521 = call <vilib>:"Std Deviation and Variance.vi"("X"=w1145) -> ("mean"=w1141:dbl)  [unwired: 1 in, 2 out]
          n522 = call <vilib>:"Std Deviation and Variance.vi"("X"=w1136) -> ("mean"=w1134:dbl)  [unwired: 1 in, 2 out]
          n523 = Get Date/Time In Seconds() -> (seconds since 1Jan1904=w1133:timestamp)
          n524 = Subtract(x=w1129, y=w1142) -> (x-y=w1140:dbl)
          n525 = Subtract(x=w1128, y=w1141) -> (x-y=w1137:dbl)
          n526 = case shown="True" w1124 {
            tunnel: [w1178 w1197] -> w1161
            tunnel: [w1166 w1196] -> w1160
            tunnel: [w1167 w1195] -> w1157
            tunnel: [w1168 w1194] -> w1156
            tunnel: [w1169 w1193] -> w1153
            tunnel: [w1170 w1192] -> w1151
            tunnel: w1144 -> [w1176 w1191]
            tunnel: w1143 -> [w1177 w1190]
            tunnel: w1142 -> [_ w1189]
            tunnel: w1141 -> [_ w1188]
            tunnel: w1140 -> [_ w1187]
            tunnel: w1139 -> [w1175 w1186]
            tunnel: w1138 -> [w1174 w1185]
            tunnel: w1137 -> [_ w1184]
            tunnel: w1135 -> [w1173 w1183]
            tunnel: w1134 -> [_ w1182]
            tunnel: w1133 -> [w1171 w1181]
            tunnel: w1132 -> [w1172 w1180]
            frame False {
              w1179 = 0.0
              n527 = Build Array (concatenate)(w1177, w1179) -> (w1178:dbl[])
              n528 = Build Array (concatenate)(w1176, w1179) -> (w1166:dbl[])
              n529 = Build Array (concatenate)(w1175, w1179) -> (w1167:dbl[])
              n530 = Build Array (concatenate)(w1174, w1179) -> (w1168:dbl[])
              n531 = Build Array (concatenate)(w1173, w1179) -> (w1169:dbl[])
              n532 = Build Array (concatenate)(w1172, w1171) -> (w1170:timestamp[])
            }
            frame True {
              n533 = Build Array (concatenate)(w1190, w1189) -> (w1197:dbl[])
              n534 = Build Array (concatenate)(w1191, w1188) -> (w1196:dbl[])
              n535 = Build Array (concatenate)(w1186, w1187) -> (w1195:dbl[])
              n536 = Build Array (concatenate)(w1185, w1184) -> (w1194:dbl[])
              n537 = Build Array (concatenate)(w1183, w1182) -> (w1193:dbl[])
              n538 = Build Array (concatenate)(w1180, w1181) -> (w1192:timestamp[])
            }
          }
          n539 = Build Array (concatenate)(w1149, w1119) -> (w1127:dbl[])
          n540 = Build Array (concatenate)(w1150, w1116) -> (w1126:dbl[])
        }
        n541 = local write "#imgs avd so far"(0.0 ("Numeric")) -> ()
        n542 = Array Size(array=w1069) -> (size(s)=w1090:i32[])
        n543 = Index Array(array=w1090, index=1) -> (element=w1088:i32)
        "History Index" <- w1088
        n544 = call <vilib>:"Add State(s) to Queue__jki_lib_state_machine.vi"("State(s) in (\"\")"=w1078, "State(s) at Back (\"\")"="Check Move\ntdms" ("State(s) at Back (\"\")")) -> ("States Out"=w1082:string)  [unwired: 13 in]
        n545 = Unbundle By Name(w1068) -> ("Detection.img to avg"=w1065:i32)
        n546 = Initialize Array(0.0 ("element"), 12 ("dimension size"), w1065) -> (w1064:dbl[][])
        n547 = Bundle By Name(cluster=w1068, "Detection.Centroid X"=w1064, "Detection.Centroid Y"=w1064, "Mean Centroid X"=w1091, "Mean Centroid Y"=w1101, "Offset X"=w1069, "Offset Y"=w1092, "Mean Size"=w1096, "Detection.Size"=w1064, "Time"=w1093, "Motor X"=w1074, "Motor Y"=w1073) -> (w1061:T35)
        n548 = Greater?(x=w1088, y="History Size") -> (0:w1086:bool)
        n549 = Select(t="history" ("State(s) at Back (\"\")"), s=w1086, f="") -> (s? t:f=w1083:string)
        n550 = call <vilib>:"Add State(s) to Queue__jki_lib_state_machine.vi"("State(s) in (\"\")"=w1082, "State(s) at Back (\"\")"=w1083) -> ("States Out"=w1063:string)  [unwired: 13 in]
        n551 = call <vilib>:"Add State(s) to Queue__jki_lib_state_machine.vi"("State(s) in (\"\")"=w1063) -> ("States Out"=w1062:string)  [unwired: 14 in]
      }
      frame "Check Move" {
        n552 = Unbundle By Name(w1208) -> ("move properties"=w1218:T11[], "Mean Size"=w1217:dbl[][], "move properties"=w1216:T11[], "Offset X"=w1215:dbl[][], "Offset Y"=w1214:dbl[][], "active cams"=w1213:string[])
        n553 = Unbundle By Name(w1208) -> ("steps speed X"=w1207:dbl[], "steps speed Y"=w1206:dbl[])
        n554 = for {
          tunnel: w1216 -> [w1258]
          tunnel: w1215 -> [w1256]
          tunnel: w1214 -> [w1254]
          tunnel: w1217 -> [w1262]
          tunnel: [w1272] -> w1202 mode=indexing
          tunnel: [w1268] -> w1200 mode=indexing
          tunnel: w1213 -> [w1263] mode=indexing
          tunnel: [w1289] -> w1219 mode=indexing
          tunnel: [w1288] -> w1211 mode=indexing
          tunnel: w1218 -> [w1261]
          tunnel: [w1240] -> w1203 mode=indexing
          tunnel: [w1252] -> w1201 mode=indexing
          tunnel: "Speedmode" -> [w1266]
          tunnel: w1210 -> [w1264]
          shift-right: [w1245] -> w1205
          shift-left: w1207 -> [w1250]
          shift-right: [w1244] -> w1204
          shift-left: w1206 -> [w1249]
          tunnel: [w1241] -> w1198 mode=indexing
          n555 = call-poly <userlib>:"Filter 1D Array__ogtk.vi"("items to filter"=w1263, "array"=w1264) -> ("filtered item indices"=w1265:i32[])  [unwired: 4 in, 1 out]
          n556 = Index Array(array=w1265) -> (element=w1248:i32)  [unwired: 1 in]
          n557 = Index Array(array=w1261, index=w1248) -> (element=w1260:T11)
          n558 = Index Array(array=w1262, index (row)=w1248) -> (element=w1259:dbl[])  [unwired: 1 in]
          n559 = Index Array(array=w1258, index=w1248) -> (element=w1257:T11)
          n560 = Index Array(array=w1256, index (row)=w1248) -> (element=w1255:dbl[])  [unwired: 1 in]
          n561 = Index Array(array=w1254, index (row)=w1248) -> (element=w1253:dbl[])  [unwired: 1 in]
          n562 = Unbundle By Name(w1257) -> ("Tolerance [%]"=w1282:dbl)
          n563 = Reverse 1D Array(array=w1255) -> (reversed array=w1287:dbl[])
          n564 = Reverse 1D Array(array=w1253) -> (reversed array=w1286:dbl[])
          n565 = Reverse 1D Array(array=w1259) -> (reversed array=w1281:dbl[])
          n566 = Unbundle By Name(w1260) -> ("Stepsize"=w1243:dbl, "enable feedback"=w1271:bool)
          n567 = Index Array(array=w1287) -> (element=w1285:dbl)  [unwired: 1 in]
          n568 = Index Array(array=w1286) -> (element=w1284:dbl)  [unwired: 1 in]
          n569 = Index Array(array=w1281) -> (element=w1280:dbl)  [unwired: 1 in]
          n570 = Absolute Value(x=w1285) -> (abs(x)=w1251:dbl)
          n571 = Absolute Value(x=w1284) -> (abs(x)=w1267:dbl)
          n572 = Square Root(x=w1280) -> (sqrt(x)=w1279:dbl)
          n573 = Divide(x=w1282, y=100.0) -> (x/y=w1242:dbl)
          n574 = Multiply(x=w1279, y=w1242) -> (x*y=w1241:dbl)
          n575 = Not Equal To 0?(x=w1267) -> (x != 0?=w1269:bool)
          n576 = Not Equal To 0?(x=w1251) -> (x != 0?=w1274:bool)
          n577 = Greater Or Equal?(x=w1251, y=w1241) -> (x >= y?=w1273:bool)
          n578 = Greater Or Equal?(x=w1267, y=w1241) -> (x >= y?=w1270:bool)
          n579 = call "speedmode.vi"("offset X"=w1251, "offset Y"=w1267, "beamsize x tolerance"=w1241, "Speedmode @"=w1266, "step size"=w1243) -> ("steps speed Y"=w1246:dbl, "steps speed X"=w1247:dbl, "speedmode X"=w1240:bool, "speedmode Y"=w1252:bool)  [unwired: 3 in]
          n580 = Compound Arithmetic op=AND(w1271, w1274, w1273) -> (w1272:bool)
          n581 = Compound Arithmetic op=AND(w1271, w1270, w1269) -> (w1268:bool)
          n582 = Boolean To (0,1)(Boolean=w1268) -> (0, 1=w1275:i16)
          n583 = Multiply(x=w1275, y=w1267) -> (x*y=w1276:dbl)
          n584 = Boolean To (0,1)(Boolean=w1272) -> (0, 1=w1278:i16)
          n585 = Replace Array Subset(array=w1250, new element=w1247, index=w1248) -> (w1245:dbl[])
          n586 = Replace Array Subset(array=w1249, new element=w1246, index=w1248) -> (w1244:dbl[])
          n587 = Multiply(x=w1278, y=w1251) -> (x*y=w1277:dbl)
          n588 = Bundle(w1276, "GUIdevice 8"=w1263) -> (w1288:cluster{dbl, "GUIdevice 8":string})  [unwired: 1 in]
          n589 = Bundle(w1277, "GUIdevice 8"=w1263) -> (w1289:cluster{dbl, "GUIdevice 8":string})  [unwired: 1 in]
        }
        "required X" <- w1202
        "required Y" <- w1200
        "tolerances (pix)" <- w1198
        n590 = case shown="False" "Align" {
          tunnel: w1219 -> [w1295 w1300]
          tunnel: w1211 -> [w1294 w1297]
          tunnel: [w1293 w1299] -> w1222
          tunnel: [w1292 w1296] -> w1221
          frame False {
            n591 = Sort 1D Array(array=w1294) -> (sorted array=w1291:cluster{dbl, "GUIdevice 8":string}[])
            n592 = Sort 1D Array(array=w1295) -> (sorted array=w1290:cluster{dbl, "GUIdevice 8":string}[])
            n593 = Reverse 1D Array(array=w1291) -> (reversed array=w1292:cluster{dbl, "GUIdevice 8":string}[])
            n594 = Reverse 1D Array(array=w1290) -> (reversed array=w1293:cluster{dbl, "GUIdevice 8":string}[])
          }
          frame True {
            w1298 = cluster{dbl, "GUIdevice 8":string}[] [] ("Array")
            n595 = for {
              shift-right: [w1310] -> w1299
              shift-left: w1298 -> [w1312]
              tunnel: w1300 -> [w1311] mode=indexing
              n596 = Unbundle(w1311) -> (w1314:dbl)  [unwired: 1 out]
              n597 = Not Equal To 0?(x=w1314) -> (x != 0?=w1313:bool)
              n598 = case shown="True" w1313 {
                tunnel: w1312 -> [w1315 w1318]
                tunnel: w1311 -> [_ w1317]
                tunnel: [w1315 w1316] -> w1310
                frame False {
                }
                frame True {
                  n599 = Build Array (concatenate)(w1318, w1317) -> (w1316:cluster{dbl, "GUIdevice 8":string}[])
                }
              }
            }
            n600 = for {
              shift-right: [w1301] -> w1296
              shift-left: w1298 -> [w1303]
              tunnel: w1297 -> [w1302] mode=indexing
              n601 = Unbundle(w1302) -> (w1305:dbl)  [unwired: 1 out]
              n602 = Not Equal To 0?(x=w1305) -> (x != 0?=w1304:bool)
              n603 = case shown="True" w1304 {
                tunnel: w1303 -> [w1306 w1309]
                tunnel: w1302 -> [_ w1308]
                tunnel: [w1306 w1307] -> w1301
                frame False {
                }
                frame True {
                  n604 = Build Array (concatenate)(w1309, w1308) -> (w1307:cluster{dbl, "GUIdevice 8":string}[])
                }
              }
            }
          }
        }
        n605 = call <vilib>:"Add State(s) to Queue__jki_lib_state_machine.vi"("State(s) in (\"\")"=w1225) -> ("States Out"=w1224:string)  [unwired: 14 in]
        n606 = Bundle By Name(cluster=w1208, "speedmode X"=w1203, "speedmode Y"=w1201, "steps speed X"=w1205, "steps speed Y"=w1204) -> (w1209:T35)
        n607 = Index Array(array=w1221) -> (element=w1226:cluster{dbl, "GUIdevice 8":string})  [unwired: 1 in]
        n608 = Index Array(array=w1222) -> (element=w1227:cluster{dbl, "GUIdevice 8":string})  [unwired: 1 in]
        n609 = Empty Array?(array=w1221) -> (empty?=w1229:bool)
        n610 = Unbundle(w1227) -> (w1235:dbl)  [unwired: 1 out]
        n611 = Unbundle(w1226) -> (w1231:dbl)  [unwired: 1 out]
        n612 = Unbundle By Name(w1209) -> ("Feedback global"=w1236:bool)
        n613 = Empty Array?(array=w1222) -> (empty?=w1233:bool)
        n614 = property on="autodetect" class="Bool (strict)"("Value"=FALSE ("autodetect")) -> ()  [unwired: 2 in, 2 out]
        n615 = Equal To 0?(x=w1235) -> (x = 0?=w1234:bool)
        n616 = Equal To 0?(x=w1231) -> (x = 0?=w1230:bool)
        n617 = Or(x=w1234, y=w1233) -> (x .or. y?=w1232:bool)
        n618 = Or(x=w1230, y=w1229) -> (x .or. y?=w1228:bool)
        n619 = case shown="True" w1236 {
          tunnel: w1232 -> [_ w1337]
          tunnel: w1222 -> [_ w1336]
          tunnel: w1228 -> [_ w1334]
          tunnel: w1221 -> [_ w1333]
          tunnel: w1224 -> [w1319 w1332]
          tunnel: [w1319 w1331] -> w1237
          tunnel: w1203 -> [_ w1330]
          tunnel: w1202 -> [_ w1329]
          tunnel: w1201 -> [_ w1328]
          tunnel: w1200 -> [_ w1327]
          frame False {
          }
          frame True {
            n620 = case shown="False" w1337 {
              tunnel: w1336 -> [w1361 _]
              tunnel: w1332 -> [w1357 w1362]
              tunnel: [w1355 w1362] -> w1335
              frame False {
                n621 = Index Array(array=w1361) -> (element=w1360:cluster{dbl, "GUIdevice 8":string})  [unwired: 1 in]
                n622 = Unbundle By Name(w1360) -> ("GUIdevice 8"=w1359:string)
                n623 = call <vilib>:"Build State String with Arguments__jki_lib_state_machine.vi"("Arguments (\"\")"=w1359, "State"="Move X") -> ("State with Arguments"=w1356:string)  [unwired: 4 in]
                n624 = call <vilib>:"Add State(s) to Queue__jki_lib_state_machine.vi"("State(s) in (\"\")"=w1357, "State(s) at Back (\"\")"=w1356) -> ("States Out"=w1355:string)  [unwired: 13 in]
              }
              frame True {
              }
            }
            n625 = case shown="False" w1334 {
              tunnel: w1333 -> [w1353 _]
              tunnel: w1335 -> [w1349 w1354]
              tunnel: [w1347 w1354] -> w1331
              frame False {
                n626 = Index Array(array=w1353) -> (element=w1352:cluster{dbl, "GUIdevice 8":string})  [unwired: 1 in]
                n627 = Unbundle By Name(w1352) -> ("GUIdevice 8"=w1351:string)
                n628 = call <vilib>:"Build State String with Arguments__jki_lib_state_machine.vi"("Arguments (\"\")"=w1351, "State"="Move Y") -> ("State with Arguments"=w1348:string)  [unwired: 4 in]
                n629 = call <vilib>:"Add State(s) to Queue__jki_lib_state_machine.vi"("State(s) in (\"\")"=w1349, "State(s) at Back (\"\")"=w1348) -> ("States Out"=w1347:string)  [unwired: 13 in]
              }
              frame True {
              }
            }
            n630 = for {
              tunnel: w1330 -> [w1346] mode=indexing
              tunnel: w1329 -> [w1345] mode=indexing
              tunnel: [w1344] -> w1326 mode=indexing
              n631 = And(x=w1346, y=w1345) -> (x .and. y?=w1344:bool)
            }
            n632 = for {
              tunnel: w1328 -> [w1343] mode=indexing
              tunnel: w1327 -> [w1342] mode=indexing
              tunnel: [w1341] -> w1325 mode=indexing
              n633 = And(x=w1343, y=w1342) -> (x .and. y?=w1341:bool)
            }
            n634 = Or Array Elements(Boolean array=w1326) -> (logical OR=w1324:bool)
            n635 = Or Array Elements(Boolean array=w1325) -> (logical OR=w1323:bool)
            n636 = Or(x=w1324, y=w1323) -> (x .or. y?=w1322:bool)
            n637 = property on="alarms" class="Bool (strict)"() -> ("Value"=w1321:bool)  [unwired: 2 in, 2 out]
            n638 = And(x=w1321, y=w1322) -> (x .and. y?=w1320:bool)
            n639 = case shown="True" w1320 {
              frame False {
              }
              frame True {
                n640 = call <vilib>:"Beep.vi"("use system alert? (T)"=FALSE, "duration (msec)"=u32 750, "frequency (Hz)"=u32 750) -> ()  [unwired: 9 in]
              }
            }
          }
        }
        n641 = call <vilib>:"Add State(s) to Queue__jki_lib_state_machine.vi"("State(s) in (\"\")"=w1224, "State(s) at Back (\"\")"=w1237) -> ("States Out"=w1239:string)  [unwired: 13 in]
      }
      frame "Move X" {
        # "Your code here.\n(You can make a copy of, or modify, this frame)"
        n642 = Unbundle By Name(w1376) -> ("Offset X"=w1388:dbl[][])
        n643 = call-poly <userlib>:"Filter 1D Array__ogtk.vi"("items to filter"=w1382, "array"=w1389) -> ("filtered item indices"=w1385:i32[])  [unwired: 4 in, 1 out]
        n644 = Unbundle By Name(w1376) -> ("dev var alias arrays.dev variable alias Motors X"=w1378:string[][])
        n645 = Unbundle By Name(w1376) -> ("move properties"=w1381:T11[])
        n646 = for {
          tunnel: w1385 -> [w1417] mode=indexing
          tunnel: w1381 -> [w1421]
          shift-right: [w1416] -> w1383
          shift-left: i32[] [] ("filtered item indices") -> [w1419]
          n647 = Index Array(array=w1421, index=w1417) -> (element=w1420:T11)
          n648 = Unbundle By Name(w1420) -> ("enable feedback"=w1418:bool)
          n649 = case shown="True" w1418 {
            tunnel: w1419 -> [w1422 w1425]
            tunnel: w1417 -> [_ w1424]
            tunnel: [w1422 w1423] -> w1416
            frame False {
            }
            frame True {
              n650 = Build Array (concatenate)(w1425, w1424) -> (w1423:i32[])
            }
          }
        }
        n651 = Index Array(array=w1383) -> (element=w1373:i32)  [unwired: 1 in]
        n652 = call "Beampointing get set motor position.vi"("Active CCD"=w1373, "error in (no error)"=w1371, "get or set"=enum16{"get", "set"}."get", "dev variable alias Motors X"=w1378) -> ("error out"=w1369:errorcluster, "Actual Position"=w1377:dbl)  [unwired: 6 in]
        n653 = Index Array(array=w1388, index (row)=w1373) -> (element=w1387:dbl[])  [unwired: 1 in]
        n654 = Reverse 1D Array(array=w1387) -> (reversed array=w1386:dbl[])
        n655 = Index Array(array=w1386) -> (element=w1367:dbl)  [unwired: 1 in]
        n656 = Index Array(array=w1381, index=w1373) -> (element=w1363:T11)
        n657 = Unbundle By Name(w1363) -> ("Invert Direction X"=w1368:bool, "enable feedback"=w1370:bool)
        n658 = local read "Align"() -> (w1365:bool)
        n659 = call "relative move from offset and calibration.vi"("Align"=w1365, "axis"=enum16{"x", "y"}."x", "Offset"=w1367, "element"=w1363) -> ("relative move out"=w1366:dbl)  [unwired: 7 in]
        n660 = case shown="No Error" w1369 {
          selector: w1369 -> [w1393 w1414]
          tunnel: w1368 -> [_ _]
          tunnel: w1370 -> [w1403 _]
          tunnel: w1378 -> [w1402 _]
          tunnel: w1377 -> [w1401 _]
          tunnel: w1376 -> [w1400 w1415]
          tunnel: [w1396 w1415] -> w1375
          tunnel: w1373 -> [w1395 _]
          tunnel: w1366 -> [w1394 _]
          tunnel: [w1392 w1414] -> w1372
          frame No Error {
            n661 = case shown="True" w1403 {
              tunnel: w1394 -> [_ w1413]
              tunnel: w1402 -> [_ w1411]
              tunnel: w1395 -> [_ w1410]
              tunnel: w1401 -> [w1404 w1408]
              tunnel: [w1404 w1407] -> w1397
              tunnel: w1393 -> [_ w1406]
              tunnel: [_ w1405] -> w1392
              frame False {
              }
              frame True {
                n662 = Add(x=w1408, y=w1413) -> (x+y=w1409:dbl)
                n663 = call "Beampointing get set motor position.vi"("Active CCD"=w1410, "error in (no error)"=w1406, "Set position"=w1409, "get or set"=enum16{"get", "set"}."set", "dev variable alias Motors X"=w1411) -> ("error out"=w1405:errorcluster, "Actual Position"=w1407:dbl)  [unwired: 5 in]
              }
            }
            n664 = Unbundle By Name(w1400) -> ("Motor positions.Positions x"=w1399:dbl[])
            n665 = Replace Array Subset(array=w1399, new element=w1397, index=w1395) -> (w1398:dbl[])
            n666 = Bundle By Name(cluster=w1400, "Motor positions.Positions x"=w1398) -> (w1396:T35)
          }
          frame Error {
          }
        }
        n667 = call <vilib>:"Build State String with Arguments__jki_lib_state_machine.vi"("Arguments (\"\")"=w1382, "State"="Wait" ("State(s) in Front (\"\")")) -> ()  [unwired: 4 in, 1 out]
        n668 = call <vilib>:"Add State(s) to Queue__jki_lib_state_machine.vi"("State(s) in (\"\")"=w1391) -> ("States Out"=w1390:string)  [unwired: 14 in]
        "Moving X" <- w1382
      }
      frame "ManMove X" {
        # "Your code here.\n(You can make a copy of, or modify, this frame)"
        n669 = Unbundle By Name(w1431) -> ("dev var alias arrays.dev variable alias Motors X"=w1435:string[][])
        n670 = Unbundle By Name(w1431) -> ("move properties"=w1445:T11[], "active ccd"=w1428:i32, "active cams"=w1443:string[])  [unwired: 1 out]
        n671 = Index Array(array=w1443, index=w1428) -> (element=w1441:string)
        n672 = call "Beampointing get set motor position.vi"("Active CCD"=w1428, "get or set"=enum16{"get", "set"}."get", "dev variable alias Motors X"=w1435) -> ("error out"=w1426:errorcluster, "Actual Position"=w1436:dbl)  [unwired: 7 in]
        n673 = Index Array(array=w1445, index=w1428) -> (element=w1447:T11)
        n674 = Unbundle By Name(w1447) -> ("Invert Direction X"=w1446:bool)
        n675 = call <vilib>:"Build State String with Arguments__jki_lib_state_machine.vi"("Arguments (\"\")"=w1441, "State"="Wait" ("State(s) in Front (\"\")")) -> ()  [unwired: 4 in, 1 out]
        n676 = call <vilib>:"Add State(s) to Queue__jki_lib_state_machine.vi"("State(s) in Front (\"\")"="RestartAveraging" ("State(s) in Front (\"\")"), "State(s) in (\"\")"=w1450) -> ("States Out"=w1449:string)  [unwired: 13 in]
        n677 = case shown="\"Left\", Default" w1440 {
          tunnel: w1446 -> [w1454 w1464]
          tunnel: "StepSize" -> [w1453 w1463]
          tunnel: w1436 -> [w1452 w1462]
          tunnel: [w1451 w1461] -> w1434
          frame "Right" {
            n678 = case shown="False" w1454 {
              tunnel: w1452 -> [w1457 w1460]
              tunnel: w1453 -> [w1456 w1459]
              tunnel: [w1455 w1458] -> w1451
              frame False {
                n679 = Add(x=w1457, y=w1456) -> (x+y=w1455:dbl)
              }
              frame True {
                n680 = Subtract(x=w1460, y=w1459) -> (x-y=w1458:dbl)
              }
            }
          }
          frame "Left", Default {
            n681 = case shown="True" w1464 {
              tunnel: w1462 -> [w1467 w1470]
              tunnel: w1463 -> [w1466 w1469]
              tunnel: [w1465 w1468] -> w1461
              frame False {
                n682 = Subtract(x=w1467, y=w1466) -> (x-y=w1465:dbl)
              }
              frame True {
                n683 = Add(x=w1470, y=w1469) -> (x+y=w1468:dbl)
              }
            }
          }
        }
        n684 = call "Beampointing get set motor position.vi"("Active CCD"=w1428, "error in (no error)"=w1426, "Set position"=w1434, "get or set"=enum16{"get", "set"}."set", "dev variable alias Motors X"=w1435) -> ("Actual Position"=w1429:dbl)  [unwired: 5 in, 1 out]
        n685 = Unbundle By Name(w1431) -> ("Motor positions.Positions x"=w1433:dbl[])
        n686 = Replace Array Subset(array=w1433, new element=w1429, index=w1428) -> (w1432:dbl[])
        n687 = Bundle By Name(cluster=w1431, "Motor positions.Positions x"=w1432) -> (w1430:T35)
      }
      frame "ManMove Y" {
        # "Your code here.\n(You can make a copy of, or modify, this frame)"
        n688 = Equal?(x=w1485, y="Down") -> ()  [unwired: 1 out]
        n689 = Unbundle By Name(w1474) -> ("active cams"=w1487:string[], "move properties"=w1491:T11[], "active ccd"=w1475:i32)
        n690 = Unbundle By Name(w1474) -> ("dev var alias arrays.dev variable alias Motors Y"=w1483:string[][])
        n691 = Index Array(array=w1487, index=w1475) -> (element=w1486:string)
        n692 = call "Beampointing get set motor position.vi"("Active CCD"=w1475, "get or set"=enum16{"get", "set"}."get", "dev variable alias Motors X"=w1483) -> ("Actual Position"=w1479:dbl)  [unwired: 7 in, 1 out]
        n693 = Index Array(array=w1491, index=w1475) -> (element=w1492:T11)
        n694 = property on="StepSize" class="DigNum (strict)"() -> ("Value"=w1488:dbl)  [unwired: 2 in, 2 out]
        n695 = Unbundle By Name(w1492) -> ("Invert Direction Y"=w1489:bool)
        n696 = call <vilib>:"Build State String with Arguments__jki_lib_state_machine.vi"("Arguments (\"\")"=w1486, "State"="Wait" ("State(s) in Front (\"\")")) -> ()  [unwired: 4 in, 1 out]
        n697 = case shown="\"Up\", Default" w1485 {
          tunnel: w1489 -> [w1499 w1509]
          tunnel: w1488 -> [w1498 w1508]
          tunnel: [w1497 w1506] -> w1480
          tunnel: w1479 -> [w1496 w1507]
          frame "Down" {
            n698 = case shown="False" w1499 {
              tunnel: w1496 -> [w1502 w1505]
              tunnel: w1498 -> [w1501 w1504]
              tunnel: [w1500 w1503] -> w1497
              frame False {
                n699 = Add(x=w1502, y=w1501) -> (x+y=w1500:dbl)
              }
              frame True {
                n700 = Subtract(x=w1505, y=w1504) -> (x-y=w1503:dbl)
              }
            }
          }
          frame "Up", Default {
            n701 = case shown="False" w1509 {
              tunnel: w1507 -> [w1512 w1515]
              tunnel: w1508 -> [w1511 w1514]
              tunnel: [w1510 w1513] -> w1506
              frame False {
                n702 = Subtract(x=w1512, y=w1511) -> (x-y=w1510:dbl)
              }
              frame True {
                n703 = Add(x=w1515, y=w1514) -> (x+y=w1513:dbl)
              }
            }
          }
        }
        n704 = call <vilib>:"Add State(s) to Queue__jki_lib_state_machine.vi"("State(s) in Front (\"\")"="RestartAveraging" ("State(s) in Front (\"\")"), "State(s) in (\"\")"=w1495) -> ("States Out"=w1494:string)  [unwired: 13 in]
        n705 = call "Beampointing get set motor position.vi"("Active CCD"=w1475, "Set position"=w1480, "get or set"=enum16{"get", "set"}."set", "dev variable alias Motors X"=w1483) -> ("Actual Position"=w1476:dbl)  [unwired: 6 in, 1 out]
        n706 = Unbundle By Name(w1474) -> ("Motor positions.Positions y"=w1478:dbl[])
        n707 = Replace Array Subset(array=w1478, new element=w1476, index=w1475) -> (w1477:dbl[])
        n708 = Bundle By Name(cluster=w1474, "Motor positions.Positions y"=w1477) -> (w1473:T35)
      }
      frame "Move Y" {
        # "Your code here.\n(You can make a copy of, or modify, this frame)"
        n709 = Unbundle By Name(w1527) -> ("dev var alias arrays.dev variable alias Motors Y"=w1528:string[][])
        n710 = Unbundle By Name(w1527) -> ("Offset Y"=w1540:dbl[][])
        n711 = call-poly <userlib>:"Filter 1D Array__ogtk.vi"("items to filter"=w1532, "array"=w1541) -> ("filtered item indices"=w1536:i32[])  [unwired: 4 in, 1 out]
        n712 = Unbundle By Name(w1527) -> ("move properties"=w1534:T11[])
        n713 = for {
          tunnel: w1536 -> [w1567] mode=indexing
          tunnel: w1534 -> [w1571]
          shift-right: [w1566] -> w1535
          shift-left: i32[] [] ("filtered item indices") -> [w1569]
          n714 = Index Array(array=w1571, index=w1567) -> (element=w1570:T11)
          n715 = Unbundle By Name(w1570) -> ("enable feedback"=w1568:bool)
          n716 = case shown="True" w1568 {
            tunnel: w1569 -> [w1572 w1575]
            tunnel: w1567 -> [_ w1574]
            tunnel: [w1572 w1573] -> w1566
            frame False {
            }
            frame True {
              n717 = Build Array (concatenate)(w1575, w1574) -> (w1573:i32[])
            }
          }
        }
        n718 = Index Array(array=w1535) -> (element=w1525:i32)  [unwired: 1 in]
        n719 = Index Array(array=w1540, index (row)=w1525) -> (element=w1539:dbl[])  [unwired: 1 in]
        n720 = Reverse 1D Array(array=w1539) -> (reversed array=w1538:dbl[])
        n721 = call "Beampointing get set motor position.vi"("Active CCD"=w1525, "error in (no error)"=w1521, "get or set"=enum16{"get", "set"}."get", "dev variable alias Motors X"=w1528) -> ("error out"=w1523:errorcluster, "Actual Position"=w1529:dbl)  [unwired: 6 in]
        n722 = Index Array(array=w1538) -> (element=w1520:dbl)  [unwired: 1 in]
        n723 = Index Array(array=w1534, index=w1525) -> (element=w1517:T11)
        n724 = Unbundle By Name(w1517) -> ("enable feedback"=w1537:bool)
        n725 = local read "Align"() -> (w1516:bool)
        n726 = call "relative move from offset and calibration.vi"("Align"=w1516, "axis"=enum16{"x", "y"}."y", "Offset"=w1520, "element"=w1517) -> ("relative move out"=w1519:dbl)  [unwired: 7 in]
        n727 = case shown="No Error" w1523 {
          selector: w1523 -> [_ w1564]
          tunnel: w1537 -> [w1554 _]
          tunnel: w1529 -> [w1553 _]
          tunnel: w1528 -> [w1552 _]
          tunnel: w1527 -> [w1549 w1565]
          tunnel: [w1548 w1565] -> w1526
          tunnel: w1525 -> [w1546 _]
          tunnel: w1519 -> [w1545 _]
          tunnel: [w1544 w1564] -> w1522
          frame No Error {
            n728 = case shown="True" w1554 {
              tunnel: w1545 -> [_ w1563]
              tunnel: w1553 -> [w1555 w1562]
              tunnel: w1552 -> [_ w1559]
              tunnel: w1546 -> [_ w1558]
              tunnel: [w1555 w1557] -> w1547
              tunnel: [_ w1556] -> w1544
              frame False {
              }
              frame True {
                n729 = Add(x=w1562, y=w1563) -> (x+y=w1561:dbl)
                n730 = call "Beampointing get set motor position.vi"("Active CCD"=w1558, "Set position"=w1561, "get or set"=enum16{"get", "set"}."set", "dev variable alias Motors X"=w1559) -> ("error out"=w1556:errorcluster, "Actual Position"=w1557:dbl)  [unwired: 6 in]
              }
            }
            n731 = Unbundle By Name(w1549) -> ("Motor positions.Positions y"=w1551:dbl[])
            n732 = Replace Array Subset(array=w1551, new element=w1547, index=w1546) -> (w1550:dbl[])
            n733 = Bundle By Name(cluster=w1549, "Motor positions.Positions y"=w1550) -> (w1548:T35)
          }
          frame Error {
          }
        }
        n734 = call <vilib>:"Build State String with Arguments__jki_lib_state_machine.vi"("Arguments (\"\")"=w1532, "State"="Wait" ("State(s) in Front (\"\")")) -> ()  [unwired: 4 in, 1 out]
        n735 = call <vilib>:"Add State(s) to Queue__jki_lib_state_machine.vi"("State(s) in (\"\")"=w1543) -> ("States Out"=w1542:string)  [unwired: 14 in]
        "Moving Y" <- w1532
      }
      frame "Wait" {
        # "Your code here.\n(You can make a copy of, or modify, this frame)"
        n736 = disable-structure shown="Disabled" {
          disable-tunnel: w1581 -> [w1595 _]
          disable-tunnel: w1580 -> [w1594 _]
          disable-tunnel: w1579 -> [w1593 _]
          disable-tunnel: w1578 -> [w1591 w1615]
          disable-tunnel: [w1590 w1615] -> w1577
          frame Disabled {
            n737 = call-poly <userlib>:"Filter 1D Array__ogtk.vi"("items to filter"=w1593, "array"=w1594) -> ("filtered item indices"=w1592:i32[])  [unwired: 4 in, 1 out]
            n738 = Index Array(array=w1592) -> (element=w1589:i32)  [unwired: 1 in]
            n739 = flat-sequence {
              tunnel: T30."Disabled and Grayed Out" ("Disabled") -> [w1596]
              tunnel: w1591 -> [w1604]
              tunnel: [w1603] -> w1590
              tunnel: w1589 -> [w1602]
              tunnel: w1588 -> [w1601]
              tunnel: T30."Enabled" ("Disabled") -> [w1614]
              frame #0 {
                n740 = property on="Right" class="Bool (strict)"("DisabledEnum"=w1596) -> ()  [unwired: 2 in, 2 out]
                n741 = property on="Up" class="Bool (strict)"("DisabledEnum"=w1596) -> ()  [unwired: 2 in, 2 out]
                n742 = property on="Left" class="Bool (strict)"("DisabledEnum"=w1596) -> ()  [unwired: 2 in, 2 out]
                n743 = property on="Down" class="Bool (strict)"("DisabledEnum"=w1596) -> ()  [unwired: 2 in, 2 out]
                n744 = property on="StepSize" class="DigNum (strict)"("DisabledEnum"=w1596) -> ()  [unwired: 2 in, 2 out]
              }
              frame #1 {
                n745 = Wait (ms)(milliseconds to wait=u32 1500) -> ()  [unwired: 1 out]
              }
              frame #2 {
                n746 = property on="Moving Y" class="Str"("Value"="") -> ()  [unwired: 2 in, 2 out]
                n747 = property on="Moving X" class="Str"("Value"="") -> ()  [unwired: 2 in, 2 out]
              }
              frame #3 {
                n748 = Equal?(x=w1601, y=w1602) -> (x = y?=w1600:bool)
                n749 = case shown="True" w1600 {
                  tunnel: _ -> [_ w1611]
                  tunnel: w1604 -> [w1605 w1608]
                  tunnel: [w1605 w1606] -> w1603
                  frame False {
                  }
                  frame True {
                    n750 = Unbundle By Name(w1611) -> ("Ref X"=w1610, "Ref Y"=w1609)
                    n751 = property class="DigNum (strict)"(reference=w1610, error in=w1608) -> (error out=w1607:errorcluster, "Value"=w1613:dbl)  [unwired: 1 out]
                    n752 = property class="DigNum (strict)"(reference=w1609, error in=w1607) -> (error out=w1606:errorcluster, "Value"=w1612:dbl)  [unwired: 1 out]
                    n753 = property on="Position 1" class="DigNum (strict)"("Value"=w1613) -> ()  [unwired: 2 in, 2 out]
                    n754 = property on="Position 2" class="DigNum (strict)"("Value"=w1612) -> ()  [unwired: 2 in, 2 out]
                  }
                }
              }
              frame #4 {
                n755 = property on="Right" class="Bool (strict)"("DisabledEnum"=w1614) -> ()  [unwired: 2 in, 2 out]
                n756 = property on="Up" class="Bool (strict)"("DisabledEnum"=w1614) -> ()  [unwired: 2 in, 2 out]
                n757 = property on="Left" class="Bool (strict)"("DisabledEnum"=w1614) -> ()  [unwired: 2 in, 2 out]
                n758 = property on="Down" class="Bool (strict)"("DisabledEnum"=w1614) -> ()  [unwired: 2 in, 2 out]
                n759 = property on="StepSize" class="DigNum (strict)"("DisabledEnum"=w1614) -> ()  [unwired: 2 in, 2 out]
              }
            }
            n760 = Unbundle By Name(w1595) -> ("active ccd"=w1588:i32)
          }
          frame Enabled {
          }
        }
        n761 = call <vilib>:"Add State(s) to Queue__jki_lib_state_machine.vi"("State(s) in (\"\")"=w1585) -> ("States Out"=w1584:string)  [unwired: 14 in]
        n762 = local read "Mean Centroid X"() -> (w1582:dbl[][])
        n763 = Bundle By Name(cluster=w1581, "Mean Centroid X"=w1582, "Mean Centroid Y"=w1582) -> (w1583:T35)
      }
      frame "RestartAveraging" {
        # "clear arrays"
        n764 = Unbundle By Name(w1622) -> ("Detection"=w1623:T32)
        n765 = Unbundle By Name(w1623) -> ("img to avg"=w1625:i32)
        n766 = Decrement(x=w1625) -> (x-1=w1620:i32)
        n767 = Initialize Array(0.0 ("element"), 12 ("dimension size"), w1620) -> (w1617:dbl[][])
        n768 = Bundle By Name(cluster=w1623, "Centroid X"=w1617, "Centroid Y"=w1617, "Size"=w1617) -> (w1624:T32)
        n769 = Bundle By Name(cluster=w1622, "Detection"=w1624) -> (w1621:T35)
        n770 = local write "#imgs avd so far"(0.0 ("#imgs avd so far")) -> ()
        n771 = call <vilib>:"Add State(s) to Queue__jki_lib_state_machine.vi"("State(s) in (\"\")"=w1629) -> ("States Out"=w1628:string)  [unwired: 14 in]
      }
      frame "---------------Statistics--------------" {
        # "Template Separator\n(You can make a copy of, or modify, this frame)"
        n772 = call <vilib>:"Add State(s) to Queue__jki_lib_state_machine.vi"("State(s) in (\"\")"=w1634) -> ("States Out"=w1633:string)  [unwired: 14 in]
      }
      frame "Save Stats" {
        # "Your code here.\n(You can make a copy of, or modify, this frame)"
        n773 = disable-structure shown="Disabled" {
          disable-tunnel: w1641 -> [w1645 _]
          disable-tunnel: [w1644 _] -> w1640
          disable-tunnel: _ -> [w1643 _]
          disable-tunnel: w1637 -> [w1642 _]
          frame Disabled {
            n774 = for {
              tunnel: w1643 -> [w1648] mode=indexing
              tunnel: w1642 -> [w1647] mode=indexing
              n775 = Empty String/Path?(string/path=w1647) -> (empty?=w1646:bool)
              n776 = case shown="False" w1646 {
                tunnel: w1648 -> [w1654 _]
                tunnel: w1647 -> [w1652 _]
                frame False {
                  n777 = Index Array(array=w1654, index #1=0 ("index"), index #2=1 ("index"), index #3=2 ("index"), index #4=3 ("index")) -> (element #1=w1689, element #2=w1683, element #3=w1682, element #4=w1681)  [unwired: 1 in, 1 out]
                  n778 = Concatenate Strings(w1652, ".dat" ("string")) -> (w1650:string)
                  n779 = Unbundle(w1689) -> (w1688, w1666)
                  n780 = Unbundle(w1683) -> (w1657)  [unwired: 1 out]
                  n781 = Unbundle(w1682) -> (w1656)  [unwired: 1 out]
                  n782 = Unbundle(w1681) -> (w1655)  [unwired: 1 out]
                  n783 = Build Path(base path="save path", name or relative path=w1650) -> (appended path=w1649:path)
                  n784 = for {
                    tunnel: w1688 -> [w1691]
                    tunnel: [w1690] -> w1664 mode=indexing
                    n785 = Format Date/Time String(time format string (%c)="%Y%m%d%H%M%S", seconds (now)=w1691) -> (date/time string=w1690:string)  [unwired: 1 in]
                  }
                  n786 = Array Size(array=w1666) -> (size(s)=w1667:i32)
                  n787 = Number To Fractional String(number=w1666) -> (F-format string=w1663:string)  [unwired: 3 in]
                  n788 = Number To Fractional String(number=w1657) -> (F-format string=w1660:string)  [unwired: 3 in]
                  n789 = Number To Fractional String(number=w1656) -> (F-format string=w1659:string)  [unwired: 3 in]
                  n790 = Number To Fractional String(number=w1655) -> (F-format string=w1658:string)  [unwired: 3 in]
                  n791 = Initialize Array("", w1667, 5 ("dimension size")) -> (w1665:string[][])
                  n792 = Insert Into Array(array=w1665, index (col)=0 ("disabled index (col)"), new element=w1664) -> (w1675:string[][])  [unwired: 1 in]
                  n793 = Insert Into Array(array=w1675, index (col)=1 ("disabled index (col)"), new element=w1663) -> (w1674:string[][])  [unwired: 1 in]
                  n794 = Insert Into Array(array=w1674, index (col)=2 ("disabled index (col)"), new element=w1660) -> (w1678:string[][])  [unwired: 1 in]
                  n795 = Insert Into Array(array=w1678, index (col)=3 ("disabled index (col)"), new element=w1659) -> (w1679:string[][])  [unwired: 1 in]
                  n796 = Insert Into Array(array=w1679, index (col)=4 ("disabled index (col)"), new element=w1658) -> (w1680:string[][])  [unwired: 1 in]
                  n797 = Insert Into Array(array=w1680, index (row)=0, new element=string[] ["time", "Centroid X", "Centroid Y", "Motor Axis 1", "Motor Axis 2"] ("new element/subarray 2")) -> (w1662:string[][])  [unwired: 1 in]
                  n798 = call-poly <vilib>:"Write To Spreadsheet File.vi"("2D data"=w1662, "file path (dialog if empty)"=w1649) -> ()  [unwired: 6 in, 1 out]
                }
                frame True {
                }
              }
            }
            n799 = call <vilib>:"Add State(s) to Queue__jki_lib_state_machine.vi"("State(s) in (\"\")"=w1645) -> ("States Out"=w1644:string)  [unwired: 14 in]
          }
          frame Enabled {
          }
        }
        n800 = property on="Save Stats" class="Bool (strict)"("Value"=FALSE ("Save Stats")) -> ()  [unwired: 2 in, 2 out]
      }
      frame "tdms" {
        w1706 = 21600.0 ("new tdms")
        # "Your code here.\n(You can make a copy of, or modify, this frame)"
        n801 = Unbundle By Name(w1713) -> ("active cams"=w1699:string[], "tdms ref"=w1696:refnum<k34>, "Offset X"=w1712:dbl[][], "Offset Y"=w1711:dbl[][], "Motor positions.Positions x"=w1694:dbl[], "Motor positions.Positions y"=w1693:dbl[])
        n802 = for {
          tunnel: w1712 -> [w1756]
          tunnel: w1711 -> [w1755]
          tunnel: w1699 -> [w1728] mode=indexing
          tunnel: w1696 -> [w1729]
          tunnel: w1715 -> [w1723]
          tunnel: [w1732] -> w1714
          tunnel: w1694 -> [w1722]
          tunnel: w1693 -> [w1720]
          i -> [w1719]
          n803 = Index Array(array=w1756, index (row)=w1719) -> (element=w1754:dbl[])  [unwired: 1 in]
          n804 = Index Array(array=w1755, index (row)=w1719) -> (element=w1753:dbl[])  [unwired: 1 in]
          n805 = Reverse 1D Array(array=w1753) -> (reversed array=w1751:dbl[])
          n806 = Reverse 1D Array(array=w1754) -> (reversed array=w1752:dbl[])
          n807 = Index Array(array=w1752) -> (element=w1750:dbl)  [unwired: 1 in]
          n808 = Index Array(array=w1751) -> (element=w1749:dbl)  [unwired: 1 in]
          n809 = Index Array(array=w1720, index=w1719) -> (element=w1718:dbl)
          n810 = Index Array(array=w1722, index=w1719) -> (element=w1721:dbl)
          n811 = Build Array(w1750) -> (w1731:dbl[])
          n812 = Build Array(w1749) -> (w1744:dbl[])
          n813 = Get Date/Time In Seconds() -> (seconds since 1Jan1904=w1730:timestamp)
          n814 = Build Array(w1730) -> (w1726:timestamp[])
          n815 = Build Array(w1721) -> (w1738:dbl[])
          n816 = TDMS Write(0:w1729, 5:w1728, 7:"time", 9:w1726, 11:w1723) -> (4:w1725:refnum<k34>, 15:w1724:errorcluster)  [unwired: 1 in, 2 out]
          n817 = Build Array(w1718) -> (w1733:dbl[])
          n818 = TDMS Write(0:w1725, 5:w1728, 7:"centroid X", 9:w1731, 11:w1724) -> (4:w1747:refnum<k34>, 6:w1746:string, 15:w1745:errorcluster)  [unwired: 1 in, 1 out]
          n819 = TDMS Write(0:w1747, 5:w1746, 7:"centroid Y", 9:w1744, 11:w1745) -> (4:w1741:refnum<k34>, 6:w1740:string, 15:w1742:errorcluster)  [unwired: 1 in, 1 out]
          n820 = TDMS Write(0:w1741, 5:w1740, 7:"Motor Axis 1", 9:w1738, 11:w1742) -> (4:w1737:refnum<k34>, 6:w1736:string, 15:w1734:errorcluster)  [unwired: 1 in, 1 out]
          n821 = TDMS Write(0:w1737, 5:w1736, 7:"Motor Axis 2", 9:w1733, 11:w1734) -> (15:w1732:errorcluster)  [unwired: 1 in, 3 out]
        }
        n822 = property on="millisecond timer value" class="DigNum (strict)"() -> ("Value"=w1698:u32)  [unwired: 2 in, 2 out]
        n823 = Tick Count (ms)() -> (millisecond timer value=w1697:u32)
        n824 = Unbundle By Name(w1713) -> ()  [unwired: 1 out]
        n825 = Subtract(x=w1697, y=w1698) -> (x-y=w1701:u32)
        n826 = Divide(x=w1701, y=u32 1000) -> (x/y=w1703:dbl)
        n827 = Quotient & Remainder(x=w1703, y=w1706) -> (x-y*floor(x/y)=w1704:dbl)  [unwired: 1 out]
        n828 = Subtract(x=w1706, y=20.0) -> (x-y=w1708:dbl)
        n829 = Greater?(x=w1704, y=w1708) -> (0:w1705:bool)
        n830 = Select(t="newtdms", s=w1705, f="") -> (s? t:f=w1700:string)
        n831 = call <vilib>:"Add State(s) to Queue__jki_lib_state_machine.vi"("State(s) in (\"\")"=w1717, "State(s) at Back (\"\")"=w1700) -> ("States Out"=w1716:string)  [unwired: 13 in]
      }
      frame "Reset History" {
        # "Your code here.\n(You can make a copy of, or modify, this frame)"
        n832 = for {
          N: 1 -> [_]
          shift-right: [w1767] -> w1759
          shift-left: timestamp[][] [] ("Time") -> [w1769]
          n833 = for {
            N: 12 -> [_]
            tunnel: w1769 -> [w1772] mode=indexing
            tunnel: [w1770] -> w1767 mode=indexing
            n834 = Get Date/Time In Seconds() -> (seconds since 1Jan1904=w1771:timestamp)
            n835 = Build Array (concatenate)(w1772, w1771) -> (w1770:timestamp[])
          }
        }
        n836 = local read "Offset X"() -> (w1758:dbl[][])
        n837 = Bundle By Name(cluster=w1763, "Offset X"=w1758, "Offset Y"=w1758, "Time"=w1759, "Motor X"=w1758) -> (w1762:T35)
        n838 = call <vilib>:"Add State(s) to Queue__jki_lib_state_machine.vi"("State(s) in (\"\")"=w1766) -> ("States Out"=w1765:string)  [unwired: 14 in]
      }
      frame "New Category: 2" {
        # "Your code here.\n(You can make a copy of, or modify, this frame)"
        n839 = call <vilib>:"Add State(s) to Queue__jki_lib_state_machine.vi"("State(s) in (\"\")"=w1777) -> ("States Out"=w1776:string)  [unwired: 14 in]
      }
      frame "stats" {
        # "Your code here.\n(You can make a copy of, or modify, this frame)"
        n840 = Unbundle By Name(w1793) -> ("Offset X"=w1784:dbl[][], "Offset Y"=w1783:dbl[][], "Time"=w1782:timestamp[][], "Motor X"=w1781:dbl[][], "Motor Y"=w1780:dbl[][], "tdms ref"=w1788:refnum<k34>)
        n841 = TDMS List Contents(4:w1787, 7:w1788) -> (0:w1779:errorcluster, 2:w1791:string[], 3:w1790:refnum<k34>)  [unwired: 1 in, 1 out]
        n842 = call <vilib>:"ClearError.vi"("error in (no error)"=w1779) -> ("error out"=w1789:errorcluster)
        n843 = for {
          tunnel: w1789 -> [w1838]
          tunnel: [w1824] -> w1785 mode=indexing
          tunnel: [w1823] -> w1786
          tunnel: [w1822] -> _
          tunnel: w1790 -> [w1821]
          tunnel: w1791 -> [w1820] mode=indexing
          w1839 = dbl[] [] ("appended array")
          n844 = TDMS Read(0:w1821, 5:w1820, 7:"time", 11:w1838, 12:timestamp[] [] ("appended array")) -> (4:w1853:refnum<k34>, 6:w1849:string, 10:w1830:timestamp[], 15:w1837:errorcluster)  [unwired: 3 in, 2 out]
          n845 = TDMS Read(0:w1853, 5:w1849, 7:"centroid X", 11:w1837, 12:w1839) -> (4:w1852:refnum<k34>, 6:w1848:string, 10:w1833:dbl[], 15:w1836:errorcluster)  [unwired: 3 in, 2 out]
          n846 = TDMS Read(0:w1852, 5:w1848, 7:"centroid Y", 11:w1836, 12:w1839) -> (4:w1851:refnum<k34>, 6:w1847:string, 10:w1832:dbl[], 15:w1835:errorcluster)  [unwired: 3 in, 2 out]
          n847 = TDMS Read(0:w1851, 5:w1847, 7:"Motor Axis 1", 11:w1835, 12:w1839) -> (4:w1850:refnum<k34>, 6:w1846:string, 10:w1831:dbl[], 15:w1834:errorcluster)  [unwired: 3 in, 2 out]
          n848 = TDMS Read(0:w1850, 5:w1846, 7:"Motor Axis 2", 11:w1834, 12:w1839) -> (4:w1822:refnum<k34>, 10:w1829:dbl[], 15:w1823:errorcluster)  [unwired: 3 in, 3 out]
          n849 = Bundle("appended array"=w1830, "appended array"=w1833) -> (w1828:T56)  [unwired: 1 in]
          n850 = Bundle("appended array"=w1830, "appended array"=w1832) -> (w1827:T56)  [unwired: 1 in]
          n851 = Bundle("appended array"=w1830, "appended array"=w1831) -> (w1826:T56)  [unwired: 1 in]
          n852 = Bundle("appended array"=w1830, "appended array"=w1829) -> (w1825:T56)  [unwired: 1 in]
          n853 = Build Array(w1828, w1827, w1826, w1825) -> (w1824:T57)
        }
        n854 = disable-structure shown="Disabled" {
          disable-tunnel: w1792 -> [w1803 _]
          disable-tunnel: w1784 -> [w1802 _]
          disable-tunnel: w1783 -> [w1801 _]
          disable-tunnel: w1782 -> [w1800 _]
          disable-tunnel: w1781 -> [w1799 _]
          disable-tunnel: w1780 -> [w1798 _]
          frame Disabled {
            n855 = for {
              tunnel: w1803 -> [_] mode=indexing
              tunnel: w1802 -> [w1813]
              tunnel: w1801 -> [w1812]
              tunnel: w1800 -> [w1811]
              tunnel: w1799 -> [w1807]
              tunnel: w1798 -> [w1806]
              tunnel: [w1815] -> _ mode=indexing
              i -> [w1814]
              n856 = Index Array(array=w1812, index (row)=w1814) -> (element=w1808:dbl[])  [unwired: 1 in]
              n857 = Index Array(array=w1807, index (row)=w1814) -> (element=w1805:dbl[])  [unwired: 1 in]
              n858 = Index Array(array=w1806, index (row)=w1814) -> (element=w1804:dbl[])  [unwired: 1 in]
              n859 = Index Array(array=w1813, index (row)=w1814) -> (element=w1809:dbl[])  [unwired: 1 in]
              n860 = Index Array(array=w1811, index (row)=w1814) -> (element=w1810:timestamp[])  [unwired: 1 in]
              n861 = Bundle("Time"=w1810, "Motor X"=w1805) -> (w1818:cluster{"Time":timestamp[], "Motor X":dbl[]})  [unwired: 1 in]
              n862 = Bundle("Time"=w1810, "Motor Y"=w1804) -> (w1819:cluster{"Time":timestamp[], "Motor Y":dbl[]})  [unwired: 1 in]
              n863 = Bundle("Time"=w1810, "Offset X"=w1809) -> (w1817:cluster{"Time":timestamp[], "Offset X":dbl[]})  [unwired: 1 in]
              n864 = Bundle("Time"=w1810, "Offset Y"=w1808) -> (w1816:cluster{"Time":timestamp[], "Offset Y":dbl[]})  [unwired: 1 in]
              n865 = Build Array(w1816, w1817, w1818, w1819) -> (w1815:cluster{"Time":timestamp[], "Motor Y":dbl[]}[])
            }
          }
          frame Enabled {
          }
        }
        n866 = Index Array(array=w1785, index (row)="Cam# history") -> (element=→"CCD 1":T57)  [unwired: 1 in]
        n867 = call <vilib>:"Add State(s) to Queue__jki_lib_state_machine.vi"("State(s) in (\"\")"=w1797) -> ("States Out"=w1796:string)  [unwired: 14 in]
      }
      frame "newtdms" {
        n868 = Unbundle By Name(w1892) -> ("tdms ref"=w1885:refnum<k34>, "active cams"=w1880:string[])
        n869 = Empty String/Path?(string/path="tdms root") -> (empty?=w1857:bool)
        n870 = Select(t=path "c:/BeamPointing" ("tdms root"), s=w1857, f="tdms root") -> (s? t:f=w1854:path)
        n871 = TDMS Close(8:w1890, 11:w1885) -> (0:w1879:errorcluster)  [unwired: 1 out]
        n872 = local read "config path"() -> (w1861:string)
        n873 = call <vilib>:"Clear Errors.vi"("error in (no error)"=w1879) -> ("error out"=w1868:errorcluster)  [unwired: 5 in, 1 out]
        n874 = Get Date/Time In Seconds() -> (seconds since 1Jan1904=w1873:timestamp)
        n875 = call-poly <userlib>:"Strip Path Extension__ogtk.vi"("path"=w1861) -> ("root"=w1860:string)  [unwired: 1 out]
        n876 = property on="new tdms" class="Bool (strict)"("Value"=FALSE ("new tdms")) -> ()  [unwired: 2 in, 2 out]
        n877 = Format Date/Time String(time format string (%c)="%Y%m%d", seconds (now)=w1873) -> (date/time string=w1874:string)  [unwired: 1 in]
        n878 = Format Date/Time String(time format string (%c)="%Y%m%d%H%M", seconds (now)=w1873) -> (date/time string=w1871:string)  [unwired: 1 in]
        n879 = String To Path(string=w1860) -> (path=w1859:path)
        n880 = Strip Path(path=w1859) -> (name=w1858:string)  [unwired: 1 out]
        n881 = Build Path(base path=w1854, name or relative path=w1874) -> (appended path=w1875:path)
        n882 = Concatenate Strings(w1871, w1858, ".tdms" ("string")) -> (w1870:string)
        n883 = String To Path(string=w1870) -> (path=w1866:path)
        n884 = call <vilib>:"Check if File or Folder Exists.vi"("error in (no error)"=w1868, "path"=w1875) -> ("error out"=w1878:errorcluster, "file or folder exists?"=w1876:bool, "dup path"=w1877:path)  [unwired: 7 in]
        n885 = case shown="False" w1876 {
          tunnel: w1877 -> [w1898 w1900]
          tunnel: [w1897 w1900] -> w1865
          tunnel: w1878 -> [w1896 w1899]
          tunnel: [w1895 w1899] -> w1867
          frame False {
            n886 = Create Folder(path (use dialog)=w1898, error in=w1896) -> (created path=w1897:path, error out=w1895:errorcluster)  [unwired: 1 in, 1 out]
          }
          frame True {
          }
        }
        n887 = call <vilib>:"Add State(s) to Queue__jki_lib_state_machine.vi"("State(s) in (\"\")"=w1894) -> ("States Out"=w1893:string)  [unwired: 14 in]
        n888 = Build Path(base path=w1865, name or relative path=w1866) -> (appended path=w1886:path)
        n889 = TDMS Open(6:FALSE ("disable buffering (T)"), 7:enum16{"1.0", "2.0"}."2.0" ("file format version (2.0)"), 8:w1867, 10:T31."create or replace" ("operation"), 11:w1886) -> (0:w1883:errorcluster, 3:w1882:refnum<k34>)  [unwired: 2 in]
        n890 = call "TDMSbuffersize.vi"("error in (no error)"=w1883, "group names"=w1880, "Data Value Reference in"=w1882) -> ("error out"=w1863:errorcluster, "Data Value Reference out"=w1881:refnum<k34>)  [unwired: 7 in]
        n891 = Bundle By Name(cluster=w1892, "tdms ref"=w1881) -> (w1891:T35)
      }
      frame "Center" {
        # "Your code here.\n(You can make a copy of, or modify, this frame)"
        n892 = control-ref of="image::1"() -> (w1916:refnum<vi>)
        n893 = control-ref of="image::2"() -> (w1915:refnum<vi>)
        n894 = control-ref of="image::3"() -> (w1914:refnum<vi>)
        n895 = control-ref of="image::4"() -> (w1913:refnum<vi>)
        n896 = control-ref of="image::5"() -> (w1912:refnum<vi>)
        n897 = control-ref of="image::6"() -> (w1911:refnum<vi>)
        n898 = control-ref of="image::7"() -> (w1910:refnum<vi>)
        n899 = control-ref of="image::8"() -> (w1909:refnum<vi>)
        n900 = control-ref of="image::9"() -> (w1908:refnum<vi>)
        n901 = control-ref of="image::10"() -> (w1907:refnum<vi>)
        n902 = control-ref of="image::11"() -> (w1906:refnum<vi>)
        n903 = control-ref of="image::12"() -> (w1905:refnum<vi>)
        n904 = for {
          tunnel: [w1925] -> w1904 mode=indexing
          tunnel: w1903 -> [w1924] mode=indexing
          n905 = Unbundle By Name(w1924) -> ("Target.X::12"=w1923:refnum<vi>, "Target.Y::12"=w1922:refnum<vi>)
          n906 = property class="DigNum (strict)"(reference=w1923) -> ("Value"=w1926:dbl)  [unwired: 1 in, 2 out]
          n907 = property class="DigNum (strict)"(reference=w1922) -> ("Value"=w1927:dbl)  [unwired: 1 in, 2 out]
          n908 = Bundle("Value"=w1926, "Value"=w1927) -> (w1925:cluster{"Value":dbl, "Value":dbl})  [unwired: 1 in]
        }
        n909 = call <vilib>:"Add State(s) to Queue__jki_lib_state_machine.vi"("State(s) in (\"\")"=w1921) -> ("States Out"=w1920:string)  [unwired: 14 in]
        n910 = Build Array(w1916, w1915, w1914, w1913, w1912, w1911, w1910, w1909, w1908, w1907, w1906, w1905) -> (w1917:refnum<vi>[])
        n911 = for {
          tunnel: w1917 -> [w1929] mode=indexing
          tunnel: w1904 -> [w1928] mode=indexing
          n912 = property class="ImageControl"(reference=w1929, "Image Center Position"=w1928) -> ()  [unwired: 1 in, 2 out]
        }
        n913 = property on="Center" class="Bool (strict)"("Value"=FALSE ("Center")) -> ()  [unwired: 2 in, 2 out]
      }
      frame "ImgToAvg" {
        n914 = Bundle By Name(cluster=w1939, "Detection.img to avg"="img to avg") -> (w1938:T35)
        n915 = call <vilib>:"Build State String with Arguments__jki_lib_state_machine.vi"("Arguments (\"\")"="T" ("Arguments (\"\")"), "State"=" Device Ini") -> ("State with Arguments"=w1932:string)  [unwired: 4 in]
        n916 = call <vilib>:"Add State(s) to Queue__jki_lib_state_machine.vi"("State(s) in Front (\"\")"=w1932, "State(s) in (\"\")"=w1937) -> ("States Out"=w1936:string)  [unwired: 13 in]
      }
      frame "history" {
        # "Your code here.\n(You can make a copy of, or modify, this frame)"
        n917 = Unbundle By Name(w1950) -> ("Offset X"=w1956:dbl[][], "Offset Y"=w1955:dbl[][], "Mean Centroid X"=w1954:dbl[][], "Mean Centroid Y"=w1953:dbl[][], "Motor X"=w1952:dbl[][], "Motor Y"=w1951:dbl[][], "Time"=w1942:timestamp[][])
        n918 = for {
          tunnel: w1956 -> [w1974] mode=indexing
          tunnel: w1955 -> [w1972] mode=indexing
          tunnel: w1954 -> [w1971] mode=indexing
          tunnel: w1953 -> [w1970] mode=indexing
          tunnel: w1952 -> [w1969] mode=indexing
          tunnel: w1951 -> [w1968] mode=indexing
          tunnel: [w1973] -> w1948 mode=indexing
          tunnel: [w1967] -> w1947 mode=indexing
          tunnel: [w1963] -> w1946 mode=indexing
          tunnel: [w1966] -> w1945 mode=indexing
          tunnel: [w1965] -> w1944 mode=indexing
          tunnel: [w1964] -> w1943 mode=indexing
          tunnel: w1942 -> [w1962] mode=indexing
          tunnel: [w1960] -> w1941 mode=indexing
          w1961 = 0
          n919 = Delete From Array(array=w1969, index=w1961) -> (array with subset deleted=w1965:dbl[])  [unwired: 1 in, 1 out]
          n920 = Delete From Array(array=w1968, index=w1961) -> (array with subset deleted=w1964:dbl[])  [unwired: 1 in, 1 out]
          n921 = Delete From Array(array=w1962, index=w1961) -> (array with subset deleted=w1960:timestamp[])  [unwired: 1 in, 1 out]
          n922 = Delete From Array(array=w1971, index=w1961) -> (array with subset deleted=w1963:dbl[])  [unwired: 1 in, 1 out]
          n923 = Delete From Array(array=w1970, index=w1961) -> (array with subset deleted=w1966:dbl[])  [unwired: 1 in, 1 out]
          n924 = Delete From Array(array=w1972, index=w1961) -> (array with subset deleted=w1967:dbl[])  [unwired: 1 in, 1 out]
          n925 = Delete From Array(array=w1974, index=w1961) -> (array with subset deleted=w1973:dbl[])  [unwired: 1 in, 1 out]
        }
        n926 = call <vilib>:"Add State(s) to Queue__jki_lib_state_machine.vi"("State(s) in (\"\")"=w1959) -> ("States Out"=w1958:string)  [unwired: 14 in]
        n927 = Bundle By Name(cluster=w1950, "Offset X"=w1948, "Offset Y"=w1947, "Mean Centroid X"=w1946, "Mean Centroid Y"=w1945, "Motor X"=w1944, "Motor Y"=w1943, "Time"=w1941) -> (w1949:T35)
      }
    }
    "Prev State" <- w49
    n928 = property on="Box" class="Arr (strict)"() -> ("Value"=w57:T2)  [unwired: 2 in, 2 out]
    n929 = for {
      tunnel: w58 -> [w101]
      tunnel: w51 -> [w110]
      tunnel: w55 -> [w108] mode=indexing
      tunnel: w57 -> [w69] mode=indexing
      tunnel: w54 -> [w99]
      tunnel: w53 -> [w98]
      tunnel: w52 -> [w80]
      i -> [w79]
      w94 = T58 {"Draw"=TRUE, "Target"={"x"=20.0, "y"=20.0}, "Size"={"x"=20.0, "y"=20.0}, "Angle"=1250067.0, "Color"=1250067, "Thickness"=0, "CrosshairLabel"=""} ("Crosshair")
      w88 = T59 {"Left"=0, "Top"=0, "Right"=0, "Bottom"=0} ("Bounding Rectangle")
      n930 = call-poly <userlib>:"Filter 1D Array__ogtk.vi"("items to filter"=w108, "array"=w110) -> ("filtered item indices"=w111:i32[])  [unwired: 4 in, 1 out]
      n931 = Index Array(array=w111) -> (element=w100:i32)  [unwired: 1 in]
      n932 = Index Array(array=w80, index (row)=w79) -> (element=w77:dbl[])  [unwired: 1 in]
      n933 = Index Array(array=w99, index (row)=w79) -> (element=w87:dbl[])  [unwired: 1 in]
      n934 = Index Array(array=w98, index (row)=w79) -> (element=w85:dbl[])  [unwired: 1 in]
      n935 = Index Array(array=w101, index=w100) -> (element=w109:T20)
      n936 = Reverse 1D Array(array=w77) -> (reversed array=w76:dbl[])
      n937 = Unbundle By Name(w109) -> ("Target.X::12"=w113:refnum<vi>, "Target.Y::12"=w112:refnum<vi>)
      n938 = Reverse 1D Array(array=w87) -> (reversed array=w86:dbl[])
      n939 = Reverse 1D Array(array=w85) -> (reversed array=w84:dbl[])
      n940 = Index Array(array=w76) -> (element=w74:dbl)  [unwired: 1 in]
      n941 = Square Root(x=w74) -> (sqrt(x)=w73:dbl)
      n942 = Index Array(array=w84) -> (element=w81:dbl)  [unwired: 1 in]
      n943 = Index Array(array=w86) -> (element=w82:dbl)  [unwired: 1 in]
      n944 = Divide(x=w73, y=2.0) -> (x/y=w71:dbl)
      n945 = property class="DigNum (strict)"(reference=w113) -> ("Value"=w105:dbl)  [unwired: 1 in, 2 out]
      n946 = property class="DigNum (strict)"(reference=w112) -> ("Value"=w104:dbl)  [unwired: 1 in, 2 out]
      n947 = Bundle(cluster=cluster{"xhair size":dbl, "xhair size 2":dbl} {"xhair size"=25.0, "xhair size 2"=25.0} ("size"), "xhair size"=w71, "xhair size 2"=w71) -> (w75:cluster{"xhair size":dbl, "xhair size 2":dbl})
      n948 = Bundle By Name(cluster=w94, "Draw"=TRUE, "Target.x"=w105, "Target.y"=w104, "Size"=w75, "Color"=u32 16774656, "Angle"=0.0, "Thickness"=u8 1) -> (w107:T58)
      n949 = call "draw crosshair imaq.vi"("clear overlay"=TRUE, "Crosshair"=w107, "Bounding Rectangle"=w88, "image in"=w108) -> ("error out"=w91:errorcluster, "image out"=w90:T5)  [unwired: 6 in]
      n950 = Bundle By Name(cluster=w94, "Draw"=TRUE, "Target.x"=w82, "Target.y"=w81, "Size"=w75, "Color"=u32 8322834, "Angle"=0.0, "Thickness"=u8 1) -> (w92:T58)
      n951 = case shown="True" "average centroid" {
        tunnel: w92 -> [_ w118]
        tunnel: w91 -> [_ w123]
        tunnel: w90 -> [w115 w122]
        tunnel: w88 -> [_ w121]
        tunnel: w69 -> [w116 _]
        tunnel: [w114 w120] -> w68
        frame False {
          n952 = call "draw box imaq.vi"("Color"=u32 1244928, "Rectangle"=w116, "image in"=w115) -> ("error out"=w114:errorcluster)  [unwired: 7 in, 1 out]
        }
        frame True {
          n953 = call "draw crosshair imaq.vi"("clear overlay"=FALSE, "error in (no error)"=w123, "Crosshair"=w118, "Bounding Rectangle"=w121, "image in"=w122) -> ("error out"=w120:errorcluster)  [unwired: 5 in, 1 out]
        }
      }
      "error out 3" <- w68
    }
  }
  n954 = call <userlib>:"Fit VI window to Largest Dec__ogtk.vi"() -> ()  [unwired: 6 in, 2 out]
  n955 = disable-structure shown="Disabled" {
    frame Disabled {
      # "GetMotorPositions"
      # "get all motor positions"
      n956 = call <userlib>:"Tick Count (ms)__ogtk.vi"() -> ("millisecond timer value"=w1983:u32)  [unwired: 10 in, 1 out]
      n957 = Unbundle By Name(w1984) -> ("dev var alias arrays"=w1976)
      n958 = Unbundle By Name(w1976) -> ("dev variable alias Motors X"=w1975, "dev variable alias Motors Y"=w1979)
      n959 = for {
        tunnel: w1979 -> [w1992]
        tunnel: w1975 -> [w1991]
        tunnel: [w1987] -> w1977 mode=indexing
        tunnel: [w1986] -> w1978 mode=indexing
        tunnel: w1979 -> [_]
        tunnel: [errorcluster {"status"=FALSE, "code"=0, "source"=""} ("error out")] -> w1980
        i -> [w1988]
        n960 = call "Beampointing get set motor position.vi"("Active CCD"=w1988, "get or set"=enum16{"get", "set"}."get", "dev variable alias Motors X"=w1991) -> ("Actual Position"=w1987:dbl)  [unwired: 7 in, 1 out]
        n961 = call "Beampointing get set motor position.vi"("Active CCD"=w1988, "get or set"=enum16{"get", "set"}."get", "dev variable alias Motors X"=w1992) -> ("Actual Position"=w1986:dbl)  [unwired: 7 in, 1 out]
      }
      n962 = Bundle By Name("Positions x"=w1977, "Positions y"=w1978) -> (w1984:cluster{})  [unwired: 1 out]
      n963 = call <userlib>:"Tick Count (ms)__ogtk.vi"("error in (no error)"=w1980) -> ("millisecond timer value"=w1981:u32)  [unwired: 9 in, 1 out]
      n964 = Subtract(x=w1981, y=w1983) -> (x-y=→"get pos time":u32)
    }
    frame Enabled {
    }
  }
  n965 = Unbundle By Name(w17) -> ("tdms ref"=w16:refnum<k34>)
  n966 = for {
    tunnel: w45 -> [w1995] mode=indexing
    tunnel: w44 -> [w1994]
    tunnel: [w1993] -> w15
    n967 = call "IMAQ Dispose"("Image"=w1995, "error in (no error)"=w1994) -> ("error out"=w1993:errorcluster)  [unwired: 4 in]
  }
  n968 = TDMS Close(8:w15, 11:w16) -> (0:→"error out 2":errorcluster)  [unwired: 1 out]
